vi "COD主界面（列队使用）.vi"() -> (8 "多列列表框":i32(listbox))   [LabVIEW 2016, in "斯坦道CODMn.lvlib"]
uses:
  <vilib>/Analysis/6fits.llb/Curve Fitting Criteria.ctl
  <vilib>/Utility/miscctls.llb/LVPointTypeDef.ctl
  <vilib>/Utility/config.llb/Read Key (I32).vi
  <vilib>/Utility/config.llb/Read Key (Double).vi
  <vilib>/Utility/config.llb/Read Key (Boolean).vi
  <vilib>/Utility/config.llb/Write Key (Double).vi
  <vilib>/Utility/config.llb/Write Key (Boolean).vi
  <vilib>/Utility/config.llb/Write Key (I32).vi
  <vilib>/Waveform/WDTFileIO.llb/Read Waveform from File.vi
  <vilib>/ptbypt/NI_PtbyPt.lvlib
  <vilib>/Utility/config.llb/NI_LVConfig.lvlib
  <vilib>/Analysis/NI_AALPro.lvlib
panel:
  in  "常规版/认证版":enum16{"常规版", "认证版"}(ring)
  in  "释放串口":bool
  in  "打开串口":bool
  in  "保存参数":dbl[](array[numeric])
  out "报警数字":i16
  out "CODMn工作状态":T1(ring)
  out "ORP-K":string
  out "ORP-B":string
  out "ORP-A":string
  out "x = y?":bool
  out "稀释倍数解释":string
  in  "CODMn跨度量程选择":enum32{"H", "L", "AUTO"}(ring)=enum."AUTO"
  in  "跨度液浓度":dbl
  in  "水样":dbl
  in  "蒸馏水":dbl
  in  "标液":dbl
  in  "质控样":dbl
  in  "加标回收":dbl
  in  "草酸钠":dbl
  in  "高锰酸钾":dbl
  in  "硫酸":dbl
  out "量程解释说明":string
  in  "高切低阈值:":dbl
  in  "低切高阈值:":dbl
  in  "自动切换量程:":enum16{"关闭", "自动切换测一次", "自动切换测两次"}(ring)
  in  "修正系数":dbl
  in  "标准液浓度":dbl
  in  "温度":dbl
  in  "恒温时间":dbl
  in  "基本量程":enum16{"L", "H"}(ring)
  in  "CODMn零点核查选择":enum16{"零点核查走纯水管", "零点核查走质控管"}(ring)
  in  "锁定按钮":bool
  in  "低量程稀释倍数:":i8=1
  out "切换量程连续测两次":bool
  in  "高量程稀释倍数:":i8=2
  in  "一键写入":bool
  in  "测量模式(公式)":u16(ring)=1 items=["水样测试"=1, "标样核查"=2, "零点核查"=3, "跨度核查"=4, "空白测试"=5, "平行样"=6, "加标回收"=7]
  out "基本量程(显示)":string
  out "测量模式(显示)":string
  in  "量程切换次数":u8
  out "数据时间":string
  out "断电排液标记":bool
  out "COM":string
  in  "启用5":bool
  in  "校准5":bool
  in  "泵滴定数5":dbl
  in  "浓度5":dbl
  in  "启用4":bool
  in  "校准4":bool
  in  "泵滴定数4":dbl
  in  "浓度4":dbl
  out "波形时间":timestamp
  in  "历史波形":bool
  out "滴定数-ORP值":u16[](array[numeric]) caption="数组"
  in  "关闭 3":bool
  in  "滴定曲线":bool
  out "ORP滴定曲线":u16[](graph)
  out "空白测试标记":bool
  out "跨度核查标记":bool
  out "启动选择 2":u16(ring) items=["水样测试", "标样核查", "零点核查", "跨度核查", "空白测试", "加标回收", "平行样", "校零", "校标"]
  in  "量程选择":enum16{"低量程", "高量程", "0-2量程"}(ring)
  in  "手动控制":bool
  in  "选用水样":enum16{"葡萄糖", "草酸钠"}(ring)
  in  "方程系数":cluster{"X":dbl, "b":dbl, "X^2":dbl} {"X^2" format="%#.6g"; "b" format="%#.6g"; "X" format="%#.6g"}
  out "多项式系数1":dbl[](array[numeric]) caption="多项式系数"
  out "XY图":cluster{"X Values":dbl[], "Y Values":dbl[]}[](graph)
  in  "模型":enum32{"线性", "多项式"}(ring)
  out "启动时间":timestamp format="%<%Y/%m/%d %H:%M:%S>T"
  in  "关闭 2":bool
  out "r^2":dbl format="%.8g"
  out "拟合公式":string
  out "b":dbl format="%#.4g"
  out "K":dbl format="%#.4f"
  out "当前校准":i32
  in  "启用3":bool
  in  "启用2":bool
  in  "启用1":bool
  in  "校准3":bool
  in  "校准2":bool
  in  "校准1":bool
  in  "泵滴定数3":dbl
  in  "泵滴定数2":dbl
  in  "泵滴定数1":dbl
  in  "浓度3":dbl
  in  "浓度2":dbl
  in  "浓度1":dbl
  in  "写入":bool
  out "测量模式数字":i32
  out "零点核查标记":bool
  out "排液故障":bool
  out "进水样超量程":bool
  out "标样核查标记":bool
  out "平行样测量":bool
  out "加标回收测量":bool
  out "质控样测量":bool
  out "待机":bool
  out "校标错误":bool
  out "校零错误":bool
  out "测量错误":bool
  out "草酸钠报警":bool
  out "高锰酸钾报警":bool
  out "加热故障":bool
  out "温控器故障":bool
  out "ORP故障":bool
  out "排液标记":bool
  out "故障标记":bool
  out "校标标记":bool
  out "校零标记":bool
  out "通讯状态":bool
  out "水样测量":bool
  in  "读取":bool
  in  "返回":bool
  in  "校准配置":bool
  in  "零点泵计量数 2":dbl
  in  "标度泵计量数 2":dbl
  out "标度滴定值":dbl
  out "零点滴定值":dbl
  in  "保存":bool
  in  "关闭":bool
  out "测量数据区":T2 {"单位" items=["ug/L", "mg/L", "ppm", "mg/m3", "cm", "ppb", "ug/m3", "%", "nmol/mol", "umol/mol", "MPN/L", "MPN/100ml", "ng/m3", "NTU", "无量纲", "ms/cm", "us/cm", "℃", "mV", "万个/L"]}
  out "仪器时间":timestamp format="%<%Y/%m/%d %H:%M:%S>T"
  out "秒":u16
  out "分":u16
  out "COD浓度（mg/L)":dbl format="%.2g"
  out "进样管":dbl
  out "高锰酸钾":dbl
  out "草酸钠":dbl
  out "硫酸":dbl
  out "ORP显示":dbl
  out "温度":dbl
  out "加热":bool
  out "搅拌":bool
  out "进硫酸":bool
  out "进加标回收样":bool
  out "进质控样":bool
  out "进标液":bool
  out "进蒸馏水":bool
  out "进水样":bool
  out "进草酸钠":bool
  out "进高锰酸钾":bool
  out "定时启动":bool
  in  "启动":bool
  in  "故障清除":bool
  in  "参数配置":bool
  in  "停止":bool
  in  "单步启动":bool
  out "系统时间":timestamp
  in  "时间校准":bool
  out "报警簇":T3
  out "模式（受控）":u16
  # "测量时间："
  # "(水样~加标回收)"
  # "mV"
  # "℃"
  # "注：遇到加热故障和排液故障时仪器不能正常启动，\n必须排查故障并点击报警清除按钮方可运行。"
  # "mg/L"
  # "泵计量参数设置"
  # "基本参数设置"
  # "校零校标结果"
  # "校零结果："
  # "校零滴定值："
  # "加热恒温温度(℃):"
  # "水样："
  # "高锰酸钾："
  # "校标结果："
  # "标度滴定值："
  # "恒温时间(分钟):"
  # "草酸钠："
  # "蒸馏水："
  # "零点泵计量值："
  # "标准液浓度(mg/L):"
  # "硫酸："
  # "标液："
  # "标度泵计量值："
  # "修正系数："
  # "跨度液浓度："
  # "质控样:"
  # "基本量程(L、H)可选:"
  # "跨度量程选择："
  # "加标回收样："
  # "是否启用"
  # "泵滴定数"
  # "浓度"
  # "辅\n助\n计\n算\n区"
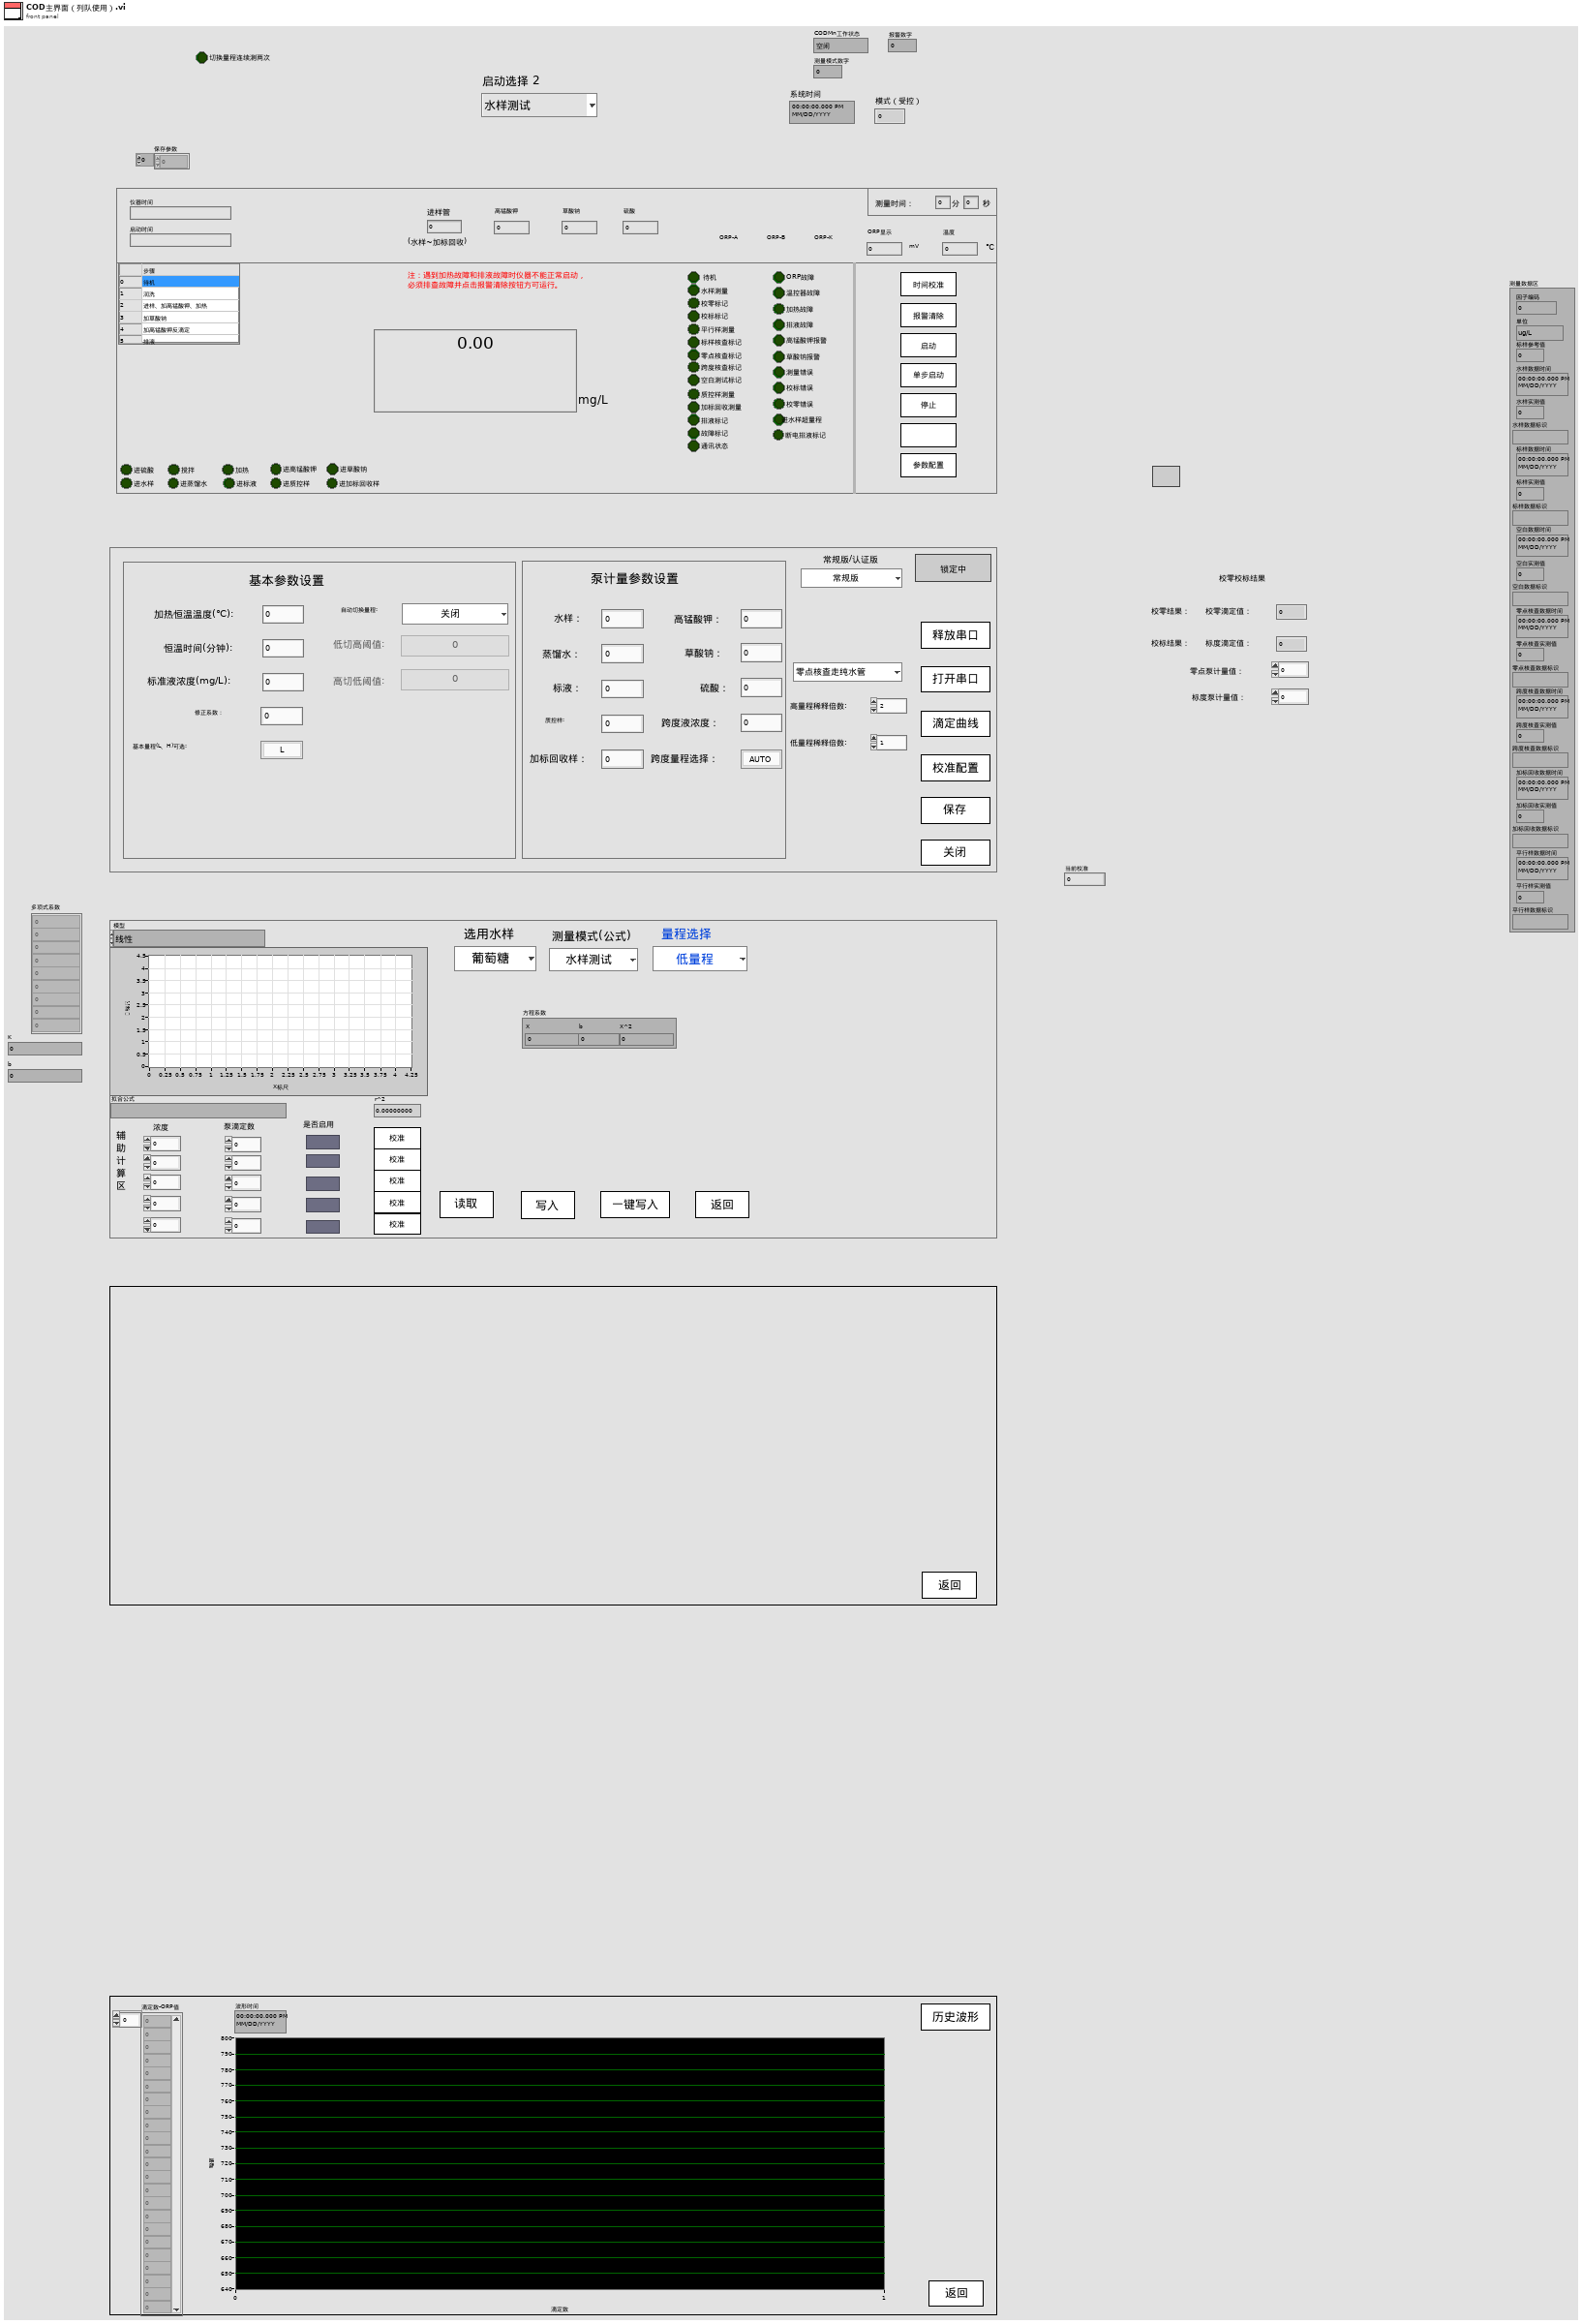
[diagram p1: front panel]
types:
  T1 = enum16{"空闲", "水样测试", "标样核查", "零点核查", "跨度核查", "空白测试", "平行样测试", "质控样", "空白校准", "标样校准", "加标回收"}
  T2 = cluster{"因子编码":u32, "单位":u16, "标样参考值":sgl, "水样数据时间":timestamp, "水样实测值":sgl, "水样数据标识":string, "标样数据时间":timestamp, "标样实测值":sgl, "标样数据标识":string, "空白数据时间":timestamp, "空白实测值":sgl, "空白数据标识":string, "零点核查数据时间":timestamp, "零点核查实测值":sgl, "零点核查数据标识":string, "跨度核查数据时间":timestamp, "跨度核查实测值":sgl, "跨度核查数据标识":string, "加标回收数据时间":timestamp, "加标回收实测值":sgl, "加标回收数据标识":string, "平行样数据时间":timestamp, "平行样实测值":sgl, "平行样数据标识":string}
  T3 = cluster{"ORP故障":bool, "温控器故障":bool, "加热故障":bool, "高锰酸钾报警":bool, "草酸钠报警":bool, "测量错误":bool, "校零错误":bool, "校标错误":bool, " 进水样超量程":bool, "排液阀故障":bool}
  T4 = cluster{"时间":timestamp, "测量模式":string, "数据类型":string, "检测值":sgl, "单位":string, "数据标识":string, "因子编码":string, "标样参考值":sgl, "ORP-A":sgl, "ORP-B":sgl, "ORP-K":sgl, "COD滴定值":sgl, "高锰酸钾滴定数":sgl, "温度":sgl, "量程":sgl}
  T5 = enum8{"Enabled", "Disabled", "Disabled and Grayed Out"}
  T6 = typedef "NI_AALPro.lvlib/Curve Fitting Criteria.ctl" = u16
  T7 = cluster{"数组 2[0]":sgl, "数组 2[1]":sgl, "数组 2[2]":sgl, "数组 2[3]":sgl, "数组 2[4]":sgl, "数组 2[5]":sgl, "数组 2[6]":sgl, "数组 2[7]":sgl, "数组 2[8]":sgl, "数组 2[9]":sgl, "数组 2[10]":sgl, "数组 2[11]":sgl, "数组 2[12]":sgl, "数组 2[13]":sgl, "数组 2[14]":sgl, "数组 2[15]":sgl, "数组 2[16]":sgl, "数组 2[17]":sgl, "数组 2[18]":sgl, "数组 2[19]":sgl, "数组 2[20]":sgl, "数组 2[21]":sgl, "数组 2[22]":sgl, "数组 2[23]":sgl, "数组 2[24]":sgl, "数组 2[25]":sgl, "数组 2[26]":sgl, "数组 2[27]":sgl, "数组 2[28]":sgl, "数组 2[29]":sgl, "数组 2[30]":sgl, "数组 2[31]":sgl, "数组 2[32]":sgl, "数组 2[33]":sgl, "数组 2[34]":sgl, "数组 2[35]":sgl, "数组 2[36]":sgl, "数组 2[37]":sgl, "数组 2[38]":sgl, "数组 2[39]":sgl, "数组 2[40]":sgl, "数组 2[41]":sgl}
  T8 = cluster{"测量模式":enum16{"水样测量", "标样核查", "零点核查", "跨度核查", "空白测试", "加标回收", "平行样", "校零", "校标"}}
  T9 = cluster{"仪器测试类型":enum16{"水样测试", "标样核查", "空白测试", "跨度核查"}, "周期设置类型":enum16{"定点启动", "间隔启动"}, "定时功能启用":bool, "定时间隔":dbl, "24H周期设置":bool[]}
  T10 = typedef "LVDateTimeRec.ctl" = cluster{"秒数的小数部分":dbl, "秒":i32, "分":i32, "时":i32, "日":i32, "月":i32, "年":i32, "天数（周）":i32, "天数（年）":i32, "DST":i32}
  T11 = cluster{"时间标识":timestamp, "设备":string, "日志信息":string}
  T12 = cluster{"时间标识":timestamp, "参数":string, "日志信息":string, "流程参数":string}
  T13 = cluster{"时间标识":timestamp, "设备":string, "日志信息":string, "流程参数":string}
  T14 = typedef "NI_LVConfig.lvlib/Config Data RefNum.ctl" = refnum<k1>
  T15 = typedef "LVPointTypeDef.ctl" = cluster{"Horizontal":i16, "Vertical":i16}
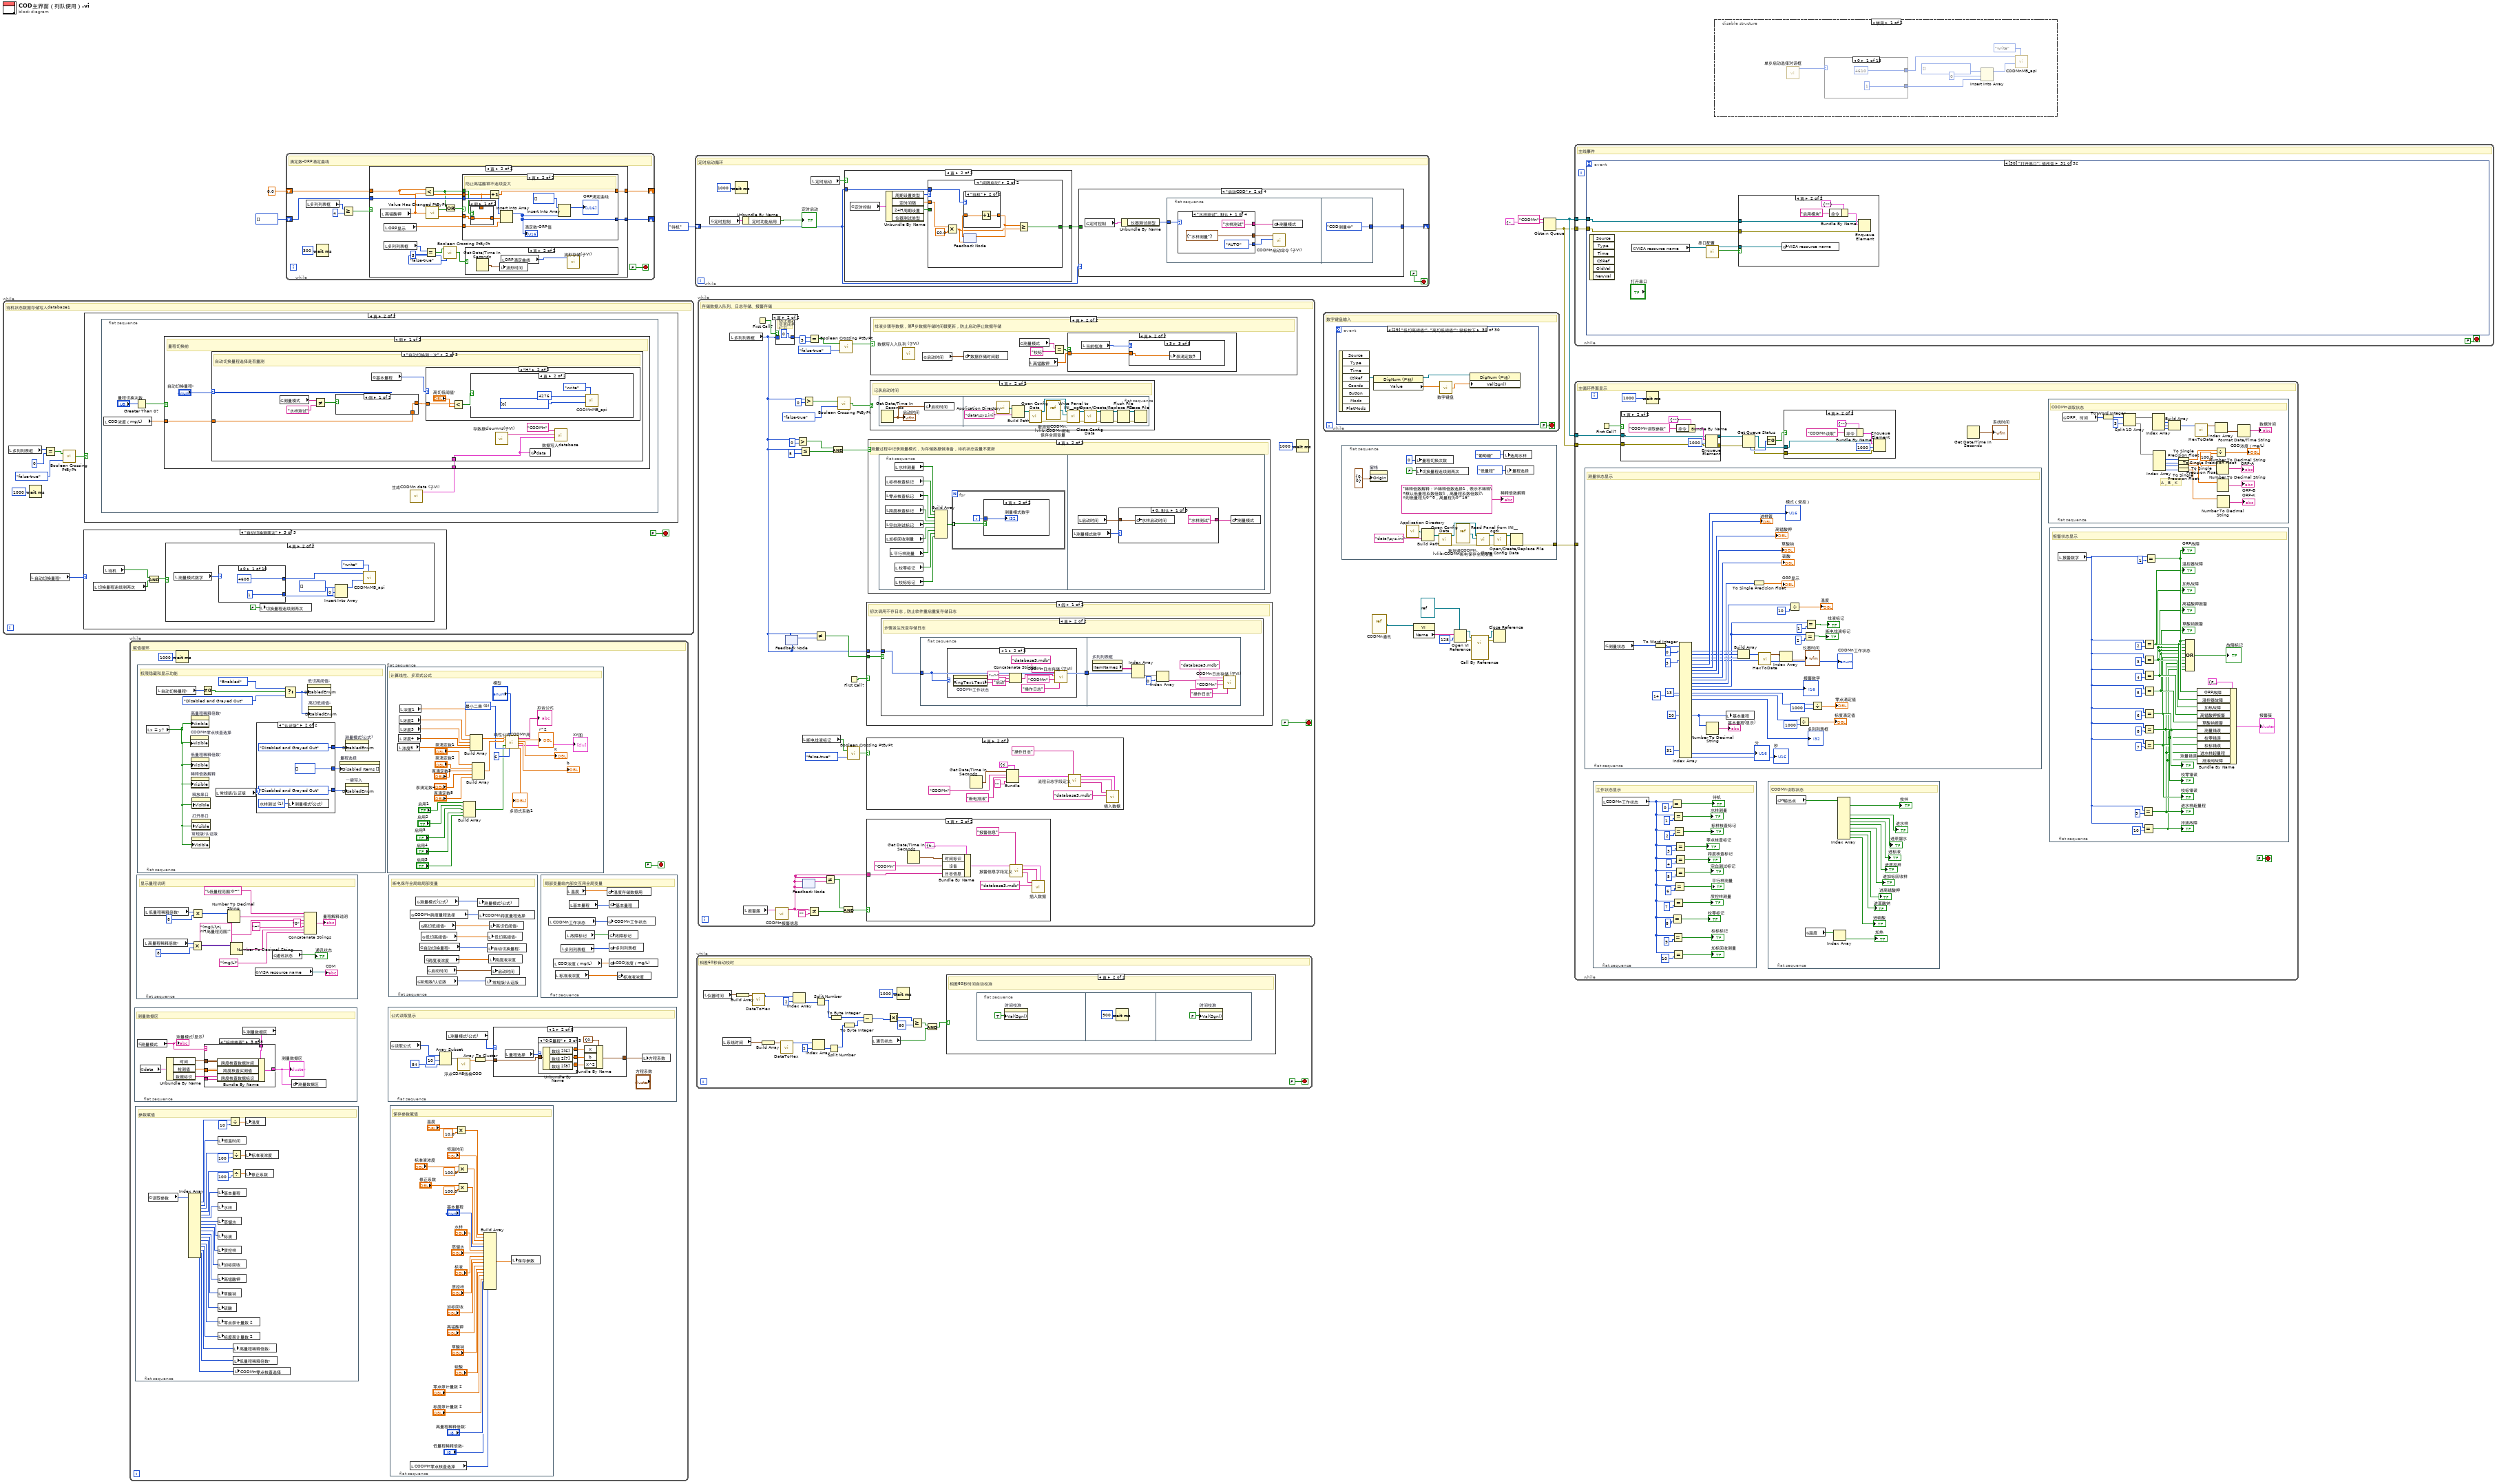
[diagram p0: block diagram]
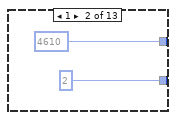
[diagram p2: hidden frame]
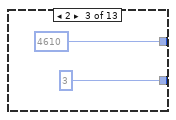
[diagram p3: hidden frame]
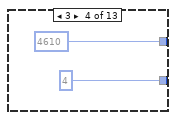
[diagram p4: hidden frame]
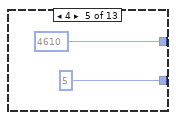
[diagram p5: hidden frame]
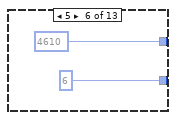
[diagram p6: hidden frame]
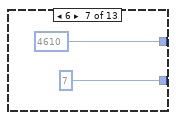
[diagram p7: hidden frame]
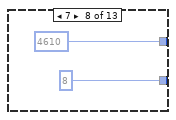
[diagram p8: hidden frame]
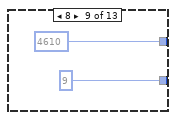
[diagram p9: hidden frame]
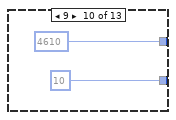
[diagram p10: hidden frame]
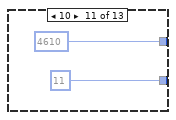
[diagram p11: hidden frame]
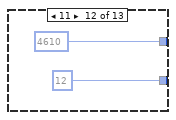
[diagram p12: hidden frame]
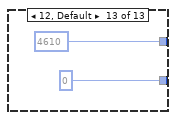
[diagram p13: hidden frame]
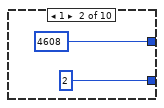
[diagram p19: hidden frame]
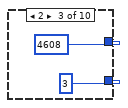
[diagram p20: hidden frame]
diagram:
  n1 = while {
    stop <- FALSE stop-if-true
    # "待机状态数据存储写入database1"
    n2 = local read "多列列表框"() -> (w22:i32)
    n3 = Wait (ms)(milliseconds to wait=u32 1000 ("等待时间（毫秒）")) -> ()  [unwired: 1 out]
    n4 = local read "自动切换量程:"() -> (w17:enum16{"关闭", "自动切换测一次", "自动切换测两次"})
    n5 = Equal?(x=w22, y=0) -> (x = y?=w20:bool)
    n6 = call <vilib>:"Boolean Crossing PtByPt.vi"("direction"=enum16{"either", "false-true", "true-false"}."false-true", "input"=w20) -> ("crossing"=w18:bool)  [unwired: 1 in]
    n7 = case shown="\"自动切换测两次\"" w17 {
      frame "关闭", Default {
      }
      frame "自动切换测一次" {
      }
      frame "自动切换测两次" {
        n8 = local read "切换量程连续测两次"() -> (w26:bool)
        n9 = local read "待机"() -> (w27:bool)
        n10 = Compound Arithmetic op=AND ("复合运算")(w27, w26) -> (w25:bool)
        n11 = case shown="真" w25 {
          frame False {
          }
          frame True {
            n12 = local read "测量模式数字"() -> (w32:i32)
            n13 = case shown="0" w32 {
              tunnel: [u16 4608 ("address") u16 4608 ("address") u16 4608 ("address") u16 4608 ("address") u16 4608 ("address") u16 4608 ("address") u16 4608 ("address") u16 4608 ("address") u16 4608 ("address") u16 4608 ("address")] -> w28
              tunnel: [u16 1 ("address") u16 2 ("address") u16 3 ("address") u16 4 ("address") u16 5 ("address") u16 7 ("address") u16 6 ("address") u16 8 ("address") u16 9 ("address") u16 0 ("address")] -> w35
              frame 0 {
              }
              frame 1 {
              }
              frame 2 {
              }
              frame 3 {
              }
              frame 4 {
              }
              frame 5 {
              }
              frame 6 {
              }
              frame 7 {
              }
              frame 8 {
              }
              frame 9, Default {
              }
            }
            n14 = local write "切换量程连续测两次"(FALSE ("切换量程连续测两次")) -> ()
            n15 = Insert Into Array(array=u16[] [] ("values"), index=0 ("索引"), new element=w35) -> (w29:u16[])
            n16 = call "CODMnMB_api.vi"("STEP"=enum16{"open", "read", "write", "close"}."write", "values"=w29, "starting address"=w28) -> ()  [unwired: 5 in, 4 out]
          }
        }
      }
    }
    n17 = case shown="真" w18 {
      frame False {
      }
      frame True {
        n18 = flat-sequence {
          frame #0 {
            n19 = local read "COD浓度（mg/L)"() -> (w56:dbl)
            n20 = Greater Than 0?(x="量程切换次数") -> (x > 0?=w57:bool)
            n21 = call "生成CODMn data (子VI).vi"() -> ("data"=w59:T4)  [unwired: 11 in]
            n22 = case shown="假" w57 {
              tunnel: w59 -> [w61 w116]
              tunnel: w56 -> [w60 _]
              frame False {
                # "量程切换前"
                n23 = case shown="\"自动切换测一次\"" "自动切换量程:" {
                  tunnel: w61 -> [w63 w68 w92]
                  tunnel: w60 -> [_ w66 w90]
                  frame "关闭", Default {
                    # "关闭自动切换量程"
                    n24 = call "存数据cloumns(子VI).vi"() -> ("数组"=w65:string[])  [unwired: 11 in]
                    n25 = global write "COD读取DATA全局.vi" "data"(w63) -> ()
                    n26 = call "数据写入database.vi"("data"=w63, "columns"=w65, "table"="CODMn") -> ()  [unwired: 8 in, 1 out]
                  }
                  frame "自动切换测一次" {
                    # "自动切换量程选择是否重测"
                    n27 = global read "COD测量模式全局.vi" "测量模式"() -> (w74:string)
                    n28 = Not Equal?(x=w74, y="水样测试") -> (x != y?=w72:bool)
                    n29 = case shown="假" w72 {
                      tunnel: [w75 w76] -> w71
                      tunnel: w66 -> [w75 _]
                      frame False {
                      }
                      frame True {
                        n30 = global read "COD读取DATA全局.vi" "测量数据区"() -> (w77:T2)
                        n31 = Unbundle By Name(w77) -> ("水样实测值"=w76:sgl)
                      }
                    }
                    n32 = global read "COD浓度全局变量.vi" "基本量程"() -> (w67:enum16{"L", "H"})
                    n33 = case shown="\"H\"" w67 {
                      tunnel: w71 -> [w78 w84]
                      frame "L", Default {
                        n34 = Greater?(x=w78, y="低切高阈值:") -> (0:w79:bool)
                        n35 = case shown="假" w79 {
                          frame False {
                          }
                          frame True {
                            n36 = call "CODMnMB_api.vi"("STEP"=enum16{"open", "read", "write", "close"}."write", "values"=u16[] [1], "starting address"=u16 4276) -> ()  [unwired: 5 in, 4 out]
                          }
                        }
                      }
                      frame "H" {
                        n37 = Less?(x=w84, y="高切低阈值:") -> (x < y?=w85:bool)
                        n38 = case shown="真" w85 {
                          frame False {
                          }
                          frame True {
                            n39 = call "CODMnMB_api.vi"("STEP"=enum16{"open", "read", "write", "close"}."write", "values"=u16[] [0], "starting address"=u16 4276) -> ()  [unwired: 5 in, 4 out]
                          }
                        }
                      }
                    }
                    n40 = call "存数据cloumns(子VI).vi"() -> ("数组"=w70:string[])  [unwired: 11 in]
                    n41 = global write "COD读取DATA全局.vi" "data"(w68) -> ()
                    n42 = call "数据写入database.vi"("data"=w68, "columns"=w70, "table"="CODMn") -> ()  [unwired: 8 in, 1 out]
                  }
                  frame "自动切换测两次" {
                    # "自动切换量程选择是否重测"
                    n43 = global read "COD浓度全局变量.vi" "基本量程"() -> (w91:enum16{"L", "H"})
                    n44 = case shown="\"L\", 默认" w91 {
                      tunnel: w90 -> [w94 w105]
                      tunnel: w92 -> [w93 w104]
                      frame "L", Default {
                        n45 = local read "低切高阈值:"() -> (w95:dbl)
                        n46 = Greater?(x=w94, y=w95) -> (0:w96:bool)
                        n47 = case shown="假" w96 {
                          tunnel: w93 -> [w97 _]
                          frame False {
                            n48 = call "存数据cloumns(子VI).vi"() -> ("数组"=w99:string[])  [unwired: 11 in]
                            n49 = global write "COD读取DATA全局.vi" "data"(w97) -> ()
                            n50 = call "数据写入database.vi"("data"=w97, "columns"=w99, "table"="CODMn") -> ()  [unwired: 8 in, 1 out]
                          }
                          frame True {
                            n51 = call "CODMnMB_api.vi"("STEP"=enum16{"open", "read", "write", "close"}."write", "values"=u16[] [1], "starting address"=u16 4276) -> ()  [unwired: 5 in, 4 out]
                            "切换量程连续测两次" <- TRUE ("切换量程连续测两次")
                          }
                        }
                      }
                      frame "H" {
                        n52 = local read "高切低阈值:"() -> (w106:dbl)
                        n53 = Less?(x=w105, y=w106) -> (x < y?=w107:bool)
                        n54 = case shown="真" w107 {
                          tunnel: w104 -> [w108 _]
                          frame False {
                            n55 = call "存数据cloumns(子VI).vi"() -> ("数组"=w110:string[])  [unwired: 11 in]
                            n56 = global write "COD读取DATA全局.vi" "data"(w108) -> ()
                            n57 = call "数据写入database.vi"("data"=w108, "columns"=w110, "table"="CODMn") -> ()  [unwired: 8 in, 1 out]
                          }
                          frame True {
                            # "重测第一次不存数据"
                            n58 = call "CODMnMB_api.vi"("STEP"=enum16{"open", "read", "write", "close"}."write", "values"=u16[] [0], "starting address"=u16 4276) -> ()  [unwired: 5 in, 4 out]
                            n59 = local write "切换量程连续测两次"(TRUE ("切换量程连续测两次")) -> ()
                          }
                        }
                      }
                    }
                  }
                }
              }
              frame True {
                # "防止无限切量程"
                n60 = local write "量程切换次数"(u8 0 ("量程切换次数")) -> ()
                n61 = call "存数据cloumns(子VI).vi"() -> ("数组"=w118:string[])  [unwired: 11 in]
                n62 = call "数据写入database.vi"("data"=w116, "columns"=w118, "table"="CODMn") -> ()  [unwired: 8 in, 1 out]
                n63 = global write "COD读取DATA全局.vi" "data"(w116) -> ()
              }
            }
          }
        }
      }
    }
  }
  n64 = while {
    stop <- FALSE stop-if-true
    # "赋值循环"
    n65 = flat-sequence {
      frame #0 {
        # "测量数据区"
        n66 = global read "COD测量模式全局.vi" "测量模式"() -> (w347:string)
        "测量模式(显示)" <- w347
        n67 = global read "COD读取DATA全局.vi" "data"() -> (w352:T4)
        n68 = Unbundle By Name(w352) -> ("时间"=w351:timestamp, "检测值"=w350:sgl, "数据标识"=w349:string)
        n69 = local read "测量数据区"() -> (w353:T2)
        n70 = case shown="\"标样核查\"" w347 {
          tunnel: w353 -> [w354 w359 w364 w369 w374 w379 w384 w389]
          tunnel: [w354 w358 w360 w368 w373 w378 w380 w388] -> w348
          tunnel: w351 -> [_ w357 w363 w367 w372 w377 w383 w387]
          tunnel: w350 -> [_ w356 w362 w366 w371 w376 w382 w386]
          tunnel: w349 -> [_ w355 w361 w365 w370 w375 w381 w385]
          frame "", Default {
          }
          frame "水样测试" {
            n71 = Bundle By Name(cluster=w359, "水样数据时间"=w357, "水样实测值"=w356, "水样数据标识"=w355) -> (w358:T2)
          }
          frame "标样核查" {
            n72 = Bundle By Name(cluster=w364, "跨度核查数据时间"=w363, "跨度核查实测值"=w362, "跨度核查数据标识"=w361) -> (w360:T2)
          }
          frame "零点核查" {
            n73 = Bundle By Name(cluster=w369, "零点核查数据时间"=w367, "零点核查实测值"=w366, "零点核查数据标识"=w365) -> (w368:T2)
          }
          frame "加标回收" {
            n74 = Bundle By Name(cluster=w374, "加标回收数据时间"=w372, "加标回收实测值"=w371, "加标回收数据标识"=w370) -> (w373:T2)
          }
          frame "平行样" {
            n75 = Bundle By Name(cluster=w379, "平行样数据时间"=w377, "平行样实测值"=w376, "平行样数据标识"=w375) -> (w378:T2)
          }
          frame "校零" {
            n76 = Bundle By Name(cluster=w384, "空白数据时间"=w383, "空白实测值"=w382, "空白数据标识"=w381) -> (w380:T2)
          }
          frame "校标" {
            n77 = Bundle By Name(cluster=w389, "标样数据时间"=w387, "标样实测值"=w386, "标样数据标识"=w385) -> (w388:T2)
          }
        }
        "测量数据区" <- w348
        n78 = global write "COD读取DATA全局.vi" "测量数据区"(w348) -> ()
      }
    }
    n79 = flat-sequence {
      frame #0 {
        # "参数赋值"
        n80 = global read "COD读取DATA全局.vi" "读取参数"() -> (w153:u16[])
        n81 = Index Array(array=w153) -> (element #1=w165:u16, element #2=w177:u16, element #3=w158:u16, element #4=w163:u16, element #5=w161:u16, element #6=w160:u16, element #7=w176:u16, element #8=w175:u16, element #9=w174:u16, element #10=w173:u16, element #11=w172:u16, element #12=w171:u16, element #13=w170:u16, element #14=w169:u16, element #15=w168:u16, element #16=w156:u16, element #17=w155:u16, element #18=w154:u16)  [unwired: 18 in]
        n82 = local write "恒温时间"(w177) -> ()
        n83 = local write "基本量程"(w161) -> ()
        n84 = local write "水样"(w160) -> ()
        n85 = local write "蒸馏水"(w176) -> ()
        n86 = local write "标液"(w175) -> ()
        n87 = local write "质控样"(w174) -> ()
        n88 = local write "加标回收"(w173) -> ()
        n89 = local write "高锰酸钾"(w172) -> ()
        n90 = local write "草酸钠"(w171) -> ()
        n91 = local write "硫酸"(w170) -> ()
        n92 = local write "零点泵计量数 2"(w169) -> ()
        n93 = local write "标度泵计量数 2"(w168) -> ()
        n94 = Divide(x=w165, y=u16 10) -> (x/y=w166:dbl)
        n95 = Divide(x=w158, y=u16 100) -> (x/y=w157:dbl)
        n96 = Divide(x=w163, y=u16 100) -> (x/y=w162:dbl)
        n97 = local write "高量程稀释倍数:"(w156) -> ()
        n98 = local write "低量程稀释倍数:"(w155) -> ()
        n99 = local write "CODMn零点核查选择"(w154) -> ()
        n100 = local write "温度"(w166) -> ()
        n101 = local write "标准液浓度"(w157) -> ()
        n102 = local write "修正系数"(w162) -> ()
      }
    }
    n103 = flat-sequence {
      frame #0 {
        # "显示量程说明"
        n104 = local read "高量程稀释倍数:"() -> (w401:i8)
        n105 = local read "低量程稀释倍数:"() -> (w411:i8)
        n106 = Multiply(x=w401, y=i8 8) -> (x*y=w399:i8)
        n107 = Multiply(x=w411, y=i8 8) -> (x*y=w403:i8)
        n108 = Number To Decimal String(number=w403) -> (decimal integer string=w408:string)  [unwired: 1 in]
        n109 = Number To Decimal String(number=w399) -> (decimal integer string=w406:string)  [unwired: 1 in]
        n110 = global read "CODMn断电保存全局变量.vi" "VISA resource name"() -> (→"COM":refnum<visa-resource-name>)
        n111 = global read "COD读取DATA全局.vi" "通讯状态"() -> (→"通讯状态":bool)
        n112 = Concatenate Strings("L低量程范围:0~" ("量程解释说明"), w408, "(mg/L)\n\nH高量程范围:" ("量程解释说明"), "0" ("字符串"), "~" ("量程解释说明"), w406, "(mg/L)" ("量程解释说明")) -> (→"量程解释说明":string)
      }
    }
    n113 = flat-sequence {
      frame #0 {
        # "权限隐藏和显示功能"
        n114 = local read "x = y?"() -> (w418:bool)
        n115 = local read "自动切换量程:"() -> (w420:enum16{"关闭", "自动切换测一次", "自动切换测两次"})
        n116 = property on="CODMn零点核查选择" class="Enum (严格)"("Visible"=w418) -> ()  [unwired: 2 in, 2 out]
        n117 = property on="高量程稀释倍数:" class="DigNum (严格)"("Visible"=w418) -> ()  [unwired: 2 in, 2 out]
        n118 = property on="低量程稀释倍数:" class="DigNum (严格)"("Visible"=w418) -> ()  [unwired: 2 in, 2 out]
        n119 = property on="稀释倍数解释" class="Str"("Visible"=w418) -> ()  [unwired: 2 in, 2 out]
        n120 = property on="常规版/认证版" class="Enum (严格)"("Visible"=w418) -> ()  [unwired: 2 in, 2 out]
        n121 = property on="释放串口" class="Bool"("Visible"=w418) -> ()  [unwired: 2 in, 2 out]
        n122 = property on="打开串口" class="Bool"("Visible"=w418) -> ()  [unwired: 2 in, 2 out]
        n123 = Not Equal To 0?(x=w420) -> (x != 0?=w419:bool)
        n124 = local read "常规版/认证版"() -> (w417:enum16{"常规版", "认证版"})
        n125 = case shown="\"认证版\"" w417 {
          tunnel: [T5."Enabled" ("禁用") T5."Disabled and Grayed Out" ("禁用")] -> w416
          tunnel: [i32[] [2] ("禁用项[]") i32[] [] ("禁用项[]")] -> w415
          tunnel: [T5."Enabled" ("禁用") T5."Disabled and Grayed Out" ("禁用")] -> w414
          frame "常规版", Default {
          }
          frame "认证版" {
            w427 = u16 1 items=["水样测试"=1, "标样核查"=2, "零点核查"=3, "跨度核查"=4, "空白测试"=5, "平行样"=6, "加标回收"=7] ("测量模式(公式)")
            n126 = local write "测量模式(公式)"(w427) -> ()
          }
        }
        n127 = Select(t=T5."Enabled" ("禁用"), s=w419, f=T5."Disabled and Grayed Out" ("禁用")) -> (s? t:f=w421:T5)
        n128 = property on="低切高阈值:" class="DigNum (严格)"("DisabledEnum"=w421) -> ()  [unwired: 2 in, 2 out]
        n129 = property on="高切低阈值:" class="DigNum (严格)"("DisabledEnum"=w421) -> ()  [unwired: 2 in, 2 out]
        n130 = property on="量程选择" class="Enum (严格)"("Disabled Items []"=w415) -> ()  [unwired: 2 in, 2 out]
        n131 = property on="测量模式(公式)" class="Ring (严格)"("DisabledEnum"=w416) -> ()  [unwired: 2 in, 2 out]
        n132 = property on="一键写入" class="Bool (严格)"("DisabledEnum"=w414) -> ()  [unwired: 2 in, 2 out]
      }
    }
    n133 = Wait (ms)(milliseconds to wait=u32 1000 ("等待时间（毫秒）")) -> ()  [unwired: 1 out]
    n134 = flat-sequence {
      frame #0 {
        w340 = T6 0 items=["最小二乘", "最小绝对残差", "Bisquare"] ("method")
        # "计算线性、多项式公式"
        n135 = local read "浓度5"() -> (w331:dbl)
        n136 = local read "浓度4"() -> (w332:dbl)
        n137 = local read "浓度2"() -> (w345:dbl)
        n138 = local read "浓度3"() -> (w346:dbl)
        n139 = local read "浓度1"() -> (w344:dbl)
        n140 = Build Array("启用1", "启用2", "启用3", "启用4", "启用5") -> (w325:bool[])
        n141 = Build Array(w344, w345, w346, w332, w331) -> (w342:dbl[])
        n142 = Build Array("泵滴定数1", "泵滴定数2", "泵滴定数3", "泵滴定数4", "泵滴定数5") -> (w341:dbl[])
        n143 = call "线性公式CODMn用.vi"("标液浓度"=w342, "监测浓度"=w341, "启用"=w325, "method"=w340, "模型"="模型", "精度"=6) -> ("拟合方程"=→"拟合公式":string, "r^2"=→"r^2":dbl, "slope"=→"K":dbl, "intercept"=→"b":dbl, "XY图"=→"XY图":cluster{"X Values":dbl[], "Y Values":dbl[]}[], "Polynomial Coefficients"=→"多项式系数1":dbl[])  [unwired: 8 in]
      }
    }
    n144 = flat-sequence {
      frame #0 {
        # "公式读取显示"
        n145 = global read "COD读取DATA全局.vi" "读取公式"() -> (w185:u16[])
        n146 = Array Subset(array=w185, index=10 ("索引"), length=84 ("长度")) -> (w180:u16[])
        n147 = local read "测量模式(公式)"() -> (w183:u16)
        n148 = call "浮点CDAB转换COD.vi"("数组"=w180) -> ("数组 2"=w181:sgl[])  [unwired: 10 in]
        n149 = Array To Cluster(array=w181) -> (cluster=w184:T7)
        n150 = case shown="1" w183 {
          tunnel: [cluster{"X":dbl, "b":dbl, "X^2":dbl} {"X"=999.0, "b"=999.0, "X^2"=999.0} ("方程系数") w188 w207 w226 w245 w264 w283 w302] -> w182
          tunnel: w184 -> [_ w187 w206 w225 w244 w263 w282 w301]
          frame 0, Default {
          }
          frame 1 {
            n151 = local read "量程选择"() -> (w190:enum16{"低量程", "高量程", "0-2量程"})
            n152 = case shown="\"0-2量程\"" w190 {
              tunnel: w187 -> [w197 w201 w205]
              tunnel: [w196 w200 w204] -> w193
              tunnel: [w195 w199 w203] -> w192
              tunnel: [w194 w198 w202] -> w191
              frame "低量程", Default {
                n153 = Unbundle By Name(w197) -> ("数组 2[0]"=w196:sgl, "数组 2[1]"=w195:sgl, "数组 2[2]"=w194:sgl)
              }
              frame "高量程" {
                n154 = Unbundle By Name(w201) -> ("数组 2[3]"=w200:sgl, "数组 2[4]"=w199:sgl, "数组 2[5]"=w198:sgl)
              }
              frame "0-2量程" {
                n155 = Unbundle By Name(w205) -> ("数组 2[6]"=w204:sgl, "数组 2[7]"=w203:sgl, "数组 2[8]"=w202:sgl)
              }
            }
            n156 = Bundle By Name(cluster=cluster{"X":dbl, "b":dbl, "X^2":dbl} {"X"=0.0, "b"=0.0, "X^2"=0.0} ("方程系数"), "X"=w193, "b"=w192, "X^2"=w191) -> (w188:cluster{"X":dbl, "b":dbl, "X^2":dbl})
          }
          frame 2 {
            n157 = local read "量程选择"() -> (w209:enum16{"低量程", "高量程", "0-2量程"})
            n158 = case shown="\"高量程\"" w209 {
              tunnel: w206 -> [w216 w220 w224]
              tunnel: [w215 w219 w223] -> w212
              tunnel: [w214 w218 w222] -> w211
              tunnel: [w213 w217 w221] -> w210
              frame "低量程", Default {
                n159 = Unbundle By Name(w216) -> ("数组 2[6]"=w215:sgl, "数组 2[7]"=w214:sgl, "数组 2[8]"=w213:sgl)
              }
              frame "高量程" {
                n160 = Unbundle By Name(w220) -> ("数组 2[9]"=w219:sgl, "数组 2[10]"=w218:sgl, "数组 2[11]"=w217:sgl)
              }
              frame "0-2量程" {
                n161 = Unbundle By Name(w224) -> ("数组 2[6]"=w223:sgl, "数组 2[7]"=w222:sgl, "数组 2[8]"=w221:sgl)
              }
            }
            n162 = Bundle By Name(cluster=cluster{"X":dbl, "b":dbl, "X^2":dbl} {"X"=0.0, "b"=0.0, "X^2"=0.0} ("方程系数"), "X"=w212, "b"=w211, "X^2"=w210) -> (w207:cluster{"X":dbl, "b":dbl, "X^2":dbl})
          }
          frame 3 {
            n163 = local read "量程选择"() -> (w228:enum16{"低量程", "高量程", "0-2量程"})
            n164 = case shown="\"高量程\"" w228 {
              tunnel: w225 -> [w235 w239 w243]
              tunnel: [w234 w238 w242] -> w231
              tunnel: [w233 w237 w241] -> w230
              tunnel: [w232 w236 w240] -> w229
              frame "低量程", Default {
                n165 = Unbundle By Name(w235) -> ("数组 2[12]"=w234:sgl, "数组 2[13]"=w233:sgl, "数组 2[14]"=w232:sgl)
              }
              frame "高量程" {
                n166 = Unbundle By Name(w239) -> ("数组 2[15]"=w238:sgl, "数组 2[16]"=w237:sgl, "数组 2[17]"=w236:sgl)
              }
              frame "0-2量程" {
                n167 = Unbundle By Name(w243) -> ("数组 2[6]"=w242:sgl, "数组 2[7]"=w241:sgl, "数组 2[8]"=w240:sgl)
              }
            }
            n168 = Bundle By Name(cluster=cluster{"X":dbl, "b":dbl, "X^2":dbl} {"X"=0.0, "b"=0.0, "X^2"=0.0} ("方程系数"), "X"=w231, "b"=w230, "X^2"=w229) -> (w226:cluster{"X":dbl, "b":dbl, "X^2":dbl})
          }
          frame 4 {
            n169 = local read "量程选择"() -> (w247:enum16{"低量程", "高量程", "0-2量程"})
            n170 = case shown="\"高量程\"" w247 {
              tunnel: w244 -> [w254 w258 w262]
              tunnel: [w253 w257 w261] -> w250
              tunnel: [w252 w256 w260] -> w249
              tunnel: [w251 w255 w259] -> w248
              frame "低量程", Default {
                n171 = Unbundle By Name(w254) -> ("数组 2[18]"=w253:sgl, "数组 2[19]"=w252:sgl, "数组 2[20]"=w251:sgl)
              }
              frame "高量程" {
                n172 = Unbundle By Name(w258) -> ("数组 2[21]"=w257:sgl, "数组 2[22]"=w256:sgl, "数组 2[23]"=w255:sgl)
              }
              frame "0-2量程" {
                n173 = Unbundle By Name(w262) -> ("数组 2[6]"=w261:sgl, "数组 2[7]"=w260:sgl, "数组 2[8]"=w259:sgl)
              }
            }
            n174 = Bundle By Name(cluster=cluster{"X":dbl, "b":dbl, "X^2":dbl} {"X"=0.0, "b"=0.0, "X^2"=0.0} ("方程系数"), "X"=w250, "b"=w249, "X^2"=w248) -> (w245:cluster{"X":dbl, "b":dbl, "X^2":dbl})
          }
          frame 5 {
            n175 = local read "量程选择"() -> (w266:enum16{"低量程", "高量程", "0-2量程"})
            n176 = case shown="\"高量程\"" w266 {
              tunnel: w263 -> [w273 w277 w281]
              tunnel: [w272 w276 w280] -> w269
              tunnel: [w271 w275 w279] -> w268
              tunnel: [w270 w274 w278] -> w267
              frame "低量程", Default {
                n177 = Unbundle By Name(w273) -> ("数组 2[24]"=w272:sgl, "数组 2[25]"=w271:sgl, "数组 2[26]"=w270:sgl)
              }
              frame "高量程" {
                n178 = Unbundle By Name(w277) -> ("数组 2[27]"=w276:sgl, "数组 2[28]"=w275:sgl, "数组 2[29]"=w274:sgl)
              }
              frame "0-2量程" {
                n179 = Unbundle By Name(w281) -> ("数组 2[6]"=w280:sgl, "数组 2[7]"=w279:sgl, "数组 2[8]"=w278:sgl)
              }
            }
            n180 = Bundle By Name(cluster=cluster{"X":dbl, "b":dbl, "X^2":dbl} {"X"=0.0, "b"=0.0, "X^2"=0.0} ("方程系数"), "X"=w269, "b"=w268, "X^2"=w267) -> (w264:cluster{"X":dbl, "b":dbl, "X^2":dbl})
          }
          frame 6 {
            n181 = local read "量程选择"() -> (w285:enum16{"低量程", "高量程", "0-2量程"})
            n182 = case shown="\"高量程\"" w285 {
              tunnel: w282 -> [w292 w296 w300]
              tunnel: [w291 w295 w299] -> w288
              tunnel: [w290 w294 w298] -> w287
              tunnel: [w289 w293 w297] -> w286
              frame "低量程", Default {
                n183 = Unbundle By Name(w292) -> ("数组 2[30]"=w291:sgl, "数组 2[31]"=w290:sgl, "数组 2[32]"=w289:sgl)
              }
              frame "高量程" {
                n184 = Unbundle By Name(w296) -> ("数组 2[33]"=w295:sgl, "数组 2[34]"=w294:sgl, "数组 2[35]"=w293:sgl)
              }
              frame "0-2量程" {
                n185 = Unbundle By Name(w300) -> ("数组 2[6]"=w299:sgl, "数组 2[7]"=w298:sgl, "数组 2[8]"=w297:sgl)
              }
            }
            n186 = Bundle By Name(cluster=cluster{"X":dbl, "b":dbl, "X^2":dbl} {"X"=0.0, "b"=0.0, "X^2"=0.0} ("方程系数"), "X"=w288, "b"=w287, "X^2"=w286) -> (w283:cluster{"X":dbl, "b":dbl, "X^2":dbl})
          }
          frame 7 {
            n187 = local read "量程选择"() -> (w304:enum16{"低量程", "高量程", "0-2量程"})
            n188 = case shown="\"高量程\"" w304 {
              tunnel: w301 -> [w311 w315 w319]
              tunnel: [w310 w314 w318] -> w307
              tunnel: [w309 w313 w317] -> w306
              tunnel: [w308 w312 w316] -> w305
              frame "低量程", Default {
                n189 = Unbundle By Name(w311) -> ("数组 2[36]"=w310:sgl, "数组 2[37]"=w309:sgl, "数组 2[38]"=w308:sgl)
              }
              frame "高量程" {
                n190 = Unbundle By Name(w315) -> ("数组 2[39]"=w314:sgl, "数组 2[40]"=w313:sgl, "数组 2[41]"=w312:sgl)
              }
              frame "0-2量程" {
                n191 = Unbundle By Name(w319) -> ("数组 2[6]"=w318:sgl, "数组 2[7]"=w317:sgl, "数组 2[8]"=w316:sgl)
              }
            }
            n192 = Bundle By Name(cluster=cluster{"X":dbl, "b":dbl, "X^2":dbl} {"X"=0.0, "b"=0.0, "X^2"=0.0} ("方程系数"), "X"=w307, "b"=w306, "X^2"=w305) -> (w302:cluster{"X":dbl, "b":dbl, "X^2":dbl})
          }
        }
        n193 = local write "方程系数"(w182) -> ()
      }
    }
    n194 = flat-sequence {
      frame #0 {
        # "断电保存全局给局部变量"
        n195 = global read "CODMn断电保存全局变量.vi" "CODMn跨度量程选择"() -> (w396:enum32{"H", "L", "AUTO"})
        n196 = global read "CODMn断电保存全局变量.vi" "测量模式(公式)"() -> (w397:u16)
        n197 = global read "CODMn断电保存全局变量.vi" "常规版/认证版"() -> (w390:enum16{"常规版", "认证版"})
        n198 = global read "CODMn断电保存全局变量.vi" "自动切换量程:"() -> (w393:enum16{"关闭", "自动切换测一次", "自动切换测两次"})
        n199 = global read "CODMn断电保存全局变量.vi" "高切低阈值:"() -> (w395:dbl)
        n200 = global read "CODMn断电保存全局变量.vi" "低切高阈值:"() -> (w394:dbl)
        n201 = global read "CODMn断电保存全局变量.vi" "跨度液浓度"() -> (w392:dbl)
        n202 = global read "CODMn断电保存全局变量.vi" "启动时间"() -> (w391:timestamp)
        n203 = local write "测量模式(公式)"(w397) -> ()
        n204 = local write "CODMn跨度量程选择"(w396) -> ()
        n205 = local write "常规版/认证版"(w390) -> ()
        n206 = local write "自动切换量程:"(w393) -> ()
        n207 = local write "低切高阈值:"(w394) -> ()
        n208 = local write "跨度液浓度"(w392) -> ()
        n209 = local write "高切低阈值:"(w395) -> ()
        n210 = local write "启动时间"(w391) -> ()
      }
    }
    n211 = flat-sequence {
      frame #0 {
        # "保存参数赋值"
        n212 = local read "CODMn零点核查选择"() -> (w122:enum16{"零点核查走纯水管", "零点核查走质控管"})
        n213 = Multiply(x="温度", y=10.0) -> (x*y=w131:dbl)
        n214 = Multiply(x="标准液浓度", y=100.0) -> (x*y=w125:dbl)
        n215 = Multiply(x="修正系数", y=100.0) -> (x*y=w128:dbl)
        n216 = Build Array(w131, "恒温时间", w125, w128, "基本量程", "水样", "蒸馏水", "标液", "质控样", "加标回收", "高锰酸钾", "草酸钠", "硫酸", "零点泵计量数 2", "标度泵计量数 2", "高量程稀释倍数:", "低量程稀释倍数:", w122) -> (w121:dbl[])
        n217 = local write "保存参数"(w121) -> ()
      }
    }
    n218 = flat-sequence {
      frame #0 {
        # "局部变量给内部交互用全局变量"
        n219 = local read "CODMn工作状态"() -> (w150:T1)
        n220 = local read "COD浓度（mg/L)"() -> (w147:dbl)
        n221 = local read "标准液浓度"() -> (w146:dbl)
        n222 = local read "多列列表框"() -> (w148:i32)
        n223 = local read "故障标记"() -> (w149:bool)
        n224 = local read "温度"() -> (w152:dbl)
        n225 = local read "基本量程"() -> (w151:enum16{"L", "H"})
        n226 = global write "COD读取DATA全局.vi" "温度存储数据用"(w152) -> ()
        n227 = global write "COD测量模式全局.vi" "CODMn工作状态"(w150) -> ()
        n228 = global write "COD读取DATA全局.vi" "故障标记"(w149) -> ()
        n229 = global write "COD浓度全局变量.vi" "基本量程"(w151) -> ()
        n230 = global write "运行时序全局变量.vi" "多列列表框"(w148) -> ()
        n231 = global write "COD浓度全局变量.vi" "COD浓度（mg/L)"(w147) -> ()
        n232 = global write "COD浓度全局变量.vi" "标准液浓度"(w146) -> ()
      }
    }
  }
  n233 = while {
    shift-right: [w436] -> _
    shift-left: u16[] [] ("ORP滴定曲线") -> [w437]
    shift-right: [w431] -> _
    shift-left: 0.0 -> [w432]
    stop <- FALSE stop-if-true
    # "滴定数-ORP滴定曲线"
    n234 = local read "多列列表框"() -> (w435:i32)
    n235 = Wait (ms)(milliseconds to wait=u32 300 ("等待时间（毫秒）")) -> ()  [unwired: 1 out]
    n236 = Greater Or Equal?(x=w435, y=4) -> (x >= y?=w433:bool)
    n237 = case shown="真" w433 {
      tunnel: w437 -> [_ w456]
      tunnel: [u16[] [] ("ORP滴定曲线") w455] -> w436
      tunnel: w432 -> [_ w444]
      tunnel: [0.0 w443] -> w431
      frame False {
      }
      frame True {
        n238 = local read "高锰酸钾"() -> (w446:dbl)
        n239 = local read "多列列表框"() -> (w451:i32)
        n240 = local read "ORP显示"() -> (w452:dbl)
        n241 = Less?(x=w444, y=w446) -> (x < y?=w442:bool)
        n242 = Equal?(x=w451, y=5) -> (x = y?=w449:bool)
        n243 = call <vilib>:"Value Has Changed PtByPt.vi"("input data point"=w446) -> ("has changed"=w454:bool, "output data point"=w453:dbl)  [unwired: 1 in]
        n244 = call <vilib>:"Boolean Crossing PtByPt.vi"("direction"=enum16{"either", "false-true", "true-false"}."false-true", "input"=w449) -> ("crossing"=w447:bool)  [unwired: 1 in]
        n245 = Or(x=w442, y=w454) -> (x .or. y?=w445:bool)
        n246 = case shown="真" w445 {
          tunnel: w456 -> [w463 w477]
          tunnel: [w462 w476] -> w455
          tunnel: w453 -> [w464 w470]
          tunnel: w452 -> [w460 w475]
          tunnel: w444 -> [w459 w472]
          tunnel: [w459 w474] -> w443
          tunnel: w442 -> [_ w473]
          frame False {
            n247 = Equal To 0?(x=w464) -> (x = 0?=w461:bool)
            n248 = case shown="真" w461 {
              tunnel: [w465 w468] -> w462
              tunnel: w463 -> [w465 _]
              tunnel: w460 -> [_ w467]
              frame False {
              }
              frame True {
                n249 = Insert Into Array(array=u16[] [] ("ORP滴定曲线"), index=0 ("索引"), new element=w467) -> (w468:u16[])
                n250 = local write "滴定数-ORP值"(w468) -> ()
              }
            }
          }
          frame True {
            # "防止高锰酸钾不连续变大"
            n251 = case shown="假" w473 {
              tunnel: w472 -> [_ w481]
              tunnel: [w480 w481] -> w471
              tunnel: w470 -> [w480 _]
              frame False {
              }
              frame True {
              }
            }
            n252 = Increment(x=w472) -> (x+1=w474:dbl)
            n253 = Insert Into Array(array=w477, index=w471, new element=w475) -> (w476:u16[])
            "滴定数-ORP值" <- w476
            n254 = Insert Into Array(array=u16[] [] ("ORP滴定曲线"), new element=w476) -> (→"ORP滴定曲线":u16[])  [unwired: 1 in]
          }
        }
        n255 = case shown="真" w447 {
          frame False {
          }
          frame True {
            n256 = Get Date/Time In Seconds() -> (seconds since 1Jan1904=w457:timestamp)
            n257 = local write "波形时间"(w457) -> ()
            n258 = local read "ORP滴定曲线"() -> (w458:u16[])
            n259 = call "波形存储(子VI).vi"("ORP滴定曲线"=w458) -> ()  [unwired: 11 in]
          }
        }
      }
    }
  }
  n260 = while {
    shift-right: [w487] -> _
    shift-left: enum16{"待机", "启动COD", "COD测量中", "延时"}."待机" -> [w486]
    stop <- FALSE stop-if-true
    # "定时启动循环"
    n261 = global read "CODMn断电保存全局变量.vi" "定时控制"() -> (w483:T9)
    n262 = Wait (ms)(milliseconds to wait=u32 1000 ("等待时间（毫秒）")) -> ()  [unwired: 1 out]
    n263 = Unbundle By Name(w483) -> ("定时功能启用"=→"定时启动":bool)
    n264 = local read "定时启动"() -> (w484:bool)
    n265 = case shown="真" w484 {
      tunnel: w486 -> [_ w527]
      tunnel: [_ w526] -> w485
      frame False {
      }
      frame True {
        n266 = global read "CODMn断电保存全局变量.vi" "定时控制"() -> (w525:T9)
        n267 = Unbundle By Name(w525) -> ("周期设置类型"=w528:enum16{"定点启动", "间隔启动"}, "定时间隔"=w529:dbl, "24H周期设置"=w530:bool[])  [unwired: 1 out]
        n268 = case shown="\"间隔启动\"" w528 {
          tunnel: w529 -> [_ w547]
          tunnel: w530 -> [w533 _]
          tunnel: w527 -> [w531 w550]
          tunnel: [w532 w545] -> w526
          frame "定点启动", Default {
            n269 = case shown="\"待机\", 默认" w531 {
              tunnel: w533 -> [w541 _]
              tunnel: [w534 _] -> w532
              frame "待机", Default {
                n270 = Get Date/Time In Seconds() -> (seconds since 1Jan1904=w543:timestamp)
                n271 = Seconds To Date/Time(time stamp (now)=w543) -> (date time rec=w542:T10)  [unwired: 1 in]
                n272 = Unbundle By Name(w542) -> ("时"=w540:i32, "分"=w538:i32, "秒"=w539:i32)
                n273 = Equal To 0?(x=w538) -> (x = 0?=w536:bool)
                n274 = Equal To 0?(x=w539) -> (x = 0?=w535:bool)
                n275 = Index Array(array=w541, index=w540) -> (element=w537:bool)
                n276 = Compound Arithmetic op=AND ("复合运算")(w537, w536, w535) -> (w534:bool)
              }
              frame "启动COD" {
              }
            }
          }
          frame "间隔启动" {
            n277 = Multiply(x=w547, y=60.0) -> (x*y=w544:dbl)
            n278 = feedback #1(w544) -> (w549:dbl)
            n279 = case shown="\"待机\"" w550 {
              tunnel: w549 -> [_ w552]
              tunnel: [_ w551] -> w548
              frame Default {
              }
              frame "待机" {
                n280 = Increment(x=w552) -> (x+1=w551:dbl)
              }
            }
            n281 = feedback-in #1(w548) -> ()
            n282 = Greater Or Equal?(x=w548, y=w544) -> (x >= y?=w545:bool)
          }
        }
      }
    }
    n283 = case shown="\"启动COD\"" w486 {
      tunnel: [w490 w496 w515 enum16{"待机", "启动COD", "COD测量中", "延时"}."待机"] -> w487
      tunnel: w485 -> [w493 _ _ _]
      frame "待机", Default {
        n284 = Select(t=enum16{"待机", "启动COD", "COD测量中", "延时"}."启动COD", s=w493, f=enum16{"待机", "启动COD", "COD测量中", "延时"}."待机") -> (s? t:f=w490:enum16{"待机", "启动COD", "COD测量中", "延时"})
      }
      frame "启动COD" {
        n285 = global read "CODMn断电保存全局变量.vi" "定时控制"() -> (w494:T9)
        n286 = Unbundle By Name(w494) -> ("仪器测试类型"=w495:enum16{"水样测试", "标样核查", "空白测试", "跨度核查"})
        n287 = flat-sequence {
          tunnel: w495 -> [w500]
          tunnel: [enum16{"待机", "启动COD", "COD测量中", "延时"}."COD测量中"] -> w496
          frame #0 {
            n288 = case shown="\"水样测试\", 默认" w500 {
              tunnel: [T8 {"测量模式"=enum."水样测量"} ("启动测量模式") T8 {"测量模式"=enum."标样核查"} ("启动测量模式") T8 {"测量模式"=enum."空白测试"} ("启动测量模式") T8 {"测量模式"=enum."跨度核查"} ("启动测量模式")] -> w499
              tunnel: ["水样测试" ("测量模式") "标样核查" ("测量模式") "空白测试" ("测量模式") "跨度核查" ("测量模式")] -> w498
              tunnel: [enum32{"H", "L", "AUTO"}."AUTO" ("CODMn跨度量程选择") w504 enum32{"H", "L", "AUTO"}."L" ("CODMn跨度量程选择") w510] -> w497
              frame "水样测试", Default {
              }
              frame "标样核查" {
                n289 = local read "CODMn跨度量程选择"() -> (w504:enum32{"H", "L", "AUTO"})
              }
              frame "空白测试" {
              }
              frame "跨度核查" {
                n290 = local read "CODMn跨度量程选择"() -> (w510:enum32{"H", "L", "AUTO"})
              }
            }
            n291 = global write "COD测量模式全局.vi" "测量模式"(w498) -> ()
            n292 = call "CODMn启动命令 (子VI).vi"("CODMn量程切换"=w497, "启动测量模式"=w499) -> ()  [unwired: 10 in]
          }
          frame #1 {
          }
        }
      }
      frame "COD测量中" {
        n293 = flat-sequence {
          tunnel: [w516] -> w514
          tunnel: [w523] -> w515
          tunnel: w514 -> [w523]
          frame #0 {
            n294 = global read "运行时序全局变量.vi" "多列列表框"() -> (w521:i32)
            n295 = Equal?(x=w521, y=0) -> (x = y?=w519:bool)
            n296 = Select(t=enum16{"待机", "启动COD", "COD测量中", "延时"}."延时", s=w519, f=enum16{"待机", "启动COD", "COD测量中", "延时"}."COD测量中") -> (s? t:f=w516:enum16{"待机", "启动COD", "COD测量中", "延时"})
          }
          frame #1 {
            n297 = Wait (ms)(milliseconds to wait=u32 5000 ("等待时间（毫秒）")) -> ()  [unwired: 1 out]
          }
        }
      }
      frame "延时" {
      }
    }
  }
  n298 = while {
    stop <- FALSE stop-if-true
    # "相差60秒自动校时"
    n299 = local read "仪器时间"() -> (w556:timestamp)
    n300 = local read "系统时间"() -> (w557:timestamp)
    n301 = Build Array(w556) -> (w555:timestamp[])
    n302 = call "DateToHex.vi"("DATE"=w555) -> ("数组"=w568:u16[])  [unwired: 10 in]
    n303 = Build Array(w557) -> (w574:timestamp[])
    n304 = call "DateToHex.vi"("DATE"=w574) -> ("数组"=w573:u16[])  [unwired: 10 in]
    n305 = Index Array(array=w568, index=2 ("索引")) -> (element=w570:u16)
    n306 = Index Array(array=w573, index=2 ("索引")) -> (element=w571:u16)
    n307 = Split Number(x=w570) -> (hi(x)=w564:u8)  [unwired: 1 out]
    n308 = Split Number(x=w571) -> (hi(x)=w567:u8)  [unwired: 1 out]
    n309 = To Byte Integer(number=w564) -> (8bit integer=w563:i8)
    n310 = To Byte Integer(number=w567) -> (8bit integer=w566:i8)
    n311 = Subtract(x=w563, y=w566) -> (x-y=w565:i8)
    n312 = local read "通讯状态"() -> (w559:bool)
    n313 = Absolute Value(x=w565) -> (abs(x)=w562:i8)
    n314 = Wait (ms)(milliseconds to wait=u32 1000 ("等待时间（毫秒）")) -> ()  [unwired: 1 out]
    n315 = Greater Or Equal?(x=w562, y=i8 60) -> (x >= y?=w560:bool)
    n316 = And(x=w560, y=w559) -> (x .and. y?=w558:bool)
    n317 = case shown="真" w558 {
      frame False {
      }
      frame True {
        # "相差60秒时间自动校准"
        n318 = flat-sequence {
          frame #0 {
            n319 = property on="时间校准" class="Bool (严格)"("Val(Sgnl)"=TRUE ("值(信号)")) -> ()  [unwired: 2 in, 2 out]
          }
          frame #1 {
            n320 = Wait (ms)(milliseconds to wait=u32 500 ("等待时间（毫秒）")) -> ()  [unwired: 1 out]
          }
          frame #2 {
            n321 = property on="时间校准" class="Bool (严格)"("Val(Sgnl)"=FALSE ("值(信号)")) -> ()  [unwired: 2 in, 2 out]
          }
        }
      }
    }
  }
  n322 = while {
    stop <- FALSE stop-if-true
    # "存储数据入队列、日志存储、报警存储"
    n323 = local read "多列列表框"() -> (w588:i32)
    n324 = local read "报警簇"() -> (w578:T3)
    n325 = First Call?() -> (First Call?: T/F=w590:bool)
    n326 = case shown="真" w590 {
      tunnel: [w630 u16 0 ("y")] -> w589
      tunnel: w588 -> [w630 _]
      frame False {
      }
      frame True {
        # "防止第5步关闭再打开"
      }
    }
    n327 = call "CODMn报警信息.vi"("报警簇"=w578) -> ("CODMN报警信息"=w579:string)  [unwired: 10 in]
    n328 = feedback #2(w588) -> (w594:i32)
    n329 = feedback-in #2(w588) -> ()
    n330 = Greater?(x=w588, y=u16 0) -> (0:w608:bool)
    n331 = Less Or Equal?(x=w588, y=u16 5) -> (x <= y?=w602:bool)
    n332 = local read "断电排液标记"() -> (w586:bool)
    n333 = feedback #3(w579) -> (w580:string)
    n334 = feedback-in #3(w579) -> ()
    n335 = Greater?(x=w588, y=u16 0) -> (0:w605:bool)
    n336 = Not Equal?(x=w579, y="") -> (x != y?=w584:bool)
    n337 = Equal?(x=w589, y=u16 5) -> (x = y?=w598:bool)
    n338 = Not Equal?(x=w588, y=w594) -> (x != y?=w595:bool)
    n339 = Not Equal?(x=w579, y=w580) -> (x != y?=w581:bool)
    n340 = And(x=w608, y=w602) -> (x .and. y?=w606:bool)
    n341 = call <vilib>:"Boolean Crossing PtByPt.vi"("direction"=enum16{"either", "false-true", "true-false"}."false-true", "input"=w605) -> ("crossing"=w591:bool)  [unwired: 1 in]
    n342 = call <vilib>:"Boolean Crossing PtByPt.vi"("direction"=enum16{"either", "false-true", "true-false"}."false-true", "input"=w598) -> ("crossing"=w600:bool)  [unwired: 1 in]
    n343 = And(x=w581, y=w584) -> (x .and. y?=w582:bool)
    n344 = call <vilib>:"Boolean Crossing PtByPt.vi"("direction"=enum16{"either", "false-true", "true-false"}."false-true", "input"=w586) -> ("crossing"=w585:bool)  [unwired: 1 in]
    n345 = First Call?() -> (First Call?: T/F=w596:bool)
    n346 = case shown="假" w596 {
      tunnel: w595 -> [w633 _]
      tunnel: w588 -> [w632 _]
      frame False {
        # "初次调用不存日志，防止软件重启重复存储日志"
        n347 = case shown="真" w633 {
          tunnel: w632 -> [_ w635]
          frame False {
          }
          frame True {
            # "步骤发生改变存储日志"
            n348 = flat-sequence {
              tunnel: w635 -> [w636]
              tunnel: [w636] -> w634
              tunnel: w634 -> [w656]
              frame #0 {
                n349 = case shown="1" w636 {
                  frame 0 {
                    n350 = global read "COD测量模式全局.vi" "测量模式"() -> (w643:string)
                    n351 = Concatenate Strings("-->", w643, "结束" ("字符串")) -> (w642:string)
                    n352 = call "CODMn日志存储 (子VI).vi"("table输入"="操作日志", "参数"="CODMn" ("table输入"), "日志信息"=w642, "database"="database3.mdb") -> ()  [unwired: 8 in]
                  }
                  frame 1 {
                    n353 = property on="CODMn工作状态" class="Enum (严格)"() -> ("RingText.Text"=w646:string)  [unwired: 2 in, 2 out]
                    n354 = Concatenate Strings("-->", w646, "启动" ("字符串")) -> (w644:string)
                    n355 = call "CODMn日志存储 (子VI).vi"("table输入"="操作日志", "参数"="CODMn" ("table输入"), "日志信息"=w644, "database"="database3.mdb") -> ()  [unwired: 8 in]
                  }
                  frame 2, Default {
                  }
                }
              }
              frame #1 {
                n356 = property on="多列列表框" class="MCListbox (严格)"() -> ("ItemNames"=w654:string[][])  [unwired: 2 in, 2 out]
                n357 = Index Array(array=w654, index (row)=w656) -> (element=w653:string[])  [unwired: 1 in]
                n358 = Index Array(array=w653, index=0 ("索引")) -> (element=w651:string)
                n359 = call "CODMn日志存储 (子VI).vi"("table输入"="操作日志", "参数"="CODMn" ("table输入"), "日志信息"=w651, "database"="database3.mdb") -> ()  [unwired: 8 in]
              }
            }
          }
        }
      }
      frame True {
      }
    }
    n360 = case shown="真" w585 {
      frame False {
      }
      frame True {
        n361 = Get Date/Time In Seconds() -> (seconds since 1Jan1904=w624:timestamp)
        n362 = Bundle(cluster=T12 {"时间标识"=timestamp(0 s since 1904-01-01), "参数"="", "日志信息"="", "流程参数"=""} ("data in"), "时间标识"=w624, "参数"="CODMn" ("table输入"), "日志信息"="断电排液", "流程参数"="" ("table输入")) -> (w622:T12)
        n363 = call "流程日志字段定义.vi"("table输入"="操作日志", "data in"=w622) -> ("table输出"=w627:string, "columns"=w628:string[], "data out"=w629:T13)  [unwired: 7 in]
        n364 = call "插入数据.vi"("data"=w629, "columns"=w628, "database"="database3.mdb", "table"=w627) -> ()  [unwired: 7 in, 1 out]
      }
    }
    n365 = case shown="真" w582 {
      tunnel: w579 -> [_ w609]
      frame False {
      }
      frame True {
        n366 = Get Date/Time In Seconds() -> (seconds since 1Jan1904=w611:timestamp)
        n367 = Bundle By Name(cluster=T11 {"时间标识"=timestamp(0 s since 1904-01-01), "设备"="", "日志信息"=""} ("data in"), "时间标识"=w611, "设备"="CODMn", "日志信息"=w609) -> (w612:T11)
        n368 = call "报警信息字段定义.vi"("table输入"="报警信息", "data in"=w612) -> ("table输出"=w616:string, "columns"=w617:string[], "data out"=w618:T11)  [unwired: 7 in]
        n369 = call "插入数据.vi"("data"=w618, "columns"=w617, "database"="database3.mdb", "table"=w616) -> ()  [unwired: 7 in, 1 out]
      }
    }
    n370 = case shown="真" w606 {
      frame False {
      }
      frame True {
        # "测量过程中记录测量模式，为存储数据做准备，待机状态变量不更新"
        n371 = flat-sequence {
          frame #0 {
            n372 = local read "标样核查标记"() -> (w682:bool)
            n373 = local read "零点核查标记"() -> (w681:bool)
            n374 = local read "跨度核查标记"() -> (w679:bool)
            n375 = local read "空白测试标记"() -> (w678:bool)
            n376 = local read "加标回收测量"() -> (w677:bool)
            n377 = local read "平行样测量"() -> (w676:bool)
            n378 = local read "水样测量"() -> (w683:bool)
            n379 = local read "校零标记"() -> (w675:bool)
            n380 = local read "校标标记"() -> (w674:bool)
            n381 = Build Array(w683, w682, w681, w679, w678, w677, w676, w675, w674) -> (w680:bool[])
            n382 = for {
              tunnel: w680 -> [w685] mode=indexing
              i -> [w684]
              n383 = case shown="真" w685 {
                tunnel: w684 -> [_ w686]
                frame False {
                }
                frame True {
                  "测量模式数字" <- w686
                }
              }
            }
          }
          frame #1 {
            n384 = local read "测量模式数字"() -> (w689:i32)
            n385 = local read "启动时间"() -> (w687:timestamp)
            n386 = case shown="0, 默认" w689 {
              tunnel: ["水样测试" ("测量模式") "标样核查" ("测量模式") "零点核查" ("测量模式") "跨度核查" ("测量模式") "空白测试" ("测量模式") "加标回收" ("测量模式") "平行样" ("测量模式") "校零" ("测量模式") "校标" ("测量模式")] -> w688
              tunnel: w687 -> [w690 _ _ _ _ w696 _ _ _]
              frame 0, Default {
                n387 = global write "COD测量模式全局.vi" "水样启动时间"(w690) -> ()
              }
              frame 1 {
              }
              frame 2 {
              }
              frame 3 {
              }
              frame 4 {
              }
              frame 5 {
                n388 = global write "COD测量模式全局.vi" "加标回收启动时间"(w696) -> ()
              }
              frame 6 {
              }
              frame 7 {
              }
              frame 8 {
              }
            }
            n389 = global write "COD测量模式全局.vi" "测量模式"(w688) -> ()
          }
        }
      }
    }
    n390 = case shown="真" w591 {
      frame False {
      }
      frame True {
        # "记录启动时间"
        n391 = flat-sequence {
          frame #0 {
            n392 = Get Date/Time In Seconds() -> (seconds since 1Jan1904=w659:timestamp)
            "启动时间" <- w659
            n393 = global write "CODMn断电保存全局变量.vi" "启动时间"(w659) -> ()
          }
          frame #1 {
            n394 = call <vilib>:"Application Directory.vi"() -> ("Application Directory"=w673:path)
            n395 = Build Path(base path=w673, name or relative path="data\\sys.ini" ("名称或相对路径")) -> (appended path=w671:path)
            n396 = call <vilib>:"Open Config Data.vi"("configuration file path"=w671) -> ("error out"=w667:errorcluster, "refnum"=w670:T14)  [unwired: 8 in, 1 out]
            n397 = vi-ref "斯坦道CODMn.lvlib:CODMn断电保存全局变量.vi"() -> (w669:refnum<vi>)
            n398 = call <userlib>:"Write Panel to INI__ogtk.vi"("error in (no error)"=w667, "VI ref"=w669, "refnum"=w670) -> ("error out"=w666:errorcluster, "refnum out"=w668:T14)  [unwired: 7 in]
            n399 = call <vilib>:"Close Config Data.vi"("error in (no error)"=w666, "refnum"=w668) -> ("error out"=w661:errorcluster, "file path"=w660:path)  [unwired: 8 in]
            n400 = Open/Create/Replace File(file path (use dialog)=w660, error in=w661) -> (refnum out=w664:refnum<file>, error out=w665:errorcluster)  [unwired: 4 in, 1 out]
            n401 = Flush File(refnum=w664, error in=w665) -> (refnum out=w663:refnum<file>, error out=w662:errorcluster)
            n402 = Close File(refnum=w663, error in=w662) -> ()  [unwired: 2 out]
          }
        }
      }
    }
    n403 = case shown="真" w600 {
      frame False {
      }
      frame True {
        # "排液步骤存数据，第5步数据存储时间戳更新，防止启动停止数据存储"
        n404 = call "数据写入入队列 (子VI).vi"() -> ()  [unwired: 12 in]
        n405 = global read "CODMn断电保存全局变量.vi" "启动时间"() -> (w705:timestamp)
        n406 = global write "COD读取DATA全局.vi" "数据存储时间戳"(w705) -> ()
        n407 = global read "COD测量模式全局.vi" "测量模式"() -> (w704:string)
        n408 = local read "高锰酸钾"() -> (w701:dbl)
        n409 = Equal?(x=w704, y="校标") -> (x = y?=w702:bool)
        n410 = case shown="真" w702 {
          tunnel: w701 -> [_ w706]
          frame False {
          }
          frame True {
            n411 = local read "当前校准"() -> (w707:i32)
            n412 = case shown="3" w707 {
              tunnel: w706 -> [w708 w709 w710 w711 w712]
              frame 1, Default {
                n413 = local write "泵滴定数1"(w708) -> ()
              }
              frame 2 {
                n414 = local write "泵滴定数2"(w709) -> ()
              }
              frame 3 {
                n415 = local write "泵滴定数3"(w710) -> ()
              }
              frame 4 {
                n416 = local write "泵滴定数4"(w711) -> ()
              }
              frame 5 {
                n417 = local write "泵滴定数5"(w712) -> ()
              }
            }
          }
        }
      }
    }
    n418 = Wait (ms)(milliseconds to wait=u32 1000 ("等待时间（毫秒）")) -> ()  [unwired: 1 out]
  }
  n419 = while {
    stop <- FALSE stop-if-true
    # "数字键盘输入"
    n420 = event shown="[29] \"低切高阈值:\", \"高切低阈值:\": 鼠标按下" {
      selector: _ -> [_ _ _ _ _ _ _ _ _ _ _ _ _ _ _ _ _ _ _ _ _ _ _ _ _ _ _ _ _ _]
      dyn-events: _ -> [_ _ _ _ _ _ _ _ _ _ _ _ _ _ _ _ _ _ _ _ _ _ _ _ _ _ _ _ _ _]
      timeout: _ -> [_ _ _ _ _ _ _ _ _ _ _ _ _ _ _ _ _ _ _ _ _ _ _ _ _ _ _ _ _ _]
      event Timeout {
        n421 = event-data() -> ()  [unwired: 1 in, 3 out]
      }
      event "温度": Mouse Down {
        n422 = event-data() -> ()  [unwired: 1 in, 8 out]
        n423 = local read "温度"() -> (w715:dbl)
        n424 = call "数字键盘.vi"("OldNumber"=w715) -> ("NewNumber"=w714:sgl)
        n425 = local write "温度"(w714) -> ()
      }
      event "恒温时间": Mouse Down {
        n426 = event-data() -> ()  [unwired: 1 in, 8 out]
        n427 = local read "恒温时间"() -> (w716:dbl)
        n428 = call "数字键盘.vi"("OldNumber"=w716) -> ("NewNumber"=w717:sgl)
        n429 = local write "恒温时间"(w717) -> ()
      }
      event "标准液浓度": Mouse Down {
        n430 = event-data() -> ()  [unwired: 1 in, 8 out]
        n431 = local read "标准液浓度"() -> (w719:dbl)
        n432 = call "数字键盘.vi"("OldNumber"=w719) -> ("NewNumber"=w718:sgl)
        n433 = local write "标准液浓度"(w718) -> ()
      }
      event "修正系数": Mouse Down {
        n434 = event-data() -> ()  [unwired: 1 in, 8 out]
        n435 = local read "修正系数"() -> (w720:dbl)
        n436 = call "数字键盘.vi"("OldNumber"=w720) -> ("NewNumber"=w721:sgl)
        n437 = local write "修正系数"(w721) -> ()
      }
      event "水样": Mouse Down {
        n438 = event-data() -> ()  [unwired: 1 in, 8 out]
        n439 = local read "水样"() -> (w722:dbl)
        n440 = call "数字键盘.vi"("OldNumber"=w722) -> ("NewNumber"=w723:sgl)
        n441 = local write "水样"(w723) -> ()
      }
      event "蒸馏水": Mouse Down {
        n442 = event-data() -> ()  [unwired: 1 in, 8 out]
        n443 = local read "蒸馏水"() -> (w724:dbl)
        n444 = call "数字键盘.vi"("OldNumber"=w724) -> ("NewNumber"=w725:sgl)
        n445 = local write "蒸馏水"(w725) -> ()
      }
      event "标液": Mouse Down {
        n446 = event-data() -> ()  [unwired: 1 in, 8 out]
        n447 = local read "标液"() -> (w726:dbl)
        n448 = call "数字键盘.vi"("OldNumber"=w726) -> ("NewNumber"=w727:sgl)
        n449 = local write "标液"(w727) -> ()
      }
      event "质控样": Mouse Down {
        n450 = event-data() -> ()  [unwired: 1 in, 8 out]
        n451 = local read "质控样"() -> (w728:dbl)
        n452 = call "数字键盘.vi"("OldNumber"=w728) -> ("NewNumber"=w729:sgl)
        n453 = local write "质控样"(w729) -> ()
      }
      event "加标回收": Mouse Down {
        n454 = event-data() -> ()  [unwired: 1 in, 8 out]
        n455 = local read "加标回收"() -> (w730:dbl)
        n456 = call "数字键盘.vi"("OldNumber"=w730) -> ("NewNumber"=w731:sgl)
        n457 = local write "加标回收"(w731) -> ()
      }
      event "草酸钠": Mouse Down {
        n458 = event-data() -> ()  [unwired: 1 in, 8 out]
        n459 = local read "草酸钠"() -> (w732:dbl)
        n460 = call "数字键盘.vi"("OldNumber"=w732) -> ("NewNumber"=w733:sgl)
        n461 = local write "草酸钠"(w733) -> ()
      }
      event "高锰酸钾": Mouse Down {
        n462 = event-data() -> ()  [unwired: 1 in, 8 out]
        n463 = local read "高锰酸钾"() -> (w734:dbl)
        n464 = call "数字键盘.vi"("OldNumber"=w734) -> ("NewNumber"=w735:sgl)
        n465 = local write "高锰酸钾"(w735) -> ()
      }
      event "硫酸": Mouse Down {
        n466 = event-data() -> ()  [unwired: 1 in, 8 out]
        n467 = local read "硫酸"() -> (w736:dbl)
        n468 = call "数字键盘.vi"("OldNumber"=w736) -> ("NewNumber"=w737:sgl)
        n469 = local write "硫酸"(w737) -> ()
      }
      event "零点泵计量数 2": Mouse Down {
        n470 = event-data() -> ()  [unwired: 1 in, 8 out]
        n471 = local read "零点泵计量数 2"() -> (w738:dbl)
        n472 = call "数字键盘.vi"("OldNumber"=w738) -> ("NewNumber"=w739:sgl)
        n473 = local write "零点泵计量数 2"(w739) -> ()
      }
      event "标度泵计量数 2": Mouse Down {
        n474 = event-data() -> ()  [unwired: 1 in, 8 out]
        n475 = local read "标度泵计量数 2"() -> (w740:dbl)
        n476 = call "数字键盘.vi"("OldNumber"=w740) -> ("NewNumber"=w741:sgl)
        n477 = local write "标度泵计量数 2"(w741) -> ()
      }
      event "高量程稀释倍数:": Mouse Down {
        n478 = event-data() -> ()  [unwired: 1 in, 8 out]
        n479 = local read "高量程稀释倍数:"() -> (w743:i8)
        n480 = call "数字键盘.vi"("OldNumber"=w743) -> ("NewNumber"=w742:sgl)
        n481 = local write "高量程稀释倍数:"(w742) -> ()
      }
      event "低量程稀释倍数:": Mouse Down {
        n482 = event-data() -> ()  [unwired: 1 in, 8 out]
        n483 = local read "低量程稀释倍数:"() -> (w745:i8)
        n484 = call "数字键盘.vi"("OldNumber"=w745) -> ("NewNumber"=w744:sgl)
        n485 = local write "低量程稀释倍数:"(w744) -> ()
      }
      event "浓度1": Mouse Down {
        n486 = event-data() -> ()  [unwired: 1 in, 8 out]
        n487 = local read "浓度1"() -> (w747:dbl)
        n488 = call "数字键盘.vi"("OldNumber"=w747) -> ("NewNumber"=w746:sgl)
        n489 = property on="浓度1" class="DigNum (严格)"("Val(Sgnl)"=w746) -> ()  [unwired: 2 in, 2 out]
      }
      event "浓度2": Mouse Down {
        n490 = event-data() -> ()  [unwired: 1 in, 8 out]
        n491 = local read "浓度2"() -> (w749:dbl)
        n492 = call "数字键盘.vi"("OldNumber"=w749) -> ("NewNumber"=w748:sgl)
        n493 = property on="浓度2" class="DigNum (严格)"("Val(Sgnl)"=w748) -> ()  [unwired: 2 in, 2 out]
      }
      event "浓度3": Mouse Down {
        n494 = event-data() -> ()  [unwired: 1 in, 8 out]
        n495 = local read "浓度3"() -> (w751:dbl)
        n496 = call "数字键盘.vi"("OldNumber"=w751) -> ("NewNumber"=w750:sgl)
        n497 = property on="浓度3" class="DigNum (严格)"("Val(Sgnl)"=w750) -> ()  [unwired: 2 in, 2 out]
      }
      event "浓度4": Mouse Down {
        n498 = event-data() -> ()  [unwired: 1 in, 8 out]
        n499 = local read "浓度4"() -> (w753:dbl)
        n500 = call "数字键盘.vi"("OldNumber"=w753) -> ("NewNumber"=w752:sgl)
        n501 = property on="浓度4" class="DigNum (严格)"("Val(Sgnl)"=w752) -> ()  [unwired: 2 in, 2 out]
      }
      event "浓度5": Mouse Down {
        n502 = event-data() -> ()  [unwired: 1 in, 8 out]
        n503 = local read "浓度5"() -> (w755:dbl)
        n504 = call "数字键盘.vi"("OldNumber"=w755) -> ("NewNumber"=w754:sgl)
        n505 = property on="浓度5" class="DigNum (严格)"("Val(Sgnl)"=w754) -> ()  [unwired: 2 in, 2 out]
      }
      event "跨度液浓度": Mouse Down {
        n506 = event-data() -> ()  [unwired: 1 in, 8 out]
        n507 = local read "跨度液浓度"() -> (w757:dbl)
        n508 = call "数字键盘.vi"("OldNumber"=w757) -> ("NewNumber"=w756:sgl)
        n509 = property on="跨度液浓度" class="DigNum (严格)"("Val(Sgnl)"=w756) -> ()  [unwired: 2 in, 2 out]
      }
      event "跨度液浓度": Value Change {
        n510 = event-data() -> ()  [unwired: 1 in, 6 out]
        n511 = call <vilib>:"Application Directory.vi"() -> ("Application Directory"=w761:path)
        n512 = Build Path(base path=w761, name or relative path="data\\Set.ini" ("名称或相对路径")) -> (appended path=w763:path)
        n513 = local read "跨度液浓度"() -> (w758:dbl)
        n514 = call <vilib>:"Open Config Data.vi"("configuration file path"=w763) -> ("error out"=w765:errorcluster, "refnum"=w764:T14)  [unwired: 8 in, 1 out]
        n515 = call-poly <vilib>:"Write Key.vi"("section"="CODMn参数" ("key"), "error in (no error)"=w765, "value"=w758, "key"="跨度液浓度", "refnum"=w764) -> ("error out"=w767:errorcluster, "refnum out"=w766:T14)  [unwired: 4 in, 1 out]
        n516 = call <vilib>:"Close Config Data.vi"("error in (no error)"=w767, "refnum"=w766) -> ()  [unwired: 8 in, 2 out]
      }
      event "泵滴定数1": Mouse Down {
        n517 = event-data() -> ()  [unwired: 1 in, 8 out]
        n518 = local read "泵滴定数1"() -> (w769:dbl)
        n519 = call "数字键盘.vi"("OldNumber"=w769) -> ("NewNumber"=w768:sgl)
        n520 = property on="泵滴定数1" class="DigNum (严格)"("Val(Sgnl)"=w768) -> ()  [unwired: 2 in, 2 out]
      }
      event "泵滴定数2": Mouse Down {
        n521 = event-data() -> ()  [unwired: 1 in, 8 out]
        n522 = local read "泵滴定数2"() -> (w771:dbl)
        n523 = call "数字键盘.vi"("OldNumber"=w771) -> ("NewNumber"=w770:sgl)
        n524 = property on="泵滴定数2" class="DigNum (严格)"("Val(Sgnl)"=w770) -> ()  [unwired: 2 in, 2 out]
      }
      event "泵滴定数3": Mouse Down {
        n525 = event-data() -> ()  [unwired: 1 in, 8 out]
        n526 = local read "泵滴定数3"() -> (w773:dbl)
        n527 = call "数字键盘.vi"("OldNumber"=w773) -> ("NewNumber"=w772:sgl)
        n528 = property on="泵滴定数3" class="DigNum (严格)"("Val(Sgnl)"=w772) -> ()  [unwired: 2 in, 2 out]
      }
      event "泵滴定数4": Mouse Down {
        n529 = event-data() -> ()  [unwired: 1 in, 8 out]
        n530 = local read "泵滴定数4"() -> (w775:dbl)
        n531 = call "数字键盘.vi"("OldNumber"=w775) -> ("NewNumber"=w774:sgl)
        n532 = property on="泵滴定数4" class="DigNum (严格)"("Val(Sgnl)"=w774) -> ()  [unwired: 2 in, 2 out]
      }
      event "泵滴定数5": Mouse Down {
        n533 = event-data() -> ()  [unwired: 1 in, 8 out]
        n534 = local read "泵滴定数5"() -> (w777:dbl)
        n535 = call "数字键盘.vi"("OldNumber"=w777) -> ("NewNumber"=w776:sgl)
        n536 = property on="泵滴定数5" class="DigNum (严格)"("Val(Sgnl)"=w776) -> ()  [unwired: 2 in, 2 out]
      }
      event "低切高阈值:", "高切低阈值:": Mouse Down {
        n537 = event-data() -> ("CtlRef"=w781:refnum<vi>)  [unwired: 1 in, 7 out]
        n538 = property class="DigNum (严格)"(reference=w781) -> (reference out=w780:refnum<vi>, "Value"=w779:dbl)  [unwired: 1 in, 1 out]
        n539 = call "数字键盘.vi"("OldNumber"=w779) -> ("NewNumber"=w778:sgl)
        n540 = property class="DigNum (严格)"(reference=w780, "Val(Sgnl)"=w778) -> ()  [unwired: 1 in, 2 out]
      }
    }
  }
  n541 = flat-sequence {
    tunnel: [w782] -> w3
    frame #0 {
      n542 = property on="窗格" class="Pane"("Origin"=T15 {"Horizontal"=0, "Vertical"=0} ("原点")) -> ()  [unwired: 2 in, 2 out]
      n543 = call <vilib>:"Application Directory.vi"() -> ("Application Directory"=w792:path)
      n544 = local write "量程切换次数"(u8 0 ("量程切换次数")) -> ()
      n545 = local write "切换量程连续测两次"(FALSE ("切换量程连续测两次")) -> ()
      n546 = Build Path(base path=w792, name or relative path="data\\sys.ini" ("名称或相对路径")) -> (appended path=w790:path)
      n547 = call <vilib>:"Open Config Data.vi"("configuration file path"=w790) -> ("error out"=w786:errorcluster, "refnum"=w789:T14)  [unwired: 8 in, 1 out]
      n548 = vi-ref "斯坦道CODMn.lvlib:CODMn断电保存全局变量.vi"() -> (w788:refnum<vi>)
      n549 = call <userlib>:"Read Panel from INI__ogtk.vi"("error in (no error)"=w786, "VI ref"=w788, "refnum"=w789) -> ("error out"=w785:errorcluster, "refnum out"=w787:T14)  [unwired: 7 in]
      n550 = call <vilib>:"Close Config Data.vi"("error in (no error)"=w785, "refnum"=w787) -> ("error out"=w784:errorcluster, "file path"=w783:path)  [unwired: 8 in]
      n551 = local write "选用水样"(enum16{"葡萄糖", "草酸钠"}."葡萄糖" ("选用水样")) -> ()
      n552 = local write "量程选择"(enum16{"低量程", "高量程", "0-2量程"}."低量程" ("量程选择")) -> ()
      n553 = Open/Create/Replace File(file path (use dialog)=w783, error in=w784) -> (error out=w782:errorcluster)  [unwired: 4 in, 2 out]
      "稀释倍数解释" <- "稀释倍数解释：\n稀释倍数选择1，表示不稀释\n默认低量程系数倍数1，高量程系数倍数2\n则低量程为0~8，高量程为0~16" ("稀释倍数解释")
    }
  }
  n554 = vi-ref "CODMn通讯.vi"() -> (w2:refnum<vi>)
  n555 = property class="VI"(reference=w2) -> ("Name"=w4:string)  [unwired: 1 in, 2 out]
  n556 = Open VI Reference(type specifier VI Refnum (for type only)=refnum<vi> refnum, vi path=w4, options=128 ("选项")) -> (vi reference=w6:refnum<vi>, error out=w8:errorcluster)  [unwired: 3 in]
  n557 = call-by-ref "?"(reference=w6, error in=w8) -> (reference out=w10:refnum<vi>, error out=w9:errorcluster)  [unwired: 12 in]
  n558 = Close Reference(reference=w10, error in (no error)=w9) -> ()  [unwired: 1 out]
  n559 = Obtain Queue(name (unnamed)="CODMn" ("名称（未命名）"), element data type=cluster{"命令":string} {"命令"="启用模块"} ("元素")) -> (queue out=w12:refnum<queue>, error out=w11:errorcluster)  [unwired: 3 in, 1 out]
  n560 = while {
    tunnel: w12 -> [w800]
    tunnel: w11 -> [w799]
    stop <- FALSE stop-if-true
    # "主线事件"
    n561 = event shown="[30] \"打开串口\": 值改变" {
      selector: _ -> [_ _ _ _ _ _ _ _ _ _ _ _ _ _ _ _ _ _ _ _ _ _ _ _ _ _ _ _ _ _ _ _]
      dyn-events: _ -> [_ _ _ _ _ _ _ _ _ _ _ _ _ _ _ _ _ _ _ _ _ _ _ _ _ _ _ _ _ _ _ _]
      timeout: _ -> [_ _ _ _ _ _ _ _ _ _ _ _ _ _ _ _ _ _ _ _ _ _ _ _ _ _ _ _ _ _ _ _]
      tunnel: w800 -> [_ _ _ _ _ w856 _ _ _ _ _ _ _ _ _ _ _ _ _ _ _ _ _ _ w1439 _ _ _ _ w1641 w1648 _]
      tunnel: w799 -> [_ _ _ _ _ w855 _ _ _ _ _ _ _ _ _ _ _ _ _ _ _ _ _ _ w1438 _ _ _ _ w1640 w1647 _]
      event "单步启动": Mouse Down {
        n562 = event-data() -> ()  [unwired: 1 in, 8 out]
        n563 = call "CODMn手动控制框.vi"() -> ()  [unwired: 12 in]
      }
      event "启动": Mouse Down {
        n564 = event-data() -> ()  [unwired: 1 in, 8 out]
        n565 = flat-sequence {
          tunnel: [w803] -> w802
          tunnel: w802 -> [w809]
          frame #0 {
            n566 = call "启动测量模式选择对话框.vi"() -> ("启动选择 2"=w803:u16)  [unwired: 11 in]
            "启动选择 2" <- w803
          }
          frame #1 {
            n567 = case shown="9, 默认" w809 {
              tunnel: [u16 4608 ("address") u16 4608 ("address") u16 4608 ("address") u16 4608 ("address") u16 4608 ("address") u16 4608 ("address") u16 4608 ("address") u16 4608 ("address") u16 4608 ("address") u16 4608 ("address")] -> w805
              tunnel: [u16 1 ("address") u16 2 ("address") u16 3 ("address") u16 4 ("address") u16 5 ("address") u16 7 ("address") u16 6 ("address") u16 8 ("address") u16 9 ("address") u16 0 ("address")] -> w810
              frame 0 {
              }
              frame 1 {
              }
              frame 2 {
              }
              frame 3 {
              }
              frame 4 {
              }
              frame 5 {
              }
              frame 6 {
              }
              frame 7 {
              }
              frame 8 {
              }
              frame 9, Default {
              }
            }
            n568 = Not Equal?(x=w809, y=u16 9) -> (x != y?=w807:bool)
            n569 = global write "CODMN外部API.vi" "手动启动CODMn"(w807) -> ()
            n570 = Insert Into Array(array=u16[] [] ("values"), index=0 ("索引"), new element=w810) -> (w804:u16[])
            n571 = call "CODMnMB_api.vi"("STEP"=enum16{"open", "read", "write", "close"}."write", "values"=w804, "starting address"=w805) -> ()  [unwired: 5 in, 4 out]
          }
        }
      }
      event "停止": Value Change {
        n572 = event-data() -> ()  [unwired: 1 in, 6 out]
        n573 = Two Button Dialog(message="确认是否停止？" ("消息"), 1:"否" ("F按钮名称（“取消”）"), 2:"是" ("T按钮名称（“确定”）")) -> (T button?=w835:bool)
        n574 = case shown="真" w835 {
          frame False {
          }
          frame True {
            n575 = call "CODMnMB_api.vi"("STEP"=enum16{"open", "read", "write", "close"}."write", "values"=u16[] [11], "starting address"=u16 4608) -> ()  [unwired: 5 in, 4 out]
          }
        }
      }
      event "手动控制": Value Change {
        n576 = event-data() -> ()  [unwired: 1 in, 6 out]
        n577 = call "数字密码键盘.vi"() -> ("NewNumber"=w840:sgl)  [unwired: 1 in]
        n578 = Equal?(x=w840, y=8.0) -> (x = y?=w841:bool)
        n579 = case shown="假" w841 {
          frame False {
            n580 = call "窗口弹出对话框(子VI).vi"("消息"="密码错误") -> ()  [unwired: 10 in, 1 out]
          }
          frame True {
          }
        }
      }
      event "锁定按钮": Mouse Down {
        n581 = event-data() -> ("CtlRef"=w846:refnum<vi>)  [unwired: 1 in, 7 out]
        n582 = property class="Bool (严格)"(reference=w846) -> ("Value"=w845:bool)  [unwired: 1 in, 2 out]
        n583 = case shown="真" w845 {
          selector: w845 -> [w847 _]
          tunnel: [w847 w848] -> w844
          frame False {
          }
          frame True {
            n584 = call "数字密码键盘.vi"() -> ("NewNumber"=w849:sgl)  [unwired: 1 in]
            n585 = Equal?(x=w849, y=8.0) -> (x = y?=w848:bool)
            n586 = case shown="假" w848 {
              selector: w848 -> [w852 _]
              frame False {
                n587 = One Button Dialog(message="密码错误!" ("消息")) -> ()  [unwired: 1 in, 1 out]
                n588 = local write "锁定按钮"(w852) -> ()
              }
              frame True {
                n589 = One Button Dialog(message="解锁成功!" ("消息")) -> ()  [unwired: 1 in, 1 out]
              }
            }
          }
        }
        "x = y?" <- w844
      }
      event "参数配置": Value Change {
        (unwired) u16 20 ("number of holding registers")
        (unwired) u16 4272 ("starting address")
        n590 = event-data() -> ()  [unwired: 1 in, 6 out]
        n591 = property on="窗格" class="Pane"("Origin"=T15 {"Horizontal"=0, "Vertical"=650} ("原点")) -> ()  [unwired: 2 in, 2 out]
        n592 = Bundle By Name(cluster=cluster{"命令":string} {"命令"=""} ("元素"), "命令"="CODMn读取参数" ("名称（未命名）")) -> (w857:cluster{"命令":string})
        n593 = Enqueue Element(queue=w856, element=w857, error in (no error)=w855) -> ()  [unwired: 1 in, 3 out]
        n594 = call <vilib>:"Application Directory.vi"() -> ("Application Directory"=w860:path)
        n595 = Build Path(base path=w860, name or relative path="data\\sys.ini" ("名称或相对路径")) -> (appended path=w862:path)
        n596 = call <vilib>:"Open Config Data.vi"("configuration file path"=w862) -> ("error out"=w866:errorcluster, "refnum"=w863:T14)  [unwired: 8 in, 1 out]
        n597 = vi-ref "斯坦道CODMn.lvlib:CODMn断电保存全局变量.vi"() -> (w864:refnum<vi>)
        n598 = call <userlib>:"Read Panel from INI__ogtk.vi"("error in (no error)"=w866, "VI ref"=w864, "refnum"=w863) -> ("error out"=w867:errorcluster, "refnum out"=w865:T14)  [unwired: 7 in]
        n599 = call <vilib>:"Close Config Data.vi"("error in (no error)"=w867, "refnum"=w865) -> ("error out"=w868:errorcluster, "file path"=w869:path)  [unwired: 8 in]
        n600 = Open/Create/Replace File(file path (use dialog)=w869, error in=w868) -> (error out=w854:errorcluster)  [unwired: 4 in, 2 out]
        n601 = call <vilib>:"Clear Errors.vi"("error in (no error)"=w854) -> ()  [unwired: 5 in, 2 out]
      }
      event "保存": Mouse Down {
        n602 = event-data() -> ()  [unwired: 1 in, 8 out]
        n603 = call "CODMnMB_api.vi"("STEP"=enum16{"open", "read", "write", "close"}."write", "values"="保存参数", "starting address"=u16 4272) -> ()  [unwired: 5 in, 4 out]
      }
      event "跨度液浓度", "常规版/认证版": Value Change {
        n604 = event-data() -> ()  [unwired: 1 in, 6 out]
        n605 = flat-sequence {
          frame #0 {
            n606 = global write "CODMn断电保存全局变量.vi" "常规版/认证版"("常规版/认证版") -> ()
            n607 = global write "CODMn断电保存全局变量.vi" "跨度液浓度"("跨度液浓度") -> ()
          }
          frame #1 {
            n608 = call <vilib>:"Application Directory.vi"() -> ("Application Directory"=w889:path)
            n609 = Build Path(base path=w889, name or relative path="data\\sys.ini" ("名称或相对路径")) -> (appended path=w887:path)
            n610 = call <vilib>:"Open Config Data.vi"("configuration file path"=w887) -> ("error out"=w883:errorcluster, "refnum"=w886:T14)  [unwired: 8 in, 1 out]
            n611 = vi-ref "斯坦道CODMn.lvlib:CODMn断电保存全局变量.vi"() -> (w885:refnum<vi>)
            n612 = call <userlib>:"Write Panel to INI__ogtk.vi"("error in (no error)"=w883, "VI ref"=w885, "refnum"=w886) -> ("error out"=w882:errorcluster, "refnum out"=w884:T14)  [unwired: 7 in]
            n613 = call <vilib>:"Close Config Data.vi"("error in (no error)"=w882, "refnum"=w884) -> ("error out"=w877:errorcluster, "file path"=w876:path)  [unwired: 8 in]
            n614 = Open/Create/Replace File(file path (use dialog)=w876, error in=w877) -> (refnum out=w880:refnum<file>, error out=w881:errorcluster)  [unwired: 4 in, 1 out]
            n615 = Flush File(refnum=w880, error in=w881) -> (refnum out=w879:refnum<file>, error out=w878:errorcluster)
            n616 = Close File(refnum=w879, error in=w878) -> ()  [unwired: 2 out]
          }
        }
      }
      event "校准配置": Value Change {
        n617 = event-data() -> ()  [unwired: 1 in, 6 out]
        n618 = property on="窗格" class="Pane"("Origin"=T15 {"Horizontal"=0, "Vertical"=1300} ("原点")) -> ()  [unwired: 2 in, 2 out]
        n619 = call <vilib>:"Application Directory.vi"() -> ("Application Directory"=w940:path)
        n620 = Build Path(base path=w940, name or relative path="data\\Set.ini" ("名称或相对路径")) -> (appended path=w938:path)
        n621 = call <vilib>:"Open Config Data.vi"("configuration file path"=w938) -> ("error out"=w908:errorcluster, "refnum"=w909:T14)  [unwired: 8 in, 1 out]
        n622 = local read "量程选择"() -> (w915:enum16{"低量程", "高量程", "0-2量程"})
        n623 = call-poly <vilib>:"Read Key.vi"("section"="CODMn模型选择" ("key"), "error in (no error)"=w908, "key"="线性和多项式", "refnum"=w909) -> ("error out"=w905:errorcluster, "value"=w907:i32, "refnum out"=w906:T14)  [unwired: 4 in, 1 out]
        n624 = case shown="\"0-2量程\"" w915 {
          tunnel: ["低量程" "高量程" "0-2量程"] -> w913
          frame "低量程", Default {
          }
          frame "高量程" {
          }
          frame "0-2量程" {
          }
        }
        n625 = local write "模型"(w907) -> ()
        n626 = call-poly <vilib>:"Read Key.vi"("section"="标线选择", "error in (no error)"=w905, "key"="选用水样", "refnum"=w906) -> ("error out"=w903:errorcluster, "value"=w890:i32, "refnum out"=w904:T14)  [unwired: 4 in, 1 out]
        n627 = case shown="0, 默认" w890 {
          tunnel: ["葡萄糖标线" ("section") "草酸钠标线" ("section")] -> w914
          frame 0, Default {
          }
          frame 1 {
          }
        }
        n628 = local write "选用水样"(w890) -> ()
        n629 = Concatenate Strings(w914, w913) -> (w912:string)
        n630 = call-poly <vilib>:"Read Key.vi"("section"=w912, "error in (no error)"=w903, "key"="浓度1", "refnum"=w904) -> ("error out"=w944:errorcluster, "value"=w942:dbl, "refnum out"=w943:T14)  [unwired: 4 in, 1 out]
        n631 = local write "浓度1"(w942) -> ()
        n632 = call-poly <vilib>:"Read Key.vi"("section"=w912, "error in (no error)"=w944, "key"="浓度2", "refnum"=w943) -> ("error out"=w958:errorcluster, "value"=w945:dbl, "refnum out"=w957:T14)  [unwired: 4 in, 1 out]
        n633 = local write "浓度2"(w945) -> ()
        n634 = call-poly <vilib>:"Read Key.vi"("section"=w912, "error in (no error)"=w958, "key"="浓度3", "refnum"=w957) -> ("error out"=w959:errorcluster, "value"=w947:dbl, "refnum out"=w956:T14)  [unwired: 4 in, 1 out]
        n635 = local write "浓度3"(w947) -> ()
        n636 = call-poly <vilib>:"Read Key.vi"("section"=w912, "error in (no error)"=w959, "key"="泵滴定数1", "refnum"=w956) -> ("error out"=w960:errorcluster, "value"=w949:dbl, "refnum out"=w955:T14)  [unwired: 4 in, 1 out]
        n637 = local write "泵滴定数1"(w949) -> ()
        n638 = call-poly <vilib>:"Read Key.vi"("section"=w912, "error in (no error)"=w960, "key"="泵滴定数2", "refnum"=w955) -> ("error out"=w954:errorcluster, "value"=w952:dbl, "refnum out"=w961:T14)  [unwired: 4 in, 1 out]
        n639 = local write "泵滴定数2"(w952) -> ()
        n640 = call-poly <vilib>:"Read Key.vi"("section"=w912, "error in (no error)"=w954, "key"="泵滴定数3", "refnum"=w961) -> ("error out"=w966:errorcluster, "value"=w965:dbl, "refnum out"=w962:T14)  [unwired: 4 in, 1 out]
        n641 = local write "泵滴定数3"(w965) -> ()
        n642 = call-poly <vilib>:"Read Key.vi"("section"=w912, "error in (no error)"=w966, "key"="浓度4", "refnum"=w962) -> ("error out"=w967:errorcluster, "value"=w896:dbl, "refnum out"=w963:T14)  [unwired: 4 in, 1 out]
        n643 = local write "浓度4"(w896) -> ()
        n644 = call-poly <vilib>:"Read Key.vi"("section"=w912, "error in (no error)"=w967, "key"="浓度5", "refnum"=w963) -> ("error out"=w901:errorcluster, "value"=w895:dbl, "refnum out"=w902:T14)  [unwired: 4 in, 1 out]
        n645 = local write "浓度5"(w895) -> ()
        n646 = call-poly <vilib>:"Read Key.vi"("section"=w912, "error in (no error)"=w901, "key"="泵滴定数4", "refnum"=w902) -> ("error out"=w968:errorcluster, "value"=w894:dbl, "refnum out"=w964:T14)  [unwired: 4 in, 1 out]
        n647 = local write "泵滴定数4"(w894) -> ()
        n648 = call-poly <vilib>:"Read Key.vi"("section"=w912, "error in (no error)"=w968, "key"="泵滴定数5", "refnum"=w964) -> ("error out"=w899:errorcluster, "value"=w893:dbl, "refnum out"=w900:T14)  [unwired: 4 in, 1 out]
        n649 = local write "泵滴定数5"(w893) -> ()
        n650 = call-poly <vilib>:"Read Key.vi"("section"=w912, "error in (no error)"=w899, "key"="当前选用的校准", "refnum"=w900) -> ("error out"=w934:errorcluster, "value"=w936:i32, "refnum out"=w935:T14)  [unwired: 4 in, 1 out]
        n651 = local write "当前校准"(w936) -> ()
        n652 = call-poly <vilib>:"Read Key.vi"("section"=w912, "error in (no error)"=w934, "key"="启用1", "refnum"=w935) -> ("error out"=w931:errorcluster, "value"=w920:bool, "refnum out"=w932:T14)  [unwired: 4 in, 1 out]
        n653 = local write "启用1"(w920) -> ()
        n654 = call-poly <vilib>:"Read Key.vi"("section"=w912, "error in (no error)"=w931, "key"="启用2", "refnum"=w932) -> ("error out"=w929:errorcluster, "value"=w919:bool, "refnum out"=w930:T14)  [unwired: 4 in, 1 out]
        n655 = local write "启用2"(w919) -> ()
        n656 = call-poly <vilib>:"Read Key.vi"("section"=w912, "error in (no error)"=w929, "key"="启用3", "refnum"=w930) -> ("error out"=w927:errorcluster, "value"=w918:bool, "refnum out"=w928:T14)  [unwired: 4 in, 1 out]
        n657 = local write "启用3"(w918) -> ()
        n658 = call-poly <vilib>:"Read Key.vi"("section"=w912, "error in (no error)"=w927, "key"="启用4", "refnum"=w928) -> ("error out"=w925:errorcluster, "value"=w892:bool, "refnum out"=w926:T14)  [unwired: 4 in, 1 out]
        n659 = local write "启用4"(w892) -> ()
        n660 = call-poly <vilib>:"Read Key.vi"("section"=w912, "error in (no error)"=w925, "key"="启用5", "refnum"=w926) -> ("error out"=w897:errorcluster, "value"=w891:bool, "refnum out"=w898:T14)  [unwired: 4 in, 1 out]
        n661 = local write "启用5"(w891) -> ()
        n662 = call <vilib>:"Close Config Data.vi"("error in (no error)"=w897, "refnum"=w898) -> ()  [unwired: 8 in, 2 out]
      }
      event "选用水样": Value Change {
        (unwired) "浓度6" ("key")
        n663 = event-data() -> ()  [unwired: 1 in, 6 out]
        n664 = property on="窗格" class="Pane"("Origin"=T15 {"Horizontal"=0, "Vertical"=1300} ("原点")) -> ()  [unwired: 2 in, 2 out]
        n665 = local read "量程选择"() -> (w992:enum16{"低量程", "高量程", "0-2量程"})
        n666 = case shown="\"0-2量程\"" w992 {
          tunnel: ["低量程" "高量程" "0-2量程"] -> w993
          frame "低量程", Default {
          }
          frame "高量程" {
          }
          frame "0-2量程" {
          }
        }
        n667 = case shown="\"葡萄糖\", 默认" "选用水样" {
          tunnel: ["葡萄糖标线" ("section") "草酸钠标线" ("section")] -> w994
          frame "葡萄糖", Default {
          }
          frame "草酸钠" {
          }
        }
        n668 = call <vilib>:"Application Directory.vi"() -> ("Application Directory"=w1018:path)
        n669 = Build Path(base path=w1018, name or relative path="data\\Set.ini" ("名称或相对路径")) -> (appended path=w1016:path)
        n670 = call <vilib>:"Open Config Data.vi"("configuration file path"=w1016) -> ("error out"=w1019:errorcluster, "refnum"=w1020:T14)  [unwired: 8 in, 1 out]
        n671 = Concatenate Strings(w994, w993) -> (w991:string)
        n672 = call-poly <vilib>:"Read Key.vi"("section"=w991, "error in (no error)"=w1019, "key"="浓度1", "refnum"=w1020) -> ("error out"=w1024:errorcluster, "value"=w1022:dbl, "refnum out"=w1023:T14)  [unwired: 4 in, 1 out]
        n673 = local write "浓度1"(w1022) -> ()
        n674 = call-poly <vilib>:"Read Key.vi"("section"=w991, "error in (no error)"=w1024, "key"="浓度2", "refnum"=w1023) -> ("error out"=w1038:errorcluster, "value"=w1025:dbl, "refnum out"=w1037:T14)  [unwired: 4 in, 1 out]
        n675 = local write "浓度2"(w1025) -> ()
        n676 = call-poly <vilib>:"Read Key.vi"("section"=w991, "error in (no error)"=w1038, "key"="浓度3", "refnum"=w1037) -> ("error out"=w1039:errorcluster, "value"=w1027:dbl, "refnum out"=w1036:T14)  [unwired: 4 in, 1 out]
        n677 = local write "浓度3"(w1027) -> ()
        n678 = call-poly <vilib>:"Read Key.vi"("section"=w991, "error in (no error)"=w1039, "key"="泵滴定数1", "refnum"=w1036) -> ("error out"=w1040:errorcluster, "value"=w1029:dbl, "refnum out"=w1035:T14)  [unwired: 4 in, 1 out]
        n679 = local write "泵滴定数1"(w1029) -> ()
        n680 = call-poly <vilib>:"Read Key.vi"("section"=w991, "error in (no error)"=w1040, "key"="泵滴定数2", "refnum"=w1035) -> ("error out"=w1034:errorcluster, "value"=w1032:dbl, "refnum out"=w1041:T14)  [unwired: 4 in, 1 out]
        n681 = local write "泵滴定数2"(w1032) -> ()
        n682 = call-poly <vilib>:"Read Key.vi"("section"=w991, "error in (no error)"=w1034, "key"="泵滴定数3", "refnum"=w1041) -> ("error out"=w1046:errorcluster, "value"=w1045:dbl, "refnum out"=w1042:T14)  [unwired: 4 in, 1 out]
        n683 = local write "泵滴定数3"(w1045) -> ()
        n684 = call-poly <vilib>:"Read Key.vi"("section"=w991, "error in (no error)"=w1046, "key"="浓度4", "refnum"=w1042) -> ("error out"=w1047:errorcluster, "value"=w986:dbl, "refnum out"=w1043:T14)  [unwired: 4 in, 1 out]
        n685 = local write "浓度4"(w986) -> ()
        n686 = call-poly <vilib>:"Read Key.vi"("section"=w991, "error in (no error)"=w1047, "key"="浓度5", "refnum"=w1043) -> ("error out"=w989:errorcluster, "value"=w985:dbl, "refnum out"=w990:T14)  [unwired: 4 in, 1 out]
        n687 = local write "浓度5"(w985) -> ()
        n688 = call-poly <vilib>:"Read Key.vi"("section"=w991, "error in (no error)"=w989, "key"="泵滴定数4", "refnum"=w990) -> ("error out"=w1048:errorcluster, "value"=w984:dbl, "refnum out"=w1044:T14)  [unwired: 4 in, 1 out]
        n689 = local write "泵滴定数4"(w984) -> ()
        n690 = call-poly <vilib>:"Read Key.vi"("section"=w991, "error in (no error)"=w1048, "key"="泵滴定数5", "refnum"=w1044) -> ("error out"=w987:errorcluster, "value"=w983:dbl, "refnum out"=w988:T14)  [unwired: 4 in, 1 out]
        n691 = local write "泵滴定数5"(w983) -> ()
        n692 = call-poly <vilib>:"Read Key.vi"("section"=w991, "error in (no error)"=w987, "key"="当前选用的校准", "refnum"=w988) -> ("error out"=w1012:errorcluster, "value"=w1014:i32, "refnum out"=w1013:T14)  [unwired: 4 in, 1 out]
        n693 = call-poly <vilib>:"Read Key.vi"("section"=w991, "error in (no error)"=w1012, "key"="启用1", "refnum"=w1013) -> ("error out"=w1009:errorcluster, "value"=w998:bool, "refnum out"=w1010:T14)  [unwired: 4 in, 1 out]
        n694 = local write "当前校准"(w1014) -> ()
        n695 = local write "启用1"(w998) -> ()
        n696 = call-poly <vilib>:"Read Key.vi"("section"=w991, "error in (no error)"=w1009, "key"="启用2", "refnum"=w1010) -> ("error out"=w1007:errorcluster, "value"=w997:bool, "refnum out"=w1008:T14)  [unwired: 4 in, 1 out]
        n697 = local write "启用2"(w997) -> ()
        n698 = call-poly <vilib>:"Read Key.vi"("section"=w991, "error in (no error)"=w1007, "key"="启用3", "refnum"=w1008) -> ("error out"=w1005:errorcluster, "value"=w996:bool, "refnum out"=w1006:T14)  [unwired: 4 in, 1 out]
        n699 = local write "启用3"(w996) -> ()
        n700 = call-poly <vilib>:"Read Key.vi"("section"=w991, "error in (no error)"=w1005, "key"="启用4", "refnum"=w1006) -> ("error out"=w1003:errorcluster, "value"=w980:bool, "refnum out"=w1004:T14)  [unwired: 4 in, 1 out]
        n701 = local write "启用4"(w980) -> ()
        n702 = call-poly <vilib>:"Read Key.vi"("section"=w991, "error in (no error)"=w1003, "key"="启用5", "refnum"=w1004) -> ("error out"=w981:errorcluster, "value"=w979:bool, "refnum out"=w982:T14)  [unwired: 4 in, 1 out]
        n703 = local write "启用5"(w979) -> ()
        n704 = call <vilib>:"Close Config Data.vi"("error in (no error)"=w981, "refnum"=w982) -> ()  [unwired: 8 in, 2 out]
      }
      event "量程选择": Value Change {
        n705 = event-data() -> ()  [unwired: 1 in, 6 out]
        n706 = local read "选用水样"() -> (w1075:enum16{"葡萄糖", "草酸钠"})
        n707 = property on="窗格" class="Pane"("Origin"=T15 {"Horizontal"=0, "Vertical"=1300} ("原点")) -> ()  [unwired: 2 in, 2 out]
        n708 = case shown="\"葡萄糖\", 默认" w1075 {
          tunnel: ["葡萄糖标线" ("section") "草酸钠标线" ("section")] -> w1074
          frame "葡萄糖", Default {
          }
          frame "草酸钠" {
          }
        }
        n709 = case shown="\"0-2量程\"" "量程选择" {
          tunnel: ["低量程" "高量程" "0-2量程"] -> w1071
          frame "低量程", Default {
          }
          frame "高量程" {
          }
          frame "0-2量程" {
          }
        }
        n710 = call <vilib>:"Application Directory.vi"() -> ("Application Directory"=w1098:path)
        n711 = Build Path(base path=w1098, name or relative path="data\\Set.ini" ("名称或相对路径")) -> (appended path=w1096:path)
        n712 = call <vilib>:"Open Config Data.vi"("configuration file path"=w1096) -> ("error out"=w1099:errorcluster, "refnum"=w1100:T14)  [unwired: 8 in, 1 out]
        n713 = Concatenate Strings(w1074, w1071) -> (w1073:string)
        n714 = call-poly <vilib>:"Read Key.vi"("section"=w1073, "error in (no error)"=w1099, "key"="浓度1", "refnum"=w1100) -> ("error out"=w1104:errorcluster, "value"=w1102:dbl, "refnum out"=w1103:T14)  [unwired: 4 in, 1 out]
        n715 = local write "浓度1"(w1102) -> ()
        n716 = call-poly <vilib>:"Read Key.vi"("section"=w1073, "error in (no error)"=w1104, "key"="浓度2", "refnum"=w1103) -> ("error out"=w1118:errorcluster, "value"=w1105:dbl, "refnum out"=w1117:T14)  [unwired: 4 in, 1 out]
        n717 = local write "浓度2"(w1105) -> ()
        n718 = call-poly <vilib>:"Read Key.vi"("section"=w1073, "error in (no error)"=w1118, "key"="浓度3", "refnum"=w1117) -> ("error out"=w1119:errorcluster, "value"=w1107:dbl, "refnum out"=w1116:T14)  [unwired: 4 in, 1 out]
        n719 = local write "浓度3"(w1107) -> ()
        n720 = call-poly <vilib>:"Read Key.vi"("section"=w1073, "error in (no error)"=w1119, "key"="泵滴定数1", "refnum"=w1116) -> ("error out"=w1120:errorcluster, "value"=w1109:dbl, "refnum out"=w1115:T14)  [unwired: 4 in, 1 out]
        n721 = local write "泵滴定数1"(w1109) -> ()
        n722 = call-poly <vilib>:"Read Key.vi"("section"=w1073, "error in (no error)"=w1120, "key"="泵滴定数2", "refnum"=w1115) -> ("error out"=w1114:errorcluster, "value"=w1112:dbl, "refnum out"=w1121:T14)  [unwired: 4 in, 1 out]
        n723 = local write "泵滴定数2"(w1112) -> ()
        n724 = call-poly <vilib>:"Read Key.vi"("section"=w1073, "error in (no error)"=w1114, "key"="泵滴定数3", "refnum"=w1121) -> ("error out"=w1126:errorcluster, "value"=w1125:dbl, "refnum out"=w1122:T14)  [unwired: 4 in, 1 out]
        n725 = local write "泵滴定数3"(w1125) -> ()
        n726 = call-poly <vilib>:"Read Key.vi"("section"=w1073, "error in (no error)"=w1126, "key"="浓度4", "refnum"=w1122) -> ("error out"=w1127:errorcluster, "value"=w1062:dbl, "refnum out"=w1123:T14)  [unwired: 4 in, 1 out]
        n727 = local write "浓度4"(w1062) -> ()
        n728 = call-poly <vilib>:"Read Key.vi"("section"=w1073, "error in (no error)"=w1127, "key"="浓度5", "refnum"=w1123) -> ("error out"=w1069:errorcluster, "value"=w1061:dbl, "refnum out"=w1070:T14)  [unwired: 4 in, 1 out]
        n729 = local write "浓度5"(w1061) -> ()
        n730 = call-poly <vilib>:"Read Key.vi"("section"=w1073, "error in (no error)"=w1069, "key"="泵滴定数4", "refnum"=w1070) -> ("error out"=w1128:errorcluster, "value"=w1060:dbl, "refnum out"=w1124:T14)  [unwired: 4 in, 1 out]
        n731 = local write "泵滴定数4"(w1060) -> ()
        n732 = call-poly <vilib>:"Read Key.vi"("section"=w1073, "error in (no error)"=w1128, "key"="泵滴定数5", "refnum"=w1124) -> ("error out"=w1067:errorcluster, "value"=w1059:dbl, "refnum out"=w1068:T14)  [unwired: 4 in, 1 out]
        n733 = local write "泵滴定数5"(w1059) -> ()
        n734 = call-poly <vilib>:"Read Key.vi"("section"=w1073, "error in (no error)"=w1067, "key"="当前选用的校准", "refnum"=w1068) -> ("error out"=w1092:errorcluster, "value"=w1094:i32, "refnum out"=w1093:T14)  [unwired: 4 in, 1 out]
        n735 = local write "当前校准"(w1094) -> ()
        n736 = call-poly <vilib>:"Read Key.vi"("section"=w1073, "error in (no error)"=w1092, "key"="启用1", "refnum"=w1093) -> ("error out"=w1089:errorcluster, "value"=w1078:bool, "refnum out"=w1090:T14)  [unwired: 4 in, 1 out]
        n737 = local write "启用1"(w1078) -> ()
        n738 = call-poly <vilib>:"Read Key.vi"("section"=w1073, "error in (no error)"=w1089, "key"="启用2", "refnum"=w1090) -> ("error out"=w1087:errorcluster, "value"=w1077:bool, "refnum out"=w1088:T14)  [unwired: 4 in, 1 out]
        n739 = local write "启用2"(w1077) -> ()
        n740 = call-poly <vilib>:"Read Key.vi"("section"=w1073, "error in (no error)"=w1087, "key"="启用3", "refnum"=w1088) -> ("error out"=w1085:errorcluster, "value"=w1076:bool, "refnum out"=w1086:T14)  [unwired: 4 in, 1 out]
        n741 = local write "启用3"(w1076) -> ()
        n742 = call-poly <vilib>:"Read Key.vi"("section"=w1073, "error in (no error)"=w1085, "key"="启用4", "refnum"=w1086) -> ("error out"=w1083:errorcluster, "value"=w1064:bool, "refnum out"=w1084:T14)  [unwired: 4 in, 1 out]
        n743 = local write "启用4"(w1064) -> ()
        n744 = call-poly <vilib>:"Read Key.vi"("section"=w1073, "error in (no error)"=w1083, "key"="启用5", "refnum"=w1084) -> ("error out"=w1065:errorcluster, "value"=w1063:bool, "refnum out"=w1066:T14)  [unwired: 4 in, 1 out]
        n745 = local write "启用5"(w1063) -> ()
        n746 = call <vilib>:"Close Config Data.vi"("error in (no error)"=w1065, "refnum"=w1066) -> ()  [unwired: 8 in, 2 out]
      }
      event "返回": Value Change {
        w1152 = "CODMn" ("section")
        n747 = event-data() -> ()  [unwired: 1 in, 6 out]
        n748 = property on="窗格" class="Pane"("Origin"=T15 {"Horizontal"=0, "Vertical"=0} ("原点")) -> ()  [unwired: 2 in, 2 out]
        n749 = call <vilib>:"Application Directory.vi"() -> ("Application Directory"=w1205:path)
        n750 = Build Path(base path=w1205, name or relative path="data\\Set.ini" ("名称或相对路径")) -> (appended path=w1203:path)
        n751 = local read "浓度1"() -> (w1199:dbl)
        n752 = call <vilib>:"Open Config Data.vi"("configuration file path"=w1203) -> ("error out"=w1201:errorcluster, "refnum"=w1202:T14)  [unwired: 8 in, 1 out]
        n753 = local read "浓度2"() -> (w1183:dbl)
        n754 = call-poly <vilib>:"Write Key.vi"("section"=w1152, "error in (no error)"=w1201, "value"=w1199, "key"="浓度1", "refnum"=w1202) -> ("error out"=w1198:errorcluster, "refnum out"=w1197:T14)  [unwired: 4 in, 1 out]
        n755 = local read "浓度3"() -> (w1179:dbl)
        n756 = call-poly <vilib>:"Write Key.vi"("section"=w1152, "error in (no error)"=w1198, "value"=w1183, "key"="浓度2", "refnum"=w1197) -> ("error out"=w1196:errorcluster, "refnum out"=w1195:T14)  [unwired: 4 in, 1 out]
        n757 = local read "泵滴定数1"() -> (w1177:dbl)
        n758 = call-poly <vilib>:"Write Key.vi"("section"=w1152, "error in (no error)"=w1196, "value"=w1179, "key"="浓度3", "refnum"=w1195) -> ("error out"=w1194:errorcluster, "refnum out"=w1193:T14)  [unwired: 4 in, 1 out]
        n759 = call-poly <vilib>:"Write Key.vi"("section"=w1152, "error in (no error)"=w1194, "value"=w1177, "key"="泵滴定数1", "refnum"=w1193) -> ("error out"=w1192:errorcluster, "refnum out"=w1191:T14)  [unwired: 4 in, 1 out]
        n760 = local read "泵滴定数2"() -> (w1175:dbl)
        n761 = call-poly <vilib>:"Write Key.vi"("section"=w1152, "error in (no error)"=w1192, "value"=w1175, "key"="泵滴定数2", "refnum"=w1191) -> ("error out"=w1190:errorcluster, "refnum out"=w1189:T14)  [unwired: 4 in, 1 out]
        n762 = local read "泵滴定数3"() -> (w1173:dbl)
        n763 = local read "浓度4"() -> (w1140:dbl)
        n764 = call-poly <vilib>:"Write Key.vi"("section"=w1152, "error in (no error)"=w1190, "value"=w1173, "key"="泵滴定数3", "refnum"=w1189) -> ("error out"=w1188:errorcluster, "refnum out"=w1187:T14)  [unwired: 4 in, 1 out]
        n765 = call-poly <vilib>:"Write Key.vi"("section"=w1152, "error in (no error)"=w1188, "value"=w1140, "key"="浓度4", "refnum"=w1187) -> ("error out"=w1181:errorcluster, "refnum out"=w1182:T14)  [unwired: 4 in, 1 out]
        n766 = local read "浓度5"() -> (w1139:dbl)
        n767 = call-poly <vilib>:"Write Key.vi"("section"=w1152, "error in (no error)"=w1181, "value"=w1139, "key"="浓度5", "refnum"=w1182) -> ("error out"=w1149:errorcluster, "refnum out"=w1150:T14)  [unwired: 4 in, 1 out]
        n768 = local read "泵滴定数4"() -> (w1141:dbl)
        n769 = call-poly <vilib>:"Write Key.vi"("section"=w1152, "error in (no error)"=w1149, "value"=w1141, "key"="泵滴定数4", "refnum"=w1150) -> ("error out"=w1186:errorcluster, "refnum out"=w1185:T14)  [unwired: 4 in, 1 out]
        n770 = local read "泵滴定数5"() -> (w1142:dbl)
        n771 = call-poly <vilib>:"Write Key.vi"("section"=w1152, "error in (no error)"=w1186, "value"=w1142, "key"="泵滴定数5", "refnum"=w1185) -> ("error out"=w1147:errorcluster, "refnum out"=w1148:T14)  [unwired: 4 in, 1 out]
        n772 = local read "启用1"() -> (w1161:bool)
        n773 = call-poly <vilib>:"Write Key.vi"("section"=w1152, "error in (no error)"=w1147, "value"=w1161, "key"="启用1", "refnum"=w1148) -> ("error out"=w1157:errorcluster, "refnum out"=w1160:T14)  [unwired: 4 in, 1 out]
        n774 = local read "启用2"() -> (w1158:bool)
        n775 = call-poly <vilib>:"Write Key.vi"("section"=w1152, "error in (no error)"=w1157, "value"=w1158, "key"="启用2", "refnum"=w1160) -> ("error out"=w1168:errorcluster, "refnum out"=w1167:T14)  [unwired: 4 in, 1 out]
        n776 = local read "启用3"() -> (w1156:bool)
        n777 = call-poly <vilib>:"Write Key.vi"("section"=w1152, "error in (no error)"=w1168, "value"=w1156, "key"="启用3", "refnum"=w1167) -> ("error out"=w1166:errorcluster, "refnum out"=w1165:T14)  [unwired: 4 in, 1 out]
        n778 = local read "启用4"() -> (w1144:bool)
        n779 = call-poly <vilib>:"Write Key.vi"("section"=w1152, "error in (no error)"=w1166, "value"=w1144, "key"="启用4", "refnum"=w1165) -> ("error out"=w1164:errorcluster, "refnum out"=w1163:T14)  [unwired: 4 in, 1 out]
        n780 = local read "启用5"() -> (w1143:bool)
        n781 = call-poly <vilib>:"Write Key.vi"("section"=w1152, "error in (no error)"=w1164, "value"=w1143, "key"="启用5", "refnum"=w1163) -> ("error out"=w1145:errorcluster, "refnum out"=w1146:T14)  [unwired: 4 in, 1 out]
        n782 = call <vilib>:"Close Config Data.vi"("error in (no error)"=w1145, "refnum"=w1146) -> ()  [unwired: 8 in, 2 out]
      }
      event "关闭", "关闭 2", "关闭 3": Value Change {
        n783 = event-data() -> ()  [unwired: 1 in, 6 out]
        n784 = property on="窗格" class="Pane"("Origin"=T15 {"Horizontal"=0, "Vertical"=0} ("原点")) -> ()  [unwired: 2 in, 2 out]
      }
      event Application Instance Close {
        n785 = event-data() -> ()  [unwired: 1 in, 4 out]
      }
      event "时间校准": Value Change {
        n786 = event-data() -> ()  [unwired: 1 in, 6 out]
        n787 = Get Date/Time In Seconds() -> (seconds since 1Jan1904=w1215:timestamp)
        n788 = Build Array(w1215) -> (w1214:timestamp[])
        n789 = call "DateToHex.vi"("DATE"=w1214) -> ("数组"=w1212:u16[])  [unwired: 10 in]
        n790 = Insert Into Array(array=u16[] [1] ("values"), index=1 ("索引"), new element=w1212) -> (w1208:u16[])
        n791 = call "CODMnMB_api.vi"("STEP"=enum16{"open", "read", "write", "close"}."write", "values"=w1208, "starting address"=u16 4612) -> ("error out"=w1207:errorcluster)  [unwired: 5 in, 3 out]
        n792 = call <vilib>:"Clear Errors.vi"("error in (no error)"=w1207) -> ()  [unwired: 5 in, 2 out]
      }
      event "故障清除": Value Change {
        n793 = event-data() -> ()  [unwired: 1 in, 6 out]
        n794 = call "CODMnMB_api.vi"("STEP"=enum16{"open", "read", "write", "close"}."write", "values"=u16[] [1], "starting address"=u16 4611) -> ()  [unwired: 5 in, 4 out]
      }
      event "定时启动": Mouse Down {
        n795 = event-data() -> ()  [unwired: 1 in, 8 out]
        n796 = flat-sequence {
          frame #0 {
            n797 = global read "CODMn断电保存全局变量.vi" "定时控制"() -> (w1219:T9)
            n798 = call "周期设置.vi"("定时控制参数输入"=w1219) -> ("定时控制参数输出"=w1220:T9)  [unwired: 10 in]
            n799 = global write "CODMn断电保存全局变量.vi" "定时控制"(w1220) -> ()
          }
          frame #1 {
            n800 = call <vilib>:"Application Directory.vi"() -> ("Application Directory"=w1234:path)
            n801 = Build Path(base path=w1234, name or relative path="data\\sys.ini" ("名称或相对路径")) -> (appended path=w1232:path)
            n802 = call <vilib>:"Open Config Data.vi"("configuration file path"=w1232) -> ("error out"=w1228:errorcluster, "refnum"=w1231:T14)  [unwired: 8 in, 1 out]
            n803 = vi-ref "斯坦道CODMn.lvlib:CODMn断电保存全局变量.vi"() -> (w1230:refnum<vi>)
            n804 = call <userlib>:"Write Panel to INI__ogtk.vi"("error in (no error)"=w1228, "VI ref"=w1230, "refnum"=w1231) -> ("error out"=w1227:errorcluster, "refnum out"=w1229:T14)  [unwired: 7 in]
            n805 = call <vilib>:"Close Config Data.vi"("error in (no error)"=w1227, "refnum"=w1229) -> ("error out"=w1222:errorcluster, "file path"=w1221:path)  [unwired: 8 in]
            n806 = Open/Create/Replace File(file path (use dialog)=w1221, error in=w1222) -> (refnum out=w1225:refnum<file>, error out=w1226:errorcluster)  [unwired: 4 in, 1 out]
            n807 = Flush File(refnum=w1225, error in=w1226) -> (refnum out=w1224:refnum<file>, error out=w1223:errorcluster)
            n808 = Close File(refnum=w1224, error in=w1223) -> ()  [unwired: 2 out]
          }
        }
      }
      event "测量模式(公式)": Value Change {
        n809 = event-data() -> ()  [unwired: 1 in, 6 out]
        n810 = flat-sequence {
          frame #0 {
            n811 = global write "CODMn断电保存全局变量.vi" "测量模式(公式)"("测量模式(公式)") -> ()
          }
          frame #1 {
            n812 = call <vilib>:"Application Directory.vi"() -> ("Application Directory"=w1249:path)
            n813 = Build Path(base path=w1249, name or relative path="data\\sys.ini" ("名称或相对路径")) -> (appended path=w1247:path)
            n814 = call <vilib>:"Open Config Data.vi"("configuration file path"=w1247) -> ("error out"=w1243:errorcluster, "refnum"=w1246:T14)  [unwired: 8 in, 1 out]
            n815 = vi-ref "斯坦道CODMn.lvlib:CODMn断电保存全局变量.vi"() -> (w1245:refnum<vi>)
            n816 = call <userlib>:"Write Panel to INI__ogtk.vi"("error in (no error)"=w1243, "VI ref"=w1245, "refnum"=w1246) -> ("error out"=w1242:errorcluster, "refnum out"=w1244:T14)  [unwired: 7 in]
            n817 = call <vilib>:"Close Config Data.vi"("error in (no error)"=w1242, "refnum"=w1244) -> ("error out"=w1237:errorcluster, "file path"=w1236:path)  [unwired: 8 in]
            n818 = Open/Create/Replace File(file path (use dialog)=w1236, error in=w1237) -> (refnum out=w1240:refnum<file>, error out=w1241:errorcluster)  [unwired: 4 in, 1 out]
            n819 = Flush File(refnum=w1240, error in=w1241) -> (refnum out=w1239:refnum<file>, error out=w1238:errorcluster)
            n820 = Close File(refnum=w1239, error in=w1238) -> ()  [unwired: 2 out]
          }
        }
      }
      event "CODMn跨度量程选择": Value Change {
        n821 = event-data() -> ()  [unwired: 1 in, 6 out]
        n822 = flat-sequence {
          frame #0 {
            n823 = global write "CODMn断电保存全局变量.vi" "CODMn跨度量程选择"("CODMn跨度量程选择") -> ()
          }
          frame #1 {
            n824 = call <vilib>:"Application Directory.vi"() -> ("Application Directory"=w1264:path)
            n825 = Build Path(base path=w1264, name or relative path="data\\sys.ini" ("名称或相对路径")) -> (appended path=w1262:path)
            n826 = call <vilib>:"Open Config Data.vi"("configuration file path"=w1262) -> ("error out"=w1258:errorcluster, "refnum"=w1261:T14)  [unwired: 8 in, 1 out]
            n827 = vi-ref "斯坦道CODMn.lvlib:CODMn断电保存全局变量.vi"() -> (w1260:refnum<vi>)
            n828 = call <userlib>:"Write Panel to INI__ogtk.vi"("error in (no error)"=w1258, "VI ref"=w1260, "refnum"=w1261) -> ("error out"=w1257:errorcluster, "refnum out"=w1259:T14)  [unwired: 7 in]
            n829 = call <vilib>:"Close Config Data.vi"("error in (no error)"=w1257, "refnum"=w1259) -> ("error out"=w1252:errorcluster, "file path"=w1251:path)  [unwired: 8 in]
            n830 = Open/Create/Replace File(file path (use dialog)=w1251, error in=w1252) -> (refnum out=w1255:refnum<file>, error out=w1256:errorcluster)  [unwired: 4 in, 1 out]
            n831 = Flush File(refnum=w1255, error in=w1256) -> (refnum out=w1254:refnum<file>, error out=w1253:errorcluster)
            n832 = Close File(refnum=w1254, error in=w1253) -> ()  [unwired: 2 out]
          }
        }
      }
      event "CODMn零点核查选择": Value Change {
        n833 = event-data() -> ()  [unwired: 1 in, 6 out]
        n834 = global write "CODMn断电保存全局变量.vi" "CODMn零点核查选择"("CODMn零点核查选择") -> ()
      }
      event "校准1", "校准2", "校准3", "校准4", "校准5": Value Change {
        n835 = event-data() -> ()  [unwired: 1 in, 6 out]
        n836 = flat-sequence {
          frame #0 {
            n837 = Build Array("校准1", "校准2", "校准3", "校准4", "校准5") -> (w1268:bool[])
            n838 = for {
              tunnel: w1268 -> [w1279] mode=indexing
              i -> [w1272]
              n839 = case shown="4" w1272 {
                tunnel: ["浓度1" "浓度2" "浓度3" "浓度4" "浓度5"] -> w1275
                frame 0, Default {
                }
                frame 1 {
                }
                frame 2 {
                }
                frame 3 {
                }
                frame 4 {
                }
              }
              n840 = Multiply(x=w1275, y=100.0) -> (x*y=w1273:dbl)
              n841 = Insert Into Array(array=u16[] [] ("values"), index=0 ("索引"), new element=w1273) -> (w1276:u16[])
              n842 = case shown="真" w1279 {
                tunnel: w1276 -> [_ w1286]
                tunnel: w1272 -> [_ w1289]
                frame False {
                }
                frame True {
                  n843 = Increment(x=w1289) -> (x+1=→"当前校准":i32)
                  n844 = call "CODMnMB_api.vi"("STEP"=enum16{"open", "read", "write", "close"}."write", "values"=w1286, "starting address"=u16 4274) -> ()  [unwired: 5 in, 4 out]
                }
              }
            }
          }
          frame #1 {
            n845 = local read "当前校准"() -> (w1296:i32)
            n846 = case shown="5" w1296 {
              tunnel: [w1300 w1301 w1302 w1303 w1304] -> w1295
              frame 1, Default {
                n847 = local read "浓度1"() -> (w1300:dbl)
              }
              frame 2 {
                n848 = local read "浓度2"() -> (w1301:dbl)
              }
              frame 3 {
                n849 = local read "浓度3"() -> (w1302:dbl)
              }
              frame 4 {
                n850 = local read "浓度4"() -> (w1303:dbl)
              }
              frame 5 {
                n851 = local read "浓度5"() -> (w1304:dbl)
              }
            }
            n852 = Not Equal To 0?(x=w1295) -> (x != 0?=w1293:bool)
            n853 = case shown="真" w1293 {
              tunnel: [u16 8 ("address") u16 9 ("address")] -> w1299
              tunnel: ["校零" ("测量模式") "校标" ("测量模式")] -> w1294
              frame False {
              }
              frame True {
              }
            }
            n854 = global write "COD测量模式全局.vi" "测量模式"(w1294) -> ()
            n855 = Insert Into Array(array=u16[] [] ("values"), index=0 ("索引"), new element=w1299) -> (w1290:u16[])
            n856 = call "CODMnMB_api.vi"("STEP"=enum16{"open", "read", "write", "close"}."write", "values"=w1290, "starting address"=u16 4608 ("address")) -> ()  [unwired: 5 in, 4 out]
          }
          frame #2 {
            n857 = local read "选用水样"() -> (w1311:enum16{"葡萄糖", "草酸钠"})
            n858 = local read "量程选择"() -> (w1310:enum16{"低量程", "高量程", "0-2量程"})
            n859 = case shown="\"葡萄糖\", 默认" w1311 {
              tunnel: ["葡萄糖标线" ("section") "草酸钠标线" ("section")] -> w1312
              frame "葡萄糖", Default {
              }
              frame "草酸钠" {
              }
            }
            n860 = case shown="\"0-2量程\"" w1310 {
              tunnel: ["低量程" "高量程" "0-2量程"] -> w1313
              frame "低量程", Default {
              }
              frame "高量程" {
              }
              frame "0-2量程" {
              }
            }
            n861 = call <vilib>:"Application Directory.vi"() -> ("Application Directory"=w1320:path)
            n862 = Concatenate Strings(w1312, w1313) -> (w1309:string)
            n863 = Build Path(base path=w1320, name or relative path="data\\Set.ini" ("名称或相对路径")) -> (appended path=w1322:path)
            n864 = local read "当前校准"() -> (w1316:i32)
            n865 = call <vilib>:"Open Config Data.vi"("configuration file path"=w1322) -> ("error out"=w1318:errorcluster, "refnum"=w1319:T14)  [unwired: 8 in, 1 out]
            n866 = call-poly <vilib>:"Write Key.vi"("section"=w1309, "error in (no error)"=w1318, "value"=w1316, "key"="当前选用的校准" ("section"), "refnum"=w1319) -> ("error out"=w1314:errorcluster, "refnum out"=w1315:T14)  [unwired: 4 in, 1 out]
            n867 = call <vilib>:"Close Config Data.vi"("error in (no error)"=w1314, "refnum"=w1315) -> ()  [unwired: 8 in, 2 out]
          }
        }
      }
      event "自动切换量程:", "低切高阈值:", "高切低阈值:": Value Change {
        n868 = event-data() -> ()  [unwired: 1 in, 6 out]
        n869 = flat-sequence {
          frame #0 {
            n870 = local read "自动切换量程:"() -> (w1330:enum16{"关闭", "自动切换测一次", "自动切换测两次"})
            n871 = local read "低切高阈值:"() -> (w1329:dbl)
            n872 = local read "高切低阈值:"() -> (w1328:dbl)
            n873 = global write "CODMn断电保存全局变量.vi" "自动切换量程:"(w1330) -> ()
            n874 = global write "CODMn断电保存全局变量.vi" "低切高阈值:"(w1329) -> ()
            n875 = global write "CODMn断电保存全局变量.vi" "高切低阈值:"(w1328) -> ()
          }
          frame #1 {
            n876 = call <vilib>:"Application Directory.vi"() -> ("Application Directory"=w1344:path)
            n877 = Build Path(base path=w1344, name or relative path="data\\sys.ini" ("名称或相对路径")) -> (appended path=w1342:path)
            n878 = call <vilib>:"Open Config Data.vi"("configuration file path"=w1342) -> ("error out"=w1338:errorcluster, "refnum"=w1341:T14)  [unwired: 8 in, 1 out]
            n879 = vi-ref "斯坦道CODMn.lvlib:CODMn断电保存全局变量.vi"() -> (w1340:refnum<vi>)
            n880 = call <userlib>:"Write Panel to INI__ogtk.vi"("error in (no error)"=w1338, "VI ref"=w1340, "refnum"=w1341) -> ("error out"=w1337:errorcluster, "refnum out"=w1339:T14)  [unwired: 7 in]
            n881 = call <vilib>:"Close Config Data.vi"("error in (no error)"=w1337, "refnum"=w1339) -> ("error out"=w1332:errorcluster, "file path"=w1331:path)  [unwired: 8 in]
            n882 = Open/Create/Replace File(file path (use dialog)=w1331, error in=w1332) -> (refnum out=w1335:refnum<file>, error out=w1336:errorcluster)  [unwired: 4 in, 1 out]
            n883 = Flush File(refnum=w1335, error in=w1336) -> (refnum out=w1334:refnum<file>, error out=w1333:errorcluster)
            n884 = Close File(refnum=w1334, error in=w1333) -> ()  [unwired: 2 out]
          }
        }
      }
      event "模型": Value Change {
        n885 = event-data() -> ()  [unwired: 1 in, 6 out]
        n886 = call <vilib>:"Application Directory.vi"() -> ("Application Directory"=w1354:path)
        n887 = Build Path(base path=w1354, name or relative path="data\\Set.ini" ("名称或相对路径")) -> (appended path=w1352:path)
        n888 = call <vilib>:"Open Config Data.vi"("configuration file path"=w1352) -> ("error out"=w1350:errorcluster, "refnum"=w1351:T14)  [unwired: 8 in, 1 out]
        n889 = local read "模型"() -> (w1345:enum32{"线性", "多项式"})
        n890 = call-poly <vilib>:"Write Key.vi"("section"="CODMn模型选择" ("key"), "error in (no error)"=w1350, "value"=w1345, "key"="线性和多项式", "refnum"=w1351) -> ("error out"=w1346:errorcluster, "refnum out"=w1347:T14)  [unwired: 4 in, 1 out]
        n891 = call <vilib>:"Close Config Data.vi"("error in (no error)"=w1346, "refnum"=w1347) -> ()  [unwired: 8 in, 2 out]
      }
      event "浓度1", "浓度2", "浓度3", "泵滴定数1", "泵滴定数2", "泵滴定数3", "启用1", "启用2", "启用3", "浓度4", "浓度5", "泵滴定数4", "泵滴定数5", "启用4", "启用5": Value Change {
        n892 = event-data() -> ()  [unwired: 1 in, 6 out]
        n893 = local read "选用水样"() -> (w1370:enum16{"葡萄糖", "草酸钠"})
        n894 = local read "量程选择"() -> (w1369:enum16{"低量程", "高量程", "0-2量程"})
        n895 = case shown="\"0-2量程\"" w1369 {
          tunnel: ["低量程" "高量程" "0-2量程"] -> w1367
          frame "低量程", Default {
          }
          frame "高量程" {
          }
          frame "0-2量程" {
          }
        }
        n896 = call <vilib>:"Application Directory.vi"() -> ("Application Directory"=w1429:path)
        n897 = case shown="\"葡萄糖\", 默认" w1370 {
          tunnel: ["葡萄糖标线" ("section") "草酸钠标线" ("section")] -> w1376
          frame "葡萄糖", Default {
          }
          frame "草酸钠" {
          }
        }
        n898 = Build Path(base path=w1429, name or relative path="data\\Set.ini" ("名称或相对路径")) -> (appended path=w1427:path)
        n899 = call <vilib>:"Open Config Data.vi"("configuration file path"=w1427) -> ("error out"=w1425:errorcluster, "refnum"=w1426:T14)  [unwired: 8 in, 1 out]
        n900 = local read "浓度1"() -> (w1423:dbl)
        n901 = Concatenate Strings(w1376, w1367) -> (w1368:string)
        n902 = local read "浓度2"() -> (w1407:dbl)
        n903 = call-poly <vilib>:"Write Key.vi"("section"=w1368, "error in (no error)"=w1425, "value"=w1423, "key"="浓度1", "refnum"=w1426) -> ("error out"=w1422:errorcluster, "refnum out"=w1421:T14)  [unwired: 4 in, 1 out]
        n904 = local read "浓度3"() -> (w1403:dbl)
        n905 = call-poly <vilib>:"Write Key.vi"("section"=w1368, "error in (no error)"=w1422, "value"=w1407, "key"="浓度2", "refnum"=w1421) -> ("error out"=w1420:errorcluster, "refnum out"=w1419:T14)  [unwired: 4 in, 1 out]
        n906 = local read "泵滴定数1"() -> (w1401:dbl)
        n907 = call-poly <vilib>:"Write Key.vi"("section"=w1368, "error in (no error)"=w1420, "value"=w1403, "key"="浓度3", "refnum"=w1419) -> ("error out"=w1418:errorcluster, "refnum out"=w1417:T14)  [unwired: 4 in, 1 out]
        n908 = call-poly <vilib>:"Write Key.vi"("section"=w1368, "error in (no error)"=w1418, "value"=w1401, "key"="泵滴定数1", "refnum"=w1417) -> ("error out"=w1416:errorcluster, "refnum out"=w1415:T14)  [unwired: 4 in, 1 out]
        n909 = local read "泵滴定数2"() -> (w1399:dbl)
        n910 = call-poly <vilib>:"Write Key.vi"("section"=w1368, "error in (no error)"=w1416, "value"=w1399, "key"="泵滴定数2", "refnum"=w1415) -> ("error out"=w1414:errorcluster, "refnum out"=w1413:T14)  [unwired: 4 in, 1 out]
        n911 = local read "泵滴定数3"() -> (w1397:dbl)
        n912 = local read "浓度4"() -> (w1366:dbl)
        n913 = call-poly <vilib>:"Write Key.vi"("section"=w1368, "error in (no error)"=w1414, "value"=w1397, "key"="泵滴定数3", "refnum"=w1413) -> ("error out"=w1412:errorcluster, "refnum out"=w1411:T14)  [unwired: 4 in, 1 out]
        n914 = local read "浓度5"() -> (w1365:dbl)
        n915 = call-poly <vilib>:"Write Key.vi"("section"=w1368, "error in (no error)"=w1412, "value"=w1366, "key"="浓度4", "refnum"=w1411) -> ("error out"=w1405:errorcluster, "refnum out"=w1406:T14)  [unwired: 4 in, 1 out]
        n916 = call-poly <vilib>:"Write Key.vi"("section"=w1368, "error in (no error)"=w1405, "value"=w1365, "key"="浓度5", "refnum"=w1406) -> ("error out"=w1363:errorcluster, "refnum out"=w1364:T14)  [unwired: 4 in, 1 out]
        n917 = local read "泵滴定数4"() -> (w1362:dbl)
        n918 = call-poly <vilib>:"Write Key.vi"("section"=w1368, "error in (no error)"=w1363, "value"=w1362, "key"="泵滴定数4", "refnum"=w1364) -> ("error out"=w1410:errorcluster, "refnum out"=w1409:T14)  [unwired: 4 in, 1 out]
        n919 = local read "泵滴定数5"() -> (w1361:dbl)
        n920 = call-poly <vilib>:"Write Key.vi"("section"=w1368, "error in (no error)"=w1410, "value"=w1361, "key"="泵滴定数5", "refnum"=w1409) -> ("error out"=w1359:errorcluster, "refnum out"=w1360:T14)  [unwired: 4 in, 1 out]
        n921 = local read "启用1"() -> (w1385:bool)
        n922 = call-poly <vilib>:"Write Key.vi"("section"=w1368, "error in (no error)"=w1359, "value"=w1385, "key"="启用1", "refnum"=w1360) -> ("error out"=w1381:errorcluster, "refnum out"=w1384:T14)  [unwired: 4 in, 1 out]
        n923 = local read "启用2"() -> (w1382:bool)
        n924 = call-poly <vilib>:"Write Key.vi"("section"=w1368, "error in (no error)"=w1381, "value"=w1382, "key"="启用2", "refnum"=w1384) -> ("error out"=w1392:errorcluster, "refnum out"=w1391:T14)  [unwired: 4 in, 1 out]
        n925 = local read "启用3"() -> (w1380:bool)
        n926 = call-poly <vilib>:"Write Key.vi"("section"=w1368, "error in (no error)"=w1392, "value"=w1380, "key"="启用3", "refnum"=w1391) -> ("error out"=w1390:errorcluster, "refnum out"=w1389:T14)  [unwired: 4 in, 1 out]
        n927 = local read "启用4"() -> (w1355:bool)
        n928 = call-poly <vilib>:"Write Key.vi"("section"=w1368, "error in (no error)"=w1390, "value"=w1355, "key"="启用4", "refnum"=w1389) -> ("error out"=w1388:errorcluster, "refnum out"=w1387:T14)  [unwired: 4 in, 1 out]
        n929 = local read "启用5"() -> (w1356:bool)
        n930 = call-poly <vilib>:"Write Key.vi"("section"=w1368, "error in (no error)"=w1388, "value"=w1356, "key"="启用5", "refnum"=w1387) -> ("error out"=w1357:errorcluster, "refnum out"=w1358:T14)  [unwired: 4 in, 1 out]
        n931 = local read "选用水样"() -> (w1375:enum16{"葡萄糖", "草酸钠"})
        n932 = call-poly <vilib>:"Write Key.vi"("section"="标线选择", "error in (no error)"=w1357, "value"=w1375, "key"="选用水样", "refnum"=w1358) -> ("error out"=w1372:errorcluster, "refnum out"=w1373:T14)  [unwired: 4 in, 1 out]
        n933 = call <vilib>:"Close Config Data.vi"("error in (no error)"=w1372, "refnum"=w1373) -> ()  [unwired: 8 in, 2 out]
      }
      event "读取": Value Change {
        (unwired) u16 94 ("number of holding registers")
        (unwired) u16 4616 ("starting address")
        n934 = event-data() -> ()  [unwired: 1 in, 6 out]
        n935 = Bundle By Name(cluster=cluster{"命令":string} {"命令"=""} ("元素"), "命令"="CODMn读取公式" ("名称（未命名）")) -> (w1435:cluster{"命令":string})
        n936 = Enqueue Element(queue=w1439, element=w1435, error in (no error)=w1438) -> ()  [unwired: 1 in, 3 out]
      }
      event "写入": Mouse Down {
        n937 = event-data() -> ()  [unwired: 1 in, 8 out]
        n938 = local read "模型"() -> (w1443:enum32{"线性", "多项式"})
        n939 = case shown="\"线性\", 默认" w1443 {
          tunnel: [w1445 w1488] -> w1441
          tunnel: [w1444 w1487] -> w1440
          frame "线性", Default {
            n940 = local read "测量模式(公式)"() -> (w1446:u16)
            n941 = case shown="1" w1446 {
              tunnel: [u16 4626 ("starting address") w1453 w1458 w1463 w1468 w1473 w1478 w1483] -> w1445
              frame 0, Default {
              }
              frame 1 {
                n942 = local read "量程选择"() -> (w1452:enum16{"低量程", "高量程", "0-2量程"})
                n943 = case shown="\"低量程\", 默认" w1452 {
                  tunnel: [u16 4626 ("starting address") u16 4632 ("starting address") u16 4638 ("starting address")] -> w1453
                  frame "低量程", Default {
                  }
                  frame "高量程" {
                  }
                  frame "0-2量程" {
                  }
                }
              }
              frame 2 {
                n944 = local read "量程选择"() -> (w1457:enum16{"低量程", "高量程", "0-2量程"})
                n945 = case shown="\"低量程\", 默认" w1457 {
                  tunnel: [u16 4638 ("starting address") u16 4644 ("starting address") u16 4638 ("starting address")] -> w1458
                  frame "低量程", Default {
                  }
                  frame "高量程" {
                  }
                  frame "0-2量程" {
                  }
                }
              }
              frame 3 {
                n946 = local read "量程选择"() -> (w1462:enum16{"低量程", "高量程", "0-2量程"})
                n947 = case shown="\"低量程\", 默认" w1462 {
                  tunnel: [u16 4650 ("starting address") u16 4656 ("starting address") u16 4638 ("starting address")] -> w1463
                  frame "低量程", Default {
                  }
                  frame "高量程" {
                  }
                  frame "0-2量程" {
                  }
                }
              }
              frame 4 {
                n948 = local read "量程选择"() -> (w1467:enum16{"低量程", "高量程", "0-2量程"})
                n949 = case shown="\"低量程\", 默认" w1467 {
                  tunnel: [u16 4662 ("starting address") u16 4668 ("starting address") u16 4638 ("starting address")] -> w1468
                  frame "低量程", Default {
                  }
                  frame "高量程" {
                  }
                  frame "0-2量程" {
                  }
                }
              }
              frame 5 {
                n950 = local read "量程选择"() -> (w1472:enum16{"低量程", "高量程", "0-2量程"})
                n951 = case shown="\"低量程\", 默认" w1472 {
                  tunnel: [u16 4674 ("starting address") u16 4680 ("starting address") u16 4638 ("starting address")] -> w1473
                  frame "低量程", Default {
                  }
                  frame "高量程" {
                  }
                  frame "0-2量程" {
                  }
                }
              }
              frame 6 {
                n952 = local read "量程选择"() -> (w1477:enum16{"低量程", "高量程", "0-2量程"})
                n953 = case shown="\"低量程\", 默认" w1477 {
                  tunnel: [u16 4686 ("starting address") u16 4692 ("starting address") u16 4638 ("starting address")] -> w1478
                  frame "低量程", Default {
                  }
                  frame "高量程" {
                  }
                  frame "0-2量程" {
                  }
                }
              }
              frame 7 {
                n954 = local read "量程选择"() -> (w1482:enum16{"低量程", "高量程", "0-2量程"})
                n955 = case shown="\"低量程\", 默认" w1482 {
                  tunnel: [u16 4698 ("starting address") u16 4704 ("starting address") u16 4638 ("starting address")] -> w1483
                  frame "低量程", Default {
                  }
                  frame "高量程" {
                  }
                  frame "0-2量程" {
                  }
                }
              }
            }
            n956 = local read "K"() -> (w1450:dbl)
            n957 = local read "b"() -> (w1449:dbl)
            n958 = Build Array(w1450, w1449, 0.0 ("元素")) -> (w1448:dbl[])
            n959 = call "浮点转CDAB整形cod.vi"("浮点数"=w1448) -> ("CDAB整形输出"=w1444:u16[])  [unwired: 10 in]
          }
          frame "多项式" {
            # "b,k,c"
            n960 = local read "测量模式(公式)"() -> (w1489:u16)
            n961 = case shown="1" w1489 {
              tunnel: [u16 4626 ("starting address") w1497 w1502 w1507 w1512 w1517 w1522 w1527] -> w1488
              frame 0, Default {
              }
              frame 1 {
                n962 = local read "量程选择"() -> (w1496:enum16{"低量程", "高量程", "0-2量程"})
                n963 = case shown="\"低量程\", 默认" w1496 {
                  tunnel: [u16 4626 ("starting address") u16 4632 ("starting address") u16 4638 ("starting address")] -> w1497
                  frame "低量程", Default {
                  }
                  frame "高量程" {
                  }
                  frame "0-2量程" {
                  }
                }
              }
              frame 2 {
                n964 = local read "量程选择"() -> (w1501:enum16{"低量程", "高量程", "0-2量程"})
                n965 = case shown="\"低量程\", 默认" w1501 {
                  tunnel: [u16 4638 ("starting address") u16 4644 ("starting address") u16 4638 ("starting address")] -> w1502
                  frame "低量程", Default {
                  }
                  frame "高量程" {
                  }
                  frame "0-2量程" {
                  }
                }
              }
              frame 3 {
                n966 = local read "量程选择"() -> (w1506:enum16{"低量程", "高量程", "0-2量程"})
                n967 = case shown="\"低量程\", 默认" w1506 {
                  tunnel: [u16 4650 ("starting address") u16 4656 ("starting address") u16 4638 ("starting address")] -> w1507
                  frame "低量程", Default {
                  }
                  frame "高量程" {
                  }
                  frame "0-2量程" {
                  }
                }
              }
              frame 4 {
                n968 = local read "量程选择"() -> (w1511:enum16{"低量程", "高量程", "0-2量程"})
                n969 = case shown="\"低量程\", 默认" w1511 {
                  tunnel: [u16 4662 ("starting address") u16 4668 ("starting address") u16 4638 ("starting address")] -> w1512
                  frame "低量程", Default {
                  }
                  frame "高量程" {
                  }
                  frame "0-2量程" {
                  }
                }
              }
              frame 5 {
                n970 = local read "量程选择"() -> (w1516:enum16{"低量程", "高量程", "0-2量程"})
                n971 = case shown="\"低量程\", 默认" w1516 {
                  tunnel: [u16 4674 ("starting address") u16 4680 ("starting address") u16 4638 ("starting address")] -> w1517
                  frame "低量程", Default {
                  }
                  frame "高量程" {
                  }
                  frame "0-2量程" {
                  }
                }
              }
              frame 6 {
                n972 = local read "量程选择"() -> (w1521:enum16{"低量程", "高量程", "0-2量程"})
                n973 = case shown="\"低量程\", 默认" w1521 {
                  tunnel: [u16 4686 ("starting address") u16 4692 ("starting address") u16 4638 ("starting address")] -> w1522
                  frame "低量程", Default {
                  }
                  frame "高量程" {
                  }
                  frame "0-2量程" {
                  }
                }
              }
              frame 7 {
                n974 = local read "量程选择"() -> (w1526:enum16{"低量程", "高量程", "0-2量程"})
                n975 = case shown="\"低量程\", 默认" w1526 {
                  tunnel: [u16 4698 ("starting address") u16 4704 ("starting address") u16 4638 ("starting address")] -> w1527
                  frame "低量程", Default {
                  }
                  frame "高量程" {
                  }
                  frame "0-2量程" {
                  }
                }
              }
            }
            n976 = local read "多项式系数1"() -> (w1494:dbl[])
            n977 = Index Array(array=w1494) -> (element #1=w1491:dbl, element #2=w1492:dbl, element #3=w1490:dbl)  [unwired: 3 in]
            n978 = Build Array(w1492, w1491, w1490) -> (w1493:dbl[])
            n979 = call "浮点转CDAB整形cod.vi"("浮点数"=w1493) -> ("CDAB整形输出"=w1487:u16[])  [unwired: 10 in]
          }
        }
        n980 = call "CODMnMB_api.vi"("STEP"=enum16{"open", "read", "write", "close"}."write", "values"=w1440, "starting address"=w1441) -> ()  [unwired: 5 in, 4 out]
      }
      event "一键写入": Value Change {
        n981 = event-data() -> ()  [unwired: 1 in, 6 out]
        n982 = local read "模型"() -> (w1531:enum32{"线性", "多项式"})
        n983 = case shown="\"线性\", 默认" w1531 {
          frame "线性", Default {
            n984 = property on="测量模式(公式)" class="Ring (严格)"() -> ("NumItems"=w1532:u32)  [unwired: 2 in, 2 out]
            n985 = for {
              N: w1532 -> [_]
              i -> [w1537]
              n986 = Increment(x=w1537) -> (x+1=w1536:i32)
              n987 = local read "K"() -> (w1541:dbl)
              n988 = case shown="1" w1536 {
                tunnel: [u16 4626 ("starting address") w1547 w1552 w1557 w1562 w1567 w1572 w1577] -> w1534
                frame 0, Default {
                }
                frame 1 {
                  n989 = local read "量程选择"() -> (w1546:enum16{"低量程", "高量程", "0-2量程"})
                  n990 = case shown="\"低量程\", 默认" w1546 {
                    tunnel: [u16 4626 ("starting address") u16 4632 ("starting address") u16 4638 ("starting address")] -> w1547
                    frame "低量程", Default {
                    }
                    frame "高量程" {
                    }
                    frame "0-2量程" {
                    }
                  }
                }
                frame 2 {
                  n991 = local read "量程选择"() -> (w1551:enum16{"低量程", "高量程", "0-2量程"})
                  n992 = case shown="\"低量程\", 默认" w1551 {
                    tunnel: [u16 4638 ("starting address") u16 4644 ("starting address") u16 4638 ("starting address")] -> w1552
                    frame "低量程", Default {
                    }
                    frame "高量程" {
                    }
                    frame "0-2量程" {
                    }
                  }
                }
                frame 3 {
                  n993 = local read "量程选择"() -> (w1556:enum16{"低量程", "高量程", "0-2量程"})
                  n994 = case shown="\"低量程\", 默认" w1556 {
                    tunnel: [u16 4650 ("starting address") u16 4656 ("starting address") u16 4638 ("starting address")] -> w1557
                    frame "低量程", Default {
                    }
                    frame "高量程" {
                    }
                    frame "0-2量程" {
                    }
                  }
                }
                frame 4 {
                  n995 = local read "量程选择"() -> (w1561:enum16{"低量程", "高量程", "0-2量程"})
                  n996 = case shown="\"高量程\"" w1561 {
                    tunnel: [u16 4662 ("starting address") u16 4668 ("starting address") u16 4638 ("starting address")] -> w1562
                    frame "低量程", Default {
                    }
                    frame "高量程" {
                    }
                    frame "0-2量程" {
                    }
                  }
                }
                frame 5 {
                  n997 = local read "量程选择"() -> (w1566:enum16{"低量程", "高量程", "0-2量程"})
                  n998 = case shown="\"低量程\", 默认" w1566 {
                    tunnel: [u16 4674 ("starting address") u16 4680 ("starting address") u16 4638 ("starting address")] -> w1567
                    frame "低量程", Default {
                    }
                    frame "高量程" {
                    }
                    frame "0-2量程" {
                    }
                  }
                }
                frame 6 {
                  n999 = local read "量程选择"() -> (w1571:enum16{"低量程", "高量程", "0-2量程"})
                  n1000 = case shown="\"低量程\", 默认" w1571 {
                    tunnel: [u16 4686 ("starting address") u16 4692 ("starting address") u16 4638 ("starting address")] -> w1572
                    frame "低量程", Default {
                    }
                    frame "高量程" {
                    }
                    frame "0-2量程" {
                    }
                  }
                }
                frame 7 {
                  n1001 = local read "量程选择"() -> (w1576:enum16{"低量程", "高量程", "0-2量程"})
                  n1002 = case shown="\"低量程\", 默认" w1576 {
                    tunnel: [u16 4698 ("starting address") u16 4704 ("starting address") u16 4638 ("starting address")] -> w1577
                    frame "低量程", Default {
                    }
                    frame "高量程" {
                    }
                    frame "0-2量程" {
                    }
                  }
                }
              }
              n1003 = local read "b"() -> (w1542:dbl)
              n1004 = Build Array(w1541, w1542, 0.0 ("元素")) -> (w1543:dbl[])
              n1005 = call "浮点转CDAB整形cod.vi"("浮点数"=w1543) -> ("CDAB整形输出"=w1540:u16[])  [unwired: 10 in]
              n1006 = Insert Into Array(array=u16[] [], index=0 ("索引"), new element=w1540) -> (w1533:u16[])
              n1007 = call "CODMnMB_api.vi"("STEP"=enum16{"open", "read", "write", "close"}."write", "values"=w1533, "starting address"=w1534) -> ()  [unwired: 5 in, 4 out]
            }
          }
          frame "多项式" {
            # "b,k,c"
            n1008 = property on="测量模式(公式)" class="Ring (严格)"() -> ("NumItems"=w1581:u32)  [unwired: 2 in, 2 out]
            n1009 = for {
              N: w1581 -> [_]
              i -> [w1586]
              n1010 = local read "多项式系数1"() -> (w1590:dbl[])
              n1011 = Increment(x=w1586) -> (x+1=w1585:i32)
              n1012 = case shown="2" w1585 {
                tunnel: [u16 4626 ("starting address") w1597 w1602 w1607 w1612 w1617 w1622 w1627] -> w1582
                frame 0, Default {
                }
                frame 1 {
                  n1013 = local read "量程选择"() -> (w1596:enum16{"低量程", "高量程", "0-2量程"})
                  n1014 = case shown="\"低量程\", 默认" w1596 {
                    tunnel: [u16 4626 ("starting address") u16 4632 ("starting address") u16 4638 ("starting address")] -> w1597
                    frame "低量程", Default {
                    }
                    frame "高量程" {
                    }
                    frame "0-2量程" {
                    }
                  }
                }
                frame 2 {
                  n1015 = local read "量程选择"() -> (w1601:enum16{"低量程", "高量程", "0-2量程"})
                  n1016 = case shown="\"低量程\", 默认" w1601 {
                    tunnel: [u16 4638 ("starting address") u16 4644 ("starting address") u16 4638 ("starting address")] -> w1602
                    frame "低量程", Default {
                    }
                    frame "高量程" {
                    }
                    frame "0-2量程" {
                    }
                  }
                }
                frame 3 {
                  n1017 = local read "量程选择"() -> (w1606:enum16{"低量程", "高量程", "0-2量程"})
                  n1018 = case shown="\"低量程\", 默认" w1606 {
                    tunnel: [u16 4650 ("starting address") u16 4656 ("starting address") u16 4638 ("starting address")] -> w1607
                    frame "低量程", Default {
                    }
                    frame "高量程" {
                    }
                    frame "0-2量程" {
                    }
                  }
                }
                frame 4 {
                  n1019 = local read "量程选择"() -> (w1611:enum16{"低量程", "高量程", "0-2量程"})
                  n1020 = case shown="\"低量程\", 默认" w1611 {
                    tunnel: [u16 4662 ("starting address") u16 4668 ("starting address") u16 4638 ("starting address")] -> w1612
                    frame "低量程", Default {
                    }
                    frame "高量程" {
                    }
                    frame "0-2量程" {
                    }
                  }
                }
                frame 5 {
                  n1021 = local read "量程选择"() -> (w1616:enum16{"低量程", "高量程", "0-2量程"})
                  n1022 = case shown="\"低量程\", 默认" w1616 {
                    tunnel: [u16 4674 ("starting address") u16 4680 ("starting address") u16 4638 ("starting address")] -> w1617
                    frame "低量程", Default {
                    }
                    frame "高量程" {
                    }
                    frame "0-2量程" {
                    }
                  }
                }
                frame 6 {
                  n1023 = local read "量程选择"() -> (w1621:enum16{"低量程", "高量程", "0-2量程"})
                  n1024 = case shown="\"低量程\", 默认" w1621 {
                    tunnel: [u16 4686 ("starting address") u16 4692 ("starting address") u16 4638 ("starting address")] -> w1622
                    frame "低量程", Default {
                    }
                    frame "高量程" {
                    }
                    frame "0-2量程" {
                    }
                  }
                }
                frame 7 {
                  n1025 = local read "量程选择"() -> (w1626:enum16{"低量程", "高量程", "0-2量程"})
                  n1026 = case shown="\"低量程\", 默认" w1626 {
                    tunnel: [u16 4698 ("starting address") u16 4704 ("starting address") u16 4638 ("starting address")] -> w1627
                    frame "低量程", Default {
                    }
                    frame "高量程" {
                    }
                    frame "0-2量程" {
                    }
                  }
                }
              }
              n1027 = Index Array(array=w1590) -> (element #1=w1593:dbl, element #2=w1592:dbl, element #3=w1594:dbl)  [unwired: 3 in]
              n1028 = Build Array(w1592, w1593, w1594) -> (w1591:dbl[])
              n1029 = call "浮点转CDAB整形cod.vi"("浮点数"=w1591) -> ("CDAB整形输出"=w1589:u16[])  [unwired: 10 in]
              n1030 = Insert Into Array(array=u16[] [], index=0 ("索引"), new element=w1589) -> (w1583:u16[])
              n1031 = call "CODMnMB_api.vi"("STEP"=enum16{"open", "read", "write", "close"}."write", "values"=w1583, "starting address"=w1582) -> ()  [unwired: 5 in, 4 out]
            }
          }
        }
      }
      event "滴定曲线": Value Change {
        n1032 = event-data() -> ()  [unwired: 1 in, 6 out]
        n1033 = property on="窗格" class="Pane"("Origin"=T15 {"Horizontal"=0, "Vertical"=3200} ("原点")) -> ()  [unwired: 2 in, 2 out]
      }
      event "历史波形": Value Change {
        n1034 = event-data() -> ()  [unwired: 1 in, 6 out]
        n1035 = call-poly <vilib>:"Read Waveforms from File.vi"() -> ("error out"=w1632:errorcluster, "first waveform in record"=w1633:waveform(dbl))  [unwired: 6 in, 2 out]
        n1036 = case shown="无错误" w1632 {
          tunnel: w1633 -> [w1636 _]
          frame No Error {
            n1037 = Unbundle By Name(w1636) -> ("t0"=→"波形时间":timestamp, "Y"=w1635:dbl[])  [unwired: 2 out]
            n1038 = local write "滴定数-ORP值"(w1635) -> ()
            n1039 = local write "ORP滴定曲线"(w1635) -> ()
          }
          frame Error {
            n1040 = One Button Dialog(message="打开失败" ("消息")) -> ()  [unwired: 1 in, 1 out]
          }
        }
      }
      event "释放串口": Value Change {
        n1041 = event-data() -> ()  [unwired: 1 in, 6 out]
        n1042 = Two Button Dialog(message="确认是否释放串口，释放串口将导致通信失败！" ("消息")) -> (T button?=w1638:bool)  [unwired: 2 in]
        n1043 = case shown="真" w1638 {
          tunnel: w1641 -> [_ w1643]
          tunnel: w1640 -> [_ w1642]
          frame False {
          }
          frame True {
            n1044 = Bundle By Name(cluster=cluster{"命令":string} {"命令"=""} ("元素"), "命令"="停用模块" ("名称（未命名）")) -> (w1644:cluster{"命令":string})
            n1045 = Enqueue Element(queue=w1643, element=w1644, error in (no error)=w1642) -> ()  [unwired: 1 in, 3 out]
          }
        }
      }
      event "打开串口": Value Change {
        n1046 = event-data() -> ()  [unwired: 1 in, 6 out]
        n1047 = global read "CODMn断电保存全局变量.vi" "VISA resource name"() -> (w1651:refnum<visa-resource-name>)
        n1048 = call "串口配置.vi"("VISA资源名称"=w1651) -> ("确认 2"=w1649:bool, "VISA资源名称 2"=w1650:refnum<visa-resource-name>)  [unwired: 9 in]
        n1049 = case shown="真" w1649 {
          tunnel: w1650 -> [_ w1657]
          tunnel: w1648 -> [_ w1653]
          tunnel: w1647 -> [_ w1652]
          frame False {
          }
          frame True {
            n1050 = global write "CODMn断电保存全局变量.vi" "VISA resource name"(w1657) -> ()
            n1051 = Bundle By Name(cluster=cluster{"命令":string} {"命令"=""} ("元素"), "命令"="启用模块" ("名称（未命名）")) -> (w1654:cluster{"命令":string})
            n1052 = Enqueue Element(queue=w1653, element=w1654, error in (no error)=w1652) -> ()  [unwired: 1 in, 3 out]
          }
        }
      }
      event Timeout {
        n1053 = event-data() -> ()  [unwired: 1 in, 3 out]
      }
    }
  }
  n1054 = while {
    tunnel: w12 -> [w1667]
    tunnel: w11 -> [w1666]
    tunnel: w3 -> [_]
    stop <- FALSE stop-if-true
    # "主循环界面显示"
    n1055 = flat-sequence {
      frame #0 {
        # "测量状态显示"
        n1056 = global read "COD读取DATA全局.vi" "测量状态"() -> (w1701:u16[])
        n1057 = To Word Integer(number=w1701) -> (16bit integer=w1712:i16[])
        n1058 = Index Array(array=w1712, index #1=0 ("索引"), index #4=3 ("索引"), index #14=13 ("索引"), index #15=14 ("索引"), index #21=20 ("索引"), index #32=31 ("索引")) -> (element #1=w1717:i16, element #2=w1716:i16, element #3=w1715:i16, element #4=→"CODMn工作状态":i16, element #5=→"模式（受控）":i16, element #6=→"进样管":i16, element #7=→"高锰酸钾":i16, element #8=→"草酸钠":i16, element #9=→"硫酸":i16, element #10=w1711:i16, element #11=w1732:i16, element #12=w1707:i16, element #13=→"报警数字":i16, element #14=w1738:i16, element #15=w1723:i16, element #16=→"多列列表框":i16, element #21=w1699:i16, element #33=→"分":i16, element #34=→"秒":i16)  [unwired: 28 in, 15 out]
        n1059 = Number To Decimal String(number=w1699) -> (decimal integer string=→"基本量程(显示)":string)  [unwired: 1 in]
        n1060 = local write "基本量程"(w1699) -> ()
        n1061 = Build Array(w1717, w1716, w1715) -> (w1718:i16[])
        n1062 = To Single Precision Float(number=w1711) -> (single precision float=→"ORP显示":sgl)
        n1063 = call "HexToDate.vi"("数组"=w1718) -> ("DATE"=w1713:timestamp[])  [unwired: 10 in]
        n1064 = Index Array(array=w1713) -> (element=→"仪器时间":timestamp)  [unwired: 1 in]
        n1065 = Divide(x=w1732, y=u16 10) -> (x/y=→"温度":dbl)
        n1066 = Divide(x=w1723, y=u16 1000) -> (x/y=→"标度滴定值":dbl)
        n1067 = Equal?(x=w1707, y=u16 2) -> (x = y?=→"断电排液标记":bool)
        n1068 = Equal?(x=w1707, y=u16 1) -> (x = y?=→"排液标记":bool)
        n1069 = Divide(x=w1738, y=u16 1000) -> (x/y=→"零点滴定值":dbl)
      }
    }
    n1070 = flat-sequence {
      frame #0 {
        # "工作状态显示"
        n1071 = local read "CODMn工作状态"() -> (w1676:T1)
        n1072 = Equal?(x=w1676, y=u16 0) -> (x = y?=→"待机":bool)
        n1073 = Equal?(x=w1676, y=u16 8) -> (x = y?=→"校零标记":bool)
        n1074 = Equal?(x=w1676, y=u16 9) -> (x = y?=→"校标标记":bool)
        n1075 = Equal?(x=w1676, y=u16 1) -> (x = y?=→"水样测量":bool)
        n1076 = Equal?(x=w1676, y=u16 7) -> (x = y?=→"质控样测量":bool)
        n1077 = Equal?(x=w1676, y=u16 10) -> (x = y?=→"加标回收测量":bool)
        n1078 = Equal?(x=w1676, y=u16 2) -> (x = y?=→"标样核查标记":bool)
        n1079 = Equal?(x=w1676, y=u16 6) -> (x = y?=→"平行样测量":bool)
        n1080 = Equal?(x=w1676, y=u16 3) -> (x = y?=→"零点核查标记":bool)
        n1081 = Equal?(x=w1676, y=u16 4) -> (x = y?=→"跨度核查标记":bool)
        n1082 = Equal?(x=w1676, y=u16 5) -> (x = y?=→"空白测试标记":bool)
      }
    }
    n1083 = First Call?() -> (First Call?: T/F=w1665:bool)
    n1084 = case shown="真" w1665 {
      tunnel: w1667 -> [w1766 w1771]
      tunnel: w1666 -> [w1765 w1770]
      tunnel: [w1766 w1769] -> w1663
      tunnel: [w1765 w1768] -> w1662
      frame False {
      }
      frame True {
        n1085 = Bundle By Name(cluster=cluster{"命令":string} {"命令"=""} ("元素"), "命令"="CODMn读取参数" ("名称（未命名）")) -> (w1774:cluster{"命令":string})
        n1086 = Enqueue Element(queue=w1771, element=w1774, timeout in ms (-1)=1000 ("超时毫秒(-1)"), error in (no error)=w1770) -> (queue out=w1769:refnum<queue>, error out=w1768:errorcluster)  [unwired: 1 out]
      }
    }
    n1087 = Wait (ms)(milliseconds to wait=u32 1000 ("等待时间（毫秒）")) -> ()  [unwired: 1 out]
    n1088 = Get Queue Status(queue=w1663, error in (no error)=w1662) -> (queue out=w1659:refnum<queue>, error out=w1658:errorcluster, # elements in queue=w1661:i32)  [unwired: 1 in, 5 out]
    n1089 = Equal To 0?(x=w1661) -> (x = 0?=w1660:bool)
    n1090 = flat-sequence {
      frame #0 {
        # "CODMn读取状态"
        n1091 = global read "COD读取DATA全局.vi" "M输出点"() -> (w1785:bool[])
        n1092 = global read "COD读取DATA全局.vi" "温度"() -> (w1786:bool[])
        n1093 = Index Array(array=w1786) -> (element=→"加热":bool)  [unwired: 1 in]
        n1094 = Index Array(array=w1785) -> (element #1=→"搅拌":bool, element #4=→"进水样":bool, element #5=→"进蒸馏水":bool, element #6=→"进标液":bool, element #7=→"进质控样":bool, element #8=→"进加标回收样":bool, element #9=→"进高锰酸钾":bool, element #10=→"进草酸钠":bool, element #11=→"进硫酸":bool)  [unwired: 11 in, 2 out]
      }
    }
    n1095 = case shown="真" w1660 {
      tunnel: w1659 -> [_ w1671]
      tunnel: w1658 -> [_ w1670]
      frame False {
      }
      frame True {
        n1096 = Bundle By Name(cluster=cluster{"命令":string} {"命令"=""} ("元素"), "命令"="CODMn读取" ("名称（未命名）")) -> (w1673:cluster{"命令":string})
        n1097 = Enqueue Element(queue=w1671, element=w1673, timeout in ms (-1)=1000 ("超时毫秒(-1)"), error in (no error)=w1670) -> ()  [unwired: 3 out]
      }
    }
    n1098 = Get Date/Time In Seconds() -> (seconds since 1Jan1904=→"系统时间":timestamp)
    n1099 = flat-sequence {
      frame #0 {
        # "A，B，K"
        # "CODMn读取状态"
        n1100 = global read "COD读取DATA全局.vi" "ORP、时间"() -> (w1789:u16[])
        n1101 = To Word Integer(number=w1789) -> (16bit integer=w1810:i16[])
        n1102 = Split 1D Array(array=w1810, index=3 ("索引")) -> (first subarray=w1791:i16[], second subarray=w1809:i16[])
        n1103 = Index Array(array=w1791) -> (element #1=w1795:i16, element #2=w1794:i16, element #3=w1793:i16)  [unwired: 3 in]
        n1104 = Index Array(array=w1809) -> (element #1=w1804:i16, element #2=w1808:i16, element #3=w1807:i16, element #4=w1806:i16)  [unwired: 4 in]
        n1105 = Build Array(w1795, w1794, w1793) -> (w1792:i16[])
        n1106 = To Single Precision Float(number=w1807) -> (single precision float=w1798:sgl)
        n1107 = To Single Precision Float(number=w1804) -> (single precision float=w1803:sgl)
        n1108 = To Single Precision Float(number=w1808) -> (single precision float=w1802:sgl)
        n1109 = To Single Precision Float(number=w1806) -> (single precision float=w1797:sgl)
        n1110 = call "HexToDate.vi"("数组"=w1792) -> ("DATE"=w1796:timestamp[])  [unwired: 10 in]
        n1111 = Divide(x=w1803, y=sgl 100.0) -> (x/y=→"COD浓度（mg/L)":sgl)
        n1112 = Index Array(array=w1796) -> (element=w1790:timestamp)  [unwired: 1 in]
        n1113 = Number To Decimal String(number=w1802) -> (decimal integer string=→"ORP-A":string)  [unwired: 1 in]
        n1114 = Number To Decimal String(number=w1798) -> (decimal integer string=→"ORP-B":string)  [unwired: 1 in]
        n1115 = Number To Decimal String(number=w1797) -> (decimal integer string=→"ORP-K":string)  [unwired: 1 in]
        n1116 = Format Date/Time String(seconds (now)=w1790) -> (date/time string=→"数据时间":string)  [unwired: 2 in]
      }
    }
    n1117 = flat-sequence {
      frame #0 {
        # "报警状态显示"
        n1118 = local read "报警数字"() -> (w1741:i16)
        n1119 = Equal?(x=w1741, y=u16 9) -> (x = y?=w1744:bool)
        "进水样超量程" <- w1744
        n1120 = Equal?(x=w1741, y=u16 10) -> (x = y?=w1743:bool)
        "排液故障" <- w1743
        n1121 = Equal?(x=w1741, y=u16 2) -> (x = y?=w1751:bool)
        "温控器故障" <- w1751
        n1122 = Equal?(x=w1741, y=u16 3) -> (x = y?=w1750:bool)
        "加热故障" <- w1750
        n1123 = Equal?(x=w1741, y=u16 4) -> (x = y?=w1749:bool)
        "高锰酸钾报警" <- w1749
        n1124 = Equal?(x=w1741, y=u16 5) -> (x = y?=w1748:bool)
        "草酸钠报警" <- w1748
        n1125 = Equal?(x=w1741, y=u16 6) -> (x = y?=w1747:bool)
        "测量错误" <- w1747
        n1126 = Equal?(x=w1741, y=u16 8) -> (x = y?=w1746:bool)
        "校零错误" <- w1746
        n1127 = Equal?(x=w1741, y=u16 7) -> (x = y?=w1745:bool)
        "校标错误" <- w1745
        n1128 = Equal?(x=w1741, y=u16 1) -> (x = y?=w1752:bool)
        "ORP故障" <- w1752
        n1129 = Compound Arithmetic op=OR ("复合运算")(w1752, w1751, w1750, w1749, w1748, w1747, w1745, w1746, w1744, w1743) -> (→"故障标记":bool)
        n1130 = Bundle By Name(cluster=T3 {"ORP故障"=FALSE, "温控器故障"=FALSE, "加热故障"=FALSE, "高锰酸钾报警"=FALSE, "草酸钠报警"=FALSE, "测量错误"=FALSE, "校零错误"=FALSE, "校标错误"=FALSE, " 进水样超量程"=FALSE, "排液阀故障"=FALSE} ("报警簇"), "ORP故障"=w1752, "温控器故障"=w1751, "加热故障"=w1750, "高锰酸钾报警"=w1749, "草酸钠报警"=w1748, "测量错误"=w1747, "校零错误"=w1746, "校标错误"=w1745, "进水样超量程"=w1744, "排液阀故障"=w1743) -> (→"报警簇":T3)
      }
    }
  }
  n1131 = disable-structure shown="禁用" {
    frame Disabled {
      n1132 = call "单步启动选择对话框.vi"() -> ("启动选择2"=w1815:u16)  [unwired: 10 in, 1 out]
      n1133 = case shown="0" w1815 {
        tunnel: [u16 4610 ("address") u16 4610 ("address") u16 4610 ("address") u16 4610 ("address") u16 4610 ("address") u16 4610 ("address") u16 4610 ("address") u16 4610 ("address") u16 4610 ("address") u16 4610 ("address") u16 4610 ("address") u16 4610 ("address") u16 4610 ("address")] -> w1817
        tunnel: [u16 1 ("address") u16 2 ("address") u16 3 ("address") u16 4 ("address") u16 5 ("address") u16 6 ("address") u16 7 ("address") u16 8 ("address") u16 9 ("holding register value") u16 10 ("holding register value") u16 11 ("holding register value") u16 12 ("address") u16 0 ("address")] -> w1814
        frame 0 {
        }
        frame 1 {
        }
        frame 2 {
        }
        frame 3 {
        }
        frame 4 {
        }
        frame 5 {
        }
        frame 6 {
        }
        frame 7 {
        }
        frame 8 {
        }
        frame 9 {
        }
        frame 10 {
        }
        frame 11 {
        }
        frame 12, Default {
        }
      }
      n1134 = Insert Into Array(array=u16[] [] ("values"), index=0 ("索引"), new element=w1814) -> (w1818:u16[])
      n1135 = call "CODMnMB_api.vi"("STEP"=enum16{"open", "read", "write", "close"}."write", "values"=w1818, "starting address"=w1817) -> ()  [unwired: 5 in, 4 out]
    }
    frame Enabled {
    }
  }
